vi "ArgosUltimateEditionV2.vi"(0 "PID 1 COM":refnum<visa-resource-name>="COM24", 1 "Setpoint\n START":bool, 2 "Write to File":bool, 3 "SP 1 input (°C)":dbl=10.0 min=0.0 max=1300.0, 4 "Intervall (s)":u32=1 max=600, 5 "Write/\nRead":bool=TRUE, 6 "Delay (ms)":u32=500 min=100 max=600000, 7 "Auto Tune":bool, 9 "Standby":bool, 11 "Reset\nSTOP":bool, 12 "ON":bool=TRUE caption="OFF", 13 "Get Values":bool, 15 "File Path":path) -> (8 "(°C)":dbl format="%#.3f", 14 "SP 1 is (°C)":dbl)   [LabVIEW 2013]
doc: "1. Verwendung\n\nDas Programm dient der Steuerung und Abfrage des Thermocontrollers I3252 und dem Auslesen von zwei VC 840 Messgeräten und einem Druckmessgerät Pfeiffer Single Gauge. \nDie Messgeräte werden Standardmäßig ausgelesen und erst nach Betätigung des Schalters \"Write to File\" in einer Textdatei abgespeichert. Das Eingabefeld \"Intervall\" legt den Abstand der Messpunkte fest.\nDer Setpoint für den Thermocontroller wird erst nach Betätigung des Tasters \"Setpoint START\" übernommen und angesteuert. Er wird ind den EEPROM des Gerätes geschrieben. Die Regelung kann mit Hilfe des Schalters \"Standby\" unterbrochen werden. Durch den Taster \"Reset STOPP\" kann der Setpoint aus dem EEPROM gelöscht werden.\nDie Eingabeflächen \"Constant\" und \"Thickness\" dienen der Berechnung des spezifischen Widerstands.\nDie Eingabeflächen \"User\" und \"Sample\" werden in den Header der Textdatei übernommen.\nDer Indikator \"File Path\" zeigt den aktuellen Speicherort der Textdatei an. Dieser wird nach ausschalten des Schalters \"Write to File\" gelöscht. Bei erneuten Schreiben muss ein neuer Speicherort gewählt werden. Bei Wahl desselben Speicherorts werden sämtliche bereits gespeicherte Daten gelöscht.\n\n\n2. Erläuterungen zum Blockdiagramm\n2.1 äußere Sequenz\nDie äußerte Sequenz besteht aus fünf Frames. Der erste dient der Initialisierung der Ports. Der zweite dient als Verzögerung um dem Programm genug Zeit zu geben die Ports zu öffnen. Jedoch senden die beiden VC 840 bereits Informationen an den Computer die in einem Puffer zwischengespeichert werden. Im dritten Frame wird dieser Puffer geleert. Somit kommt es zu keinem Framing Error. Desweiteren wird in diesem Frame die Startzeit der Messungen genommen. Im vierten Frame wird die eigentliche Messung und Verarbeitung der Daten durchgeführt. Die while-Schleife wird nur durch Auftreten eines Fehlers oder durch Betätigung des Stopbuttons auf dem Front Panel in der oberen linken Ecke unterbrochen. Im fünften und letzten Frame werden die Ports wieder geschlossen und beim Auftreten eines Fehlers wird das Programm automatisch gestoppt. Falls kein Fehler auftritt wird die Sequenz von vorne abgearbeitet.\n\n2.2 while-Schleife und innere Sequenz\n2.2.1 \"Event Structure\"\n2.2.1.1 Allgemein\nDer erste Frame beinhaltet ein \"Event Structure\". Dieser reagiert auf insgesamt elf verschiedene Ereignisse. Falls keines dieser Ereignisse auftreten sollte, warte die Struktur eine Millisekunde bevor die \"Event Structure\" verlassen wird. Die übrigen Ereignisse treten ein, wenn der entsprechende Kontroller eine Werteänderung erfährt.\n\n2.2.1.2 Event: Setpoint\nDieser Case besteht von außen nach innen aus einer Stacked Sequence, einer for-Loop und einer Flat Sequence die wiederum zwei \"Case Structures\" enthält. Als erstes wird bei dem Schalter \"Setpoint START\" der Blinkmodus aktiviert und bei dem Schalter \"Read Temperature\" deaktiviert. Danach folgt das eigentliche setzen des Temperatursollwerts. In der ersten Iteration wird dem Controller I3252 ein Schreibbefehl gesendet. Theoretisch kann der Setpoint in den RAM oder in den EEPROM geschrieben werden. Diese Auswahl erfolgt mit Hilfe des Schalters \"RAM\". Da das Schreiben in den RAM -Speicher aber aus diversen Gründen nicht erwünscht ist, wurde es nicht implementiert. Eine nachträgliche Implementierung ist aber leicht möglich, in dem die untere String-Konstante \"*P012\" durch \"*W012\" ersetzt wird. An diesem Befehl wird eine fünfstellige Hexadezimalzahl angehängt, die den Sollwert wiedergibt. Der Sollwert wird vorher mit zehn multipliziert, da das Komma standardmäßig nach der ersten Ziffer festgesetzt wurde (Bsp.: 800 wird gesendet um 80 einzustellen). Dieser Befehlsstrang wird an das Gerät mittels des SubVIs \"Comm_Interface\", auf welches später noch näher eingegangen wird, weitergegeben. Der durch das Gerät zurückgegebene String wird nicht verarbeitet.\nDie zweite Iteration dient dem Auslesen des eingestellten Sollwertes. Wahlweise kann der RAM- oder der EEPROM-Speicher ausgelesen werden. Die eigentliche Verarbeitung des Ausgabestrings erfolgt durch das SubVI \"Edit Setpoint\".\nDie Implementierung zur Einstellung des zweiten Setpoints erfolgt durch kopieren der ersten beiden Fälle und ersetzen der \"1\" im Befehf durch eine \"2\" (Bsp.: \"*P012\" zu \"*P022\"). Es darf aber nicht vergessen werden, dass dann ebenfalls die Anzahl der Iterationen angepasst werden muss.\nAls letztes wird der Blinkmodus des Schalters \"Setpoint START\" wieder deaktiviert.\n\n2.2.1.3 Event: Standby\nDieses Ereignis aktiviert bzw. deaktiviert als erstes den Blinckmodus des entsprechenden Schalters und sendet danach den Befehl zum aktivieren (\"*D03\") oder zum deaktivieren (\"*E03\") des Standbymodus an den Thermocontroller.\n\n2.2.1.4 Event: Set Command \nDer in das Feld \"Command shall be\" eingegebene Befehl wird an den Thermocontroller übermittlet. Die korrekte Form des Befehls ist im \"Communication Manuel\" nachzuschlagen. Das \"*\"-Zeichen wurde allerdings schon implementiert und muss somit nicht mit eingegeben werden.\n\n2.2.1.5 Event: Reset\nIn der ersten Iteration wird der Reset-Befehl an den Thermocontroller gesendet. In Folge wird der gesamte EEPROM-Speicher gelöscht. Deshalb wird in der zweiten Iteration der Setpoint aktualisiert. Dieser Befehl hat keinen Einfluss auf den RAM-Speicher. Die anschließende Wartezeit ist auf vier Sekunden festgesetzt und wurde empirisch ermittelt. Diese Zeit benötigt das Gerät um den Reset durchzuführen und für die Kommunikation wieder zur Verfügung zu stehen.\n\n2.2.1.6 Event: Auto Tune\nEs ist festgeschrieben, dass der Setpoint für die \"Auto Tune\"-Funktion wenigstens 20°C über der aktuellen Temperatur liegt. Deshalb wird zunächst der aktuelle Temperaturwert ausgelesen. Im zweiten Schritt werden zu diesem Wert zwanzig addiert und der Setpoint wird in den RAM-Speicher geschrieben. Das Schreiben in diesen Speicher ist nötig, da die \"Auto Tune\"-Funktion\" erst nach einem Reset startet. Im dritten Schritt wird der eigentliche Befehl für den \"Auto Tune\" gesendet (siehe dazu \"Communication Manuel\" S.27). Als vierte und letzte Iteration der for-Schleife folgt der bereits erwähnte Reset-Befehl. Der Temperatursollwert, der im RAM-Speicher eingetragen ist, muss zum Schluss wieder auf 0°C gesetzt werden. Die Zeit für die Ausführung des \"Auto Tune\"-Befehls wurde empirisch ermittelt und 45 s festgesetzt.\n\n2.2.1.7 Event: Write LOW/HI\nDieses Ereignis setzt die am Analogausgang anliegende Spannung fest. Normalerweise beträgt dieser Spannungswert 0-10 V. Das angeschlossene Netzteil verträgt aber maximal nur 2,3 V. Aus diesem Grund wird der \"%HIGH\" auf 23 gesetzt. Somit beträgt die maximal anliegende Spannung nur noch 23% von der maximal möglichen, d.h 2,3V. Ein niedrigerer Wert ist jederzeit möglich, genauso wie ein höherer für den Parameter \"%LOW\". Diese werden zunächst nacheinander in den RAM-Speicher geschrieben und anschließend wieder ausgelesen.\n\n2.2.1.8 Event: Set PID\nDie Werte für den PID-Regler können sowohl mit Hilfe der \"Auto Tune\"-Funktion, als auch manuell eingestellt werden. Es wird wiederum zwischen dem Schreiben in den RAM- und dem EEPROM-Speicher unterschieden. Zunächst werden die Werte für \"P\", \"I\" und \"D\", in dieser Reihenfolge, gesetzt und danach die aktuellen Werte ausgelesen.\n\n2.2.1.9 Event: Get Values\nDieses Ereignis hat zur Folge, dass die Werte für \"P\", \"I\", \"D\", \"%LOW\", \"%HIGH\" und des Setpoints wahlweise aus dem RAM- oder EEPROM-Speicher gelesen werden. Die aktuellen Werte werden nicht nur in die entsprechenden Anzeigefelder übernommen, sondern auch in die entsprechenden Eingabefelder, mit Ausnahme des Temperatursollwerts. \n\n2.2.1.10 Event: RAM\nPrinzipiell kann zwischen dem Schreiben in den RAM- oder EEPROM-Speicher des Thermocontrollers gewählt werden. Die entsprechende Schalterposition auf dem Frontpanel zeigt den aktuell verwendeten Speicher an. Die Anzeigewerte werden bei jedem Umschalten aktualisiert und sind im entsprechenden Speicher eingetragen. Die Implementierung ist identisch mit der des Ereignisses \"Get Values\". Es gilt zu beachten, dass die Werte für \"%LOW\" und \"%HIGH\" nur in den RAM-Speicher geschrieben werden können und somit auch nur aus diesem ausgelesen werden können.\n\n2.2.1.11 Event: Set Gauge to Zero\nMit Hilfe der SubVIs \"Get Pressure\" und \"Offset Display\" werden die Werte für den alten und den neuen Offset und der durch den zweiten Drucksensor ermittelt Druck ermittelt. \n\n2.2.1.12 Event: Write to File\nSollte der Schalter \"Write to File\" aktiviert werden, d.h. Schalterposition oben, so wird zunächst durch das SubVI \"Header\" ein Header für die unter \"File Path\" definierte Datei angelegt. Alle Werte, die bereits in der entsprechenden Datei stehen, werden dabei gelöscht.\n\n2.2.2 \"Timed Structures\"\nIm dritten Frame der inneren Sequenz werden die Werte für Zeitpunkt, Temperatur, Spannung, Strom und Druck ermittelt. Damit die Werte zum gleichen Zeitpunkt aufgenommen werden, werden \"Timed Sequences\" eingesetzt. Mit dem entsprechenden Schalter auf dem Front Panel unter dem Tab \"Settings\" kann gewählt werden, ob das entsprechende Gerät ausgelesen werden soll oder nicht. Die einzelnen Sequenzen werden parallel abgearbeitet, womit die Prozesszeit von diesem Frame durch der zeitintensivsten Sequenz abhängt. Dies ist in aller Regel das Auslesen der Temperatur, da ein \"Delay\" von 500 ms oder größer benötigt wird, um den Controller ordentlich ansprechen zu können.\nDie Systemzeit wird durch das SubVI \"System Time in Seconds\" in Sekunden umgerechnet und der in dem Parameter \"Starttime\" gespeicherte Wert wird abgezogen. Somit werden die Sekunden seit dem Start des Programms gezählt.\n\n2.2.3 restlichen Frames\nIm zweiten Frame wird das Intervall zwischen den einzelnen Messwerten festgelegt. Dabei wird der Wert des Parameters \"Delay\" abgezogen. Dieser Wert beträgt im Normalfall 500 ms und ist somit nicht vernachlääsigbar.\nDer Vierte Frame beinhaltet die Umrechnung des Temperatur-Strings in einen Temperaturwert durch das SubVI \"Edit Tmperature\", die Berechnung des spezifischen Widerstands durch das SubVI \"Resistivity Calculation\" und die Überprüfung des Druckwerts. Auch werden die neu gewonnen Werte in das entsprechende Shift-Register übernommen. Falls der Druckwert einen in dem Parameter \"Pressure Limit (mbar)\" festgelegten Grenzwert überschreiten sollte, wird der Thermocontroller automatisch in den Standby-Modus versetzt. Des Weiteren wird der Schalter \"Standby\" solange gesperrt, wie der Druck oberhalb des Grenzwertes liegt. Wenn der Druck wieder unter den Grenzwert gesunken ist, wird der Standby-Befehl nicht automatisch aufgehoben, sondern muss vom Benutzer durch Betätigung des entsprechenden Schalters gegeben werden.\nIm fünften Frame werden die Diagramme erstellt. Dabei wird jedes Mal von neuem das gesamte Shift-Register als Graph dargestellt. Weiterhin werden die Messwerte in ein 1D-Array geschrieben.\nDer sechste und letzte Frame beinhaltet den eigentlich Schreibvorgang der Messwerte in eine Textdatei und die Überprüfung ob ein Fehler vorliegt.\n\n2.3 SubVIs\n2.3.1 Allgemein\nDie SubVIs für die Messgeräte VC840 und das Druckmessgerät wurden aus anderen Quellen übernommen. \n\n2.3.2 \"Header\"\nIn den Header wird zunächst das aktuelle Datum und die aktuelle Zeit übernommen. Die ausgewählte Datei wird dabei überschrieben. Danach wird der Name des Benutzers und der Probe übernommen. Zum Schluss werden die Einheiten in einer Reihe, durch einen Tabulator getrennt, in den Header geschrieben.\n\n2.3.3 \"I3252 Comm Interface\"\nDieses VI stellt die Kommunikation mit dem Thermocontroller her und gibt den Ausgabe-String zurück.\n\n2.3.4 \"I3252 Edit Setpoint\"\nIm Ausgabe-String vom Thermocontroller ist an der vierten Stelle die Stelle des Dezimalpunktes verschlüsselt. Dieses Hexadezimalzahl wird herausgefiltert und an ein \"ENUM Controller\" übergeben. Dieser weist der Hexadezimalzahl eine Nummer zu, mit welcher ein Wert aus einem Array entnommen wird. Dieser Wert dient als Quotient. Der tatsächliche Wert kann somit errechnet werden.\n\n2.3.5 \"I3252 Edit Temperature\"\nDer Temperatur-String, der vom Thermocontroller zurückgegeben wird, wird in eine Dezimalzahl umgewandelt. Manchmal kommt es aus zu Dropouts, die durch dieses Programm herausgefiltert werden. Der letzte Wert wird dabei in einer \"Feedback Node\" gehalten unter der Annahme, dass sich der Temperaturwert nicht sprunghaft ändert.\n\n2.3.6 \"Resistivity Calculation\"\nDer spezifische Widerstand wird nach folgender Formel ausgerechnet. Dabei entspricht t der Dicke der Probe und C ist eine Konstante.\nrho=C*pi*t*U/(ln( 2)*I)\n\n2.3.7 \"System Time in Seconds\"\nZunächst wird die aktuelle Systemzeit ausgelesen. Danach wird diese in Stunden, Minuten und Sekunden aufgeteilt, alles in Sekunden umgerechnet und letztendlich addiert."
uses:
  <vilib>/Platform/TimedLoop/XDataNode/timing_clust.ctl
  <vilib>/Platform/TimedLoop/XDataNode/nitl_modes.ctl
  <vilib>/Platform/TimedLoop/XDataNode/wakeup.ctl
  <vilib>/Utility/config.llb/Read Key (String).vi
  <vilib>/Instr/_visa.llb/VISA Configure Serial Port (Instr).vi
  <vilib>/Platform/TimedLoop/scheduler/LVUserAPI/_suppVIs/Create_1kHz_TSource.vi
  <vilib>/Utility/file.llb/Write To Spreadsheet File (DBL).vi
  <vilib>/Platform/TimedLoop/XDataNode/XDataNode.xnode
  <vilib>/Platform/TimedLoop/XDataNode/XDNodeRunTimeDep.lvlib
  Dependencies/Pfeiffer TPG261+262 Single+Dual Gauge/Dual Gauge.lvlib
  <vilib>/Utility/config.llb/NI_LVConfig.lvlib
panel:
  out "appended array":dbl[](array[numeric])
  in  "Tab Control":T1(tab)
  in  "Temperature2":bool
  in  "Temprature1":bool
  out "TEMPERATURE":cluster{dbl[], dbl[]}[](graph)
  in  "OUTPUT":bool
  in  "SET":bool
  in  "Source \nCurrent":dbl=20.0
  in  "Unit":string(combo)="1"
  in  "Voltage\nCompl.":dbl=2.0
  in  "Unit   2":string(combo)="0"
  in  "4PP Const":dbl=1.0
  in  "Thickness":dbl=40.0
  out "Log Intervall (s)":dbl
  in  "Sample":string
  in  "User":string
  in  "SP 2 input (°C)":dbl=10.0 min=0.0 max=1300.0
  in  "Ramp 2":bool
  in  "RAMP\n\n 2":dbl
  in  "SOAK \n\n2":dbl
  in  "Ramp":bool
  in  "SOAK":dbl
  in  "RAMP":dbl
  out "SP 2 is (°C)":dbl
  in  "Standby\n2":bool
  in  "Setpoint\n START\n2":bool
  in  "Reset\nSTOP 2":bool
  in  "Baratron":bool
  out "Baratron":dbl format="%#_3e"
  in  "Manip":bool
  in  "VVP2":bool
  in  "VVP1":bool
  in  "Transf":bool
  in  "Main":bool
  out "Main Chamber":dbl format="%#.2e"
  out "VVP1":dbl format="%#.2e"
  out "Manipulator":dbl caption="current" format="%#.2e"
  out "LoadLock":dbl format="%#.2e"
  out "VVP2 2":dbl format="%#.2e"
  out "Pirani (VVP1 Scroll)":cluster{dbl[], dbl[]}[](graph)
  out "Current Time (s)":dbl
  out "Loop Time (s)":dbl
  out "CMR275 Baratron":cluster{dbl[], dbl[]}(graph)
  out "(°C) \n\n2":dbl format="%#.3f"
  in  "Set Gauge to Zero":bool
  out "Current Offset (mbar)":dbl caption="Offset"
  out "Resistivity Graph (Ohm Cm)":cluster{dbl[], dbl[]}(graph)
  out "Resistivity/ Temp Dependency":cluster{dbl[], dbl[]}(graph)
  out "Voltage Graph":cluster{dbl[], dbl[]}(graph)
  out "Current Graph":cluster{dbl[], dbl[]}(graph)
  out "Current (A) \n\n3":string
  out "Voltage  (V)\n 2":string
  out "Resistivity\n 2":dbl
  in  "Emissivity\n(eg: 0500)":dbl
  in  "Pyrometer":bool caption="ON\nOFF"
  out "Pyrometer Temperature °C":cluster{dbl[], dbl[]}(graph)
  out "Pyro Temp":dbl format="%.2f"
  in  "Thickness (nm)":dbl min=0.0
  in  "4PP constant":dbl min=0.0 max=5.0
  out "MM2":dbl format="%.4e"
  out "MM2":cluster{dbl[], dbl[]}(graph)
  out "MM1":cluster{dbl[], dbl[]}(graph)
  out "MM1":dbl format="%.4e"
  out "Resistivity":cluster{dbl[], dbl[]}(graph)
  out "Resistivity\n (Ohm*cm)":dbl format="%.3e"
  out "read buffer":string
  in  "Keithley COM Port":refnum<visa-resource-name>="COM6"
  in  "Pyro COM Port":refnum<visa-resource-name>="COM3"
  out "Pressure Gauge 2#2 2":dbl format="%.3e"
  out "Pressure Gauge 2#1 2":dbl format="%.3e"
  out "Status Gauge 2#2 2":i32(ring) items=["data OK", "underrange", "overrange", "sensor error", "sensor off", "no sensor", "ID error"]
  out "Status Gauge 2#1 2":i32(ring) items=["data OK", "underrange", "overrange", "sensor error", "sensor off", "no sensor", "ID error"]
  in  "TPG 2 COM 2":refnum<visa-resource-name>="COM22"
  in  "ON (TPG 3)":bool=TRUE caption="OFF"
  in  "ON (TPG 2)":bool=TRUE caption="OFF"
  out "Status Gauge 1#2":i32(ring) items=["data OK", "underrange", "overrange", "sensor error", "sensor off", "no sensor", "ID error"]
  out "Pressure Gauge 1#2":dbl format="%.3e"
  out "Pressure Gauge 1#1":dbl format="%.3e"
  out "Status Gauge 1#1":i32(ring) items=["data OK", "underrange", "overrange", "sensor error", "sensor off", "no sensor", "ID error"]
  in  "TPG 1 COM":refnum<visa-resource-name>="COM23"
  in  "ON (TPG 1)":bool=TRUE caption="OFF"
  in  "TPG 2 COM":refnum<visa-resource-name>="COM22"
  out "Pressure Gauge 2#2":dbl format="%.3e"
  out "Pressure Gauge 2#1":dbl format="%.3e"
  out "Status Gauge 2#2":i32(ring) items=["data OK", "underrange", "overrange", "sensor error", "sensor off", "no sensor", "ID error"]
  out "Status Gauge 2#1":i32(ring) items=["data OK", "underrange", "overrange", "sensor error", "sensor off", "no sensor", "ID error"]
  out "% HIGH Istwert 2":u32
  out "% LOW Istwert 2":u32
  in  "% High Sollwert 2":u32=23 max=24
  in  "% LOW Sollwert 2":u32 max=25
  in  "RAM 2":bool=TRUE caption="EEPROM"
  out "D (Rate) IstWert 2":u32
  out "I ( Reset1) Istwert 2":u32
  out "P (PB1) Istwert 2":u32 caption="actual value"
  in  "D (Rate) Sollwert 2":u32 max=3999
  in  "I ( Reset1) Sollwert 2":u32 max=3999
  in  "P (PB1) Sollwert 2":u32 caption="set value" max=9999
  in  "ON 2":bool=TRUE caption="OFF"
  in  "PID 2 COM":refnum<visa-resource-name>="COM25"
  in  "Delay (ms) 2":u32=500 min=100 max=600000
  in  "Write/\nRead \n\n2":bool=TRUE
  out "Command output 2":string
  in  "Command input 2":string
  in  "Set Command\n\n 2":bool
  in  "Auto Tune 2":bool
  in  "Set PID 2":bool
  in  "Write LOW/HI 2":bool
  in  "Get Values 2":bool
  in  "Pressure Limit (mbar)":dbl=1.0 min=0.0 max=1100.0
  in  "ON":bool caption="OFF"
  in  "VC 840 2":refnum<visa-resource-name>="COM8"
  out "Reading 2":dbl format="%_4f"
  out "Mode 2":enum16{"?", "Diode", "Beep", "DC", "AC"}(ring)
  out "Unit 2":string
  in  "VC 840 1":refnum<visa-resource-name>="COM1"
  out "Reading 1":dbl format="%_4f"
  out "Mode 1":enum16{"?", "Diode", "Beep", "DC", "AC"}(ring)
  out "Unit 1":string
  out "Status 1":T2
  out "Status 2":T2
  in  "ON":bool caption="OFF"
  out "% HIGH Istwert":u32
  out "% LOW Istwert":u32
  in  "% High Sollwert":u32=23 max=24
  in  "% LOW Sollwert":u32 max=25
  in  "RAM":bool=TRUE caption="EEPROM"
  out "D (Rate) IstWert":u32
  out "I ( Reset1) Istwert":u32
  out "P (PB1) Istwert":u32 caption="actual value"
  in  "D (Rate) Sollwert":u32 max=3999
  in  "I ( Reset1) Sollwert":u32 max=3999
  in  "P (PB1) Sollwert":u32 caption="set value" max=9999
  in  "Set Command":bool
  in  "Set PID":bool
  in  "Write LOW/HI":bool
  out "Command output":string
  in  "Command input":string
  in  "Get COM from Config":bool=TRUE
  # "mbar"
  # "PID Side B"
  # "PID Side A"
  # "T (°C)"
  # "T (°C)"
  # "Actual \n \n2"
  # "Actual"
  # "Pressure Measurement \n      (Pfeiffer TPG261)"
  # "PID Controller 2 (Omega Newport i3252)"
  # "P"
  # "I"
  # "D"
  # "% Low"
  # "% High"
  # "Multimeter\n#1 (VC 840)"
  # "Multimeter\n#2 (VC 840)"
  # "PID Controller (Omega Newport i3252)"
  # "P"
  # "I"
  # "D"
  # "% Low"
  # "% High"
  # "Authors:  Daniel Schuster (sir-dan@web.de)\n                 Steffen Cornelius (s.cornelius@hzdr.de)\n                 Nico Spahn (x)\n\n                 premade SubVIs for readout of Pfeiffer gauge and VC840 Multimeters were used\n                 SubVI \"I3252_Comm_Interface\" is based on a modified Labview example\n\nRelease:  v1.0    \n\nVersion History:\n\nv1.1  -    28.06.2011\n             - Format des Files geändert von %.3f auf %g\n             - maximale Eingabewerte für PID begrenzt\nv1.2  -    12.07.2011\n             - Anzeige p,rho, U, V auf Scientific geändert\n             - y-Achse p,rho auf Log geändert\n             - numerische Zeitanzeige hinzugefügt\n             - 4PP Constant: pi/ln(2)=4,532 set as the default value\nv1.3  -    25.07.2011\n             - Zeitvariable auf EXT geändert, um Sprünge in Diagrammen loszuwerden\nv1.4  -   27.07.2011\n             - ALLE Variablen auf DBL zurückgesetzt wegen Formatierungsproblem im File\n             - Zeitberechnung neu gemacht (Tick count differenzen) -> Zeitsprünge korrigiert ?\n             - Delay/Intervall überarbeitet\nv1.5  -   05.12.2012\n                - Austausch der alten Pfeifer SubvIs durch neue -> nun alle 4 Kanäle des DualGauge\n                                                                                                         Controllers gleichzeitig auslesbar\n                - neue Pfeiffer SubVIs verwendet in Druckwertauslesung und Offset Berechnung des Baratron\n                  Druckes (COM5 Sensor1)\n                - Neuarragement des GUI -> FullRange und Baratron neben Temperatur auf Haupseite zu sehen\n                                                                   Pirani und OpenPort auf Meas.2 zu sehen\n                                                                   Diagnose Seite umfasst nun auch Widerstandsdiagramm\n                - Änderungen der Settingseite -> nun alle 4 Drucksensoren mit aktuellem Messwert und Gerätestatus\n                                                                           zu sehen\n                - The readout of the PID-Temperature Controller and the VC840 Multimeters was not modified\nv1.73  -  18.10.2013\n                - Layout Änderungen\nv.1.8   -  19.01.2014\n                - Änderung Layout Settings Tab\n                - Trennung der beiden TPG Dual Gauge Controls\n                -"
  # "Version 1.73    - last change 18.10.2013"
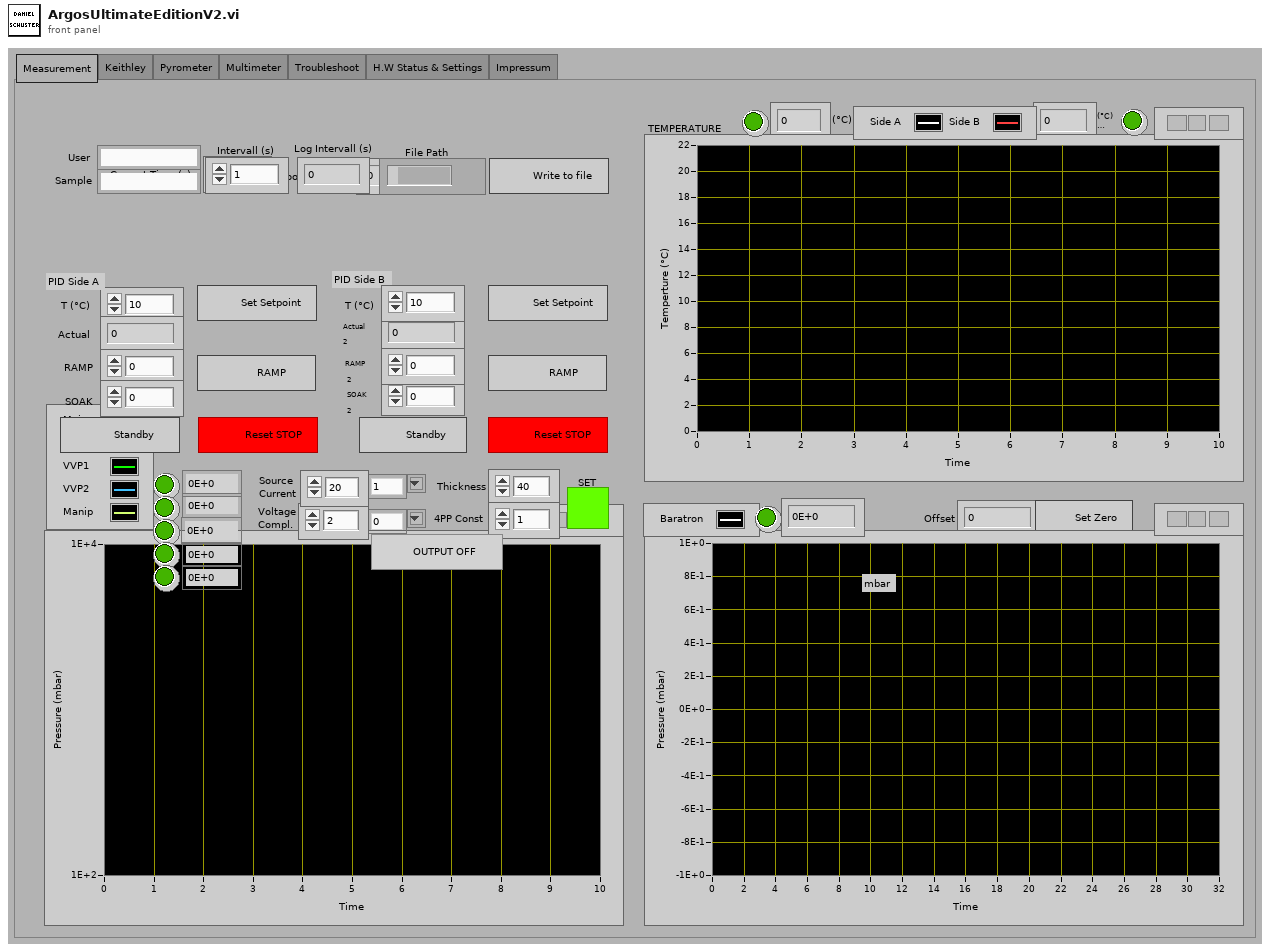
[diagram p1: front panel]
types:
  T1 = enum32{"Measurement", "Keithley", "Pyrometer", "Multimeter", "Troubleshoot", "H.W Status & Settings", "Impressum"}
  T2 = cluster{"Low Bat":bool, "Auto":bool, "Delta":bool, "Hold":bool, "RS232":bool}
  T3 = cluster{dbl[], dbl[], dbl[], dbl[], dbl[], dbl[]}
  T4 = typedef "XDNodeRunTimeDep.lvlib/timing_clust.ctl" = cluster{"Expected End [f-1]":u64, "Actual End [f-1]":u64, "Finished Late? [f-1]":bool, "Expected End [i-1]":u64, "Actual End [i-1]":u64, "Finished Late? [i-1]":bool, "Expected Start [i]":u64, "Actual Start [i]":u64, "Expected Start [f]":u64, "Actual Start [f]":u64, "Source Name":string, "Structure Name":string, "Period":i64, "Deadline":i64, "Offset":i64, "Start":i64, "Priority":i32, "Timeout":i32, "Mode":T5, "Wakeup Reason":T6, "Error":errorcluster, "Source Type":string, "Secondary Source Type":string, "Global End Time":u64, "Global Start Time":u64, "Frame Duration":u64, "Iteration Duration":u64, "Assigned CPU":i32, "I/O Scan Engine Mode":u32}
  T5 = typedef "XDNodeRunTimeDep.lvlib/nitl_modes.ctl" = enum32{"No Change", "Process missed periods, maintain original phase", "Discard missed periods, maintain original phase", "Process missed periods, ignore original phase", "Discard missed periods, ignore original phase"}
  T6 = typedef "XDNodeRunTimeDep.lvlib/wakeup.ctl" = enum32{"Normal", "Aborted", "Asynchronous wakeup", "Timing source error", "Timed loop error", "Timeout"}
  T7 = typedef "NI_LVConfig.lvlib/Config Data RefNum.ctl" = refnum<k1>
  T8 = enum8{"Enabled", "Disabled", "Disabled and Grayed Out"}
  T9 = cluster{"VISA resource name out":refnum<visa-resource-name>, "error out":errorcluster, "Delay (ms)":u32, "Write/\nRead":bool}
  T10 = cluster{"VISA resource name out":refnum<visa-resource-name>, "error out":errorcluster, "Delay (ms) 2":u32, "Write/\nRead \n\n2":bool}
  T11 = cluster{"TPG 2 COM":refnum<visa-resource-name>, "error out":errorcluster}
  T12 = cluster{"COM out":refnum<visa-resource-name>, "Cluster (Ausgang)":errorcluster}
  T13 = cluster{"Pressure Gauge#1":dbl, "Pressure Gauge#2":dbl}
  T14 = cluster{"TPG 1 COM":refnum<visa-resource-name>, "error out":errorcluster}
  T15 = cluster{"TPG 2 COM 2":refnum<visa-resource-name>, "error out":errorcluster}
  T16 = cluster{"COM out":refnum<visa-resource-name>, "error out":errorcluster, "COM out":refnum<visa-resource-name>, "error out":errorcluster}
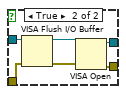
[diagram p10: hidden frame]
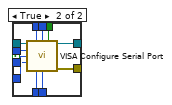
[diagram p12: hidden frame]
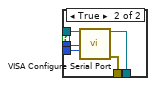
[diagram p14: hidden frame]
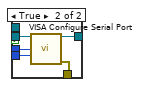
[diagram p15: hidden frame]
diagram:
  n1 = while {
    stop <- w52 stop-if-true
    n2 = flat-sequence {
      tunnel: [w97] -> w28
      tunnel: [w105] -> w27
      tunnel: [w104] -> w26
      tunnel: [w103] -> w25
      tunnel: [w102] -> w24
      tunnel: [w101] -> w23
      tunnel: [w100] -> w22
      tunnel: [w99] -> w21
      tunnel: [w92] -> w20
      tunnel: [w89] -> w15
      tunnel: [w88] -> w14
      tunnel: [w87] -> w13
      tunnel: [w86] -> w12
      tunnel: [w85] -> w11
      tunnel: [w84] -> w10
      tunnel: [w83] -> w7
      tunnel: [w82] -> w6
      tunnel: [w81] -> w1
      tunnel: [w200] -> w80
      tunnel: [w201] -> w79
      tunnel: [w193] -> w78
      tunnel: [w199] -> w77
      tunnel: [w198] -> w76
      tunnel: [w138] -> w75
      tunnel: [w137] -> w74
      tunnel: [errorcluster {"status"=FALSE, "code"=0, "source"=""} ("Fehler (Eingang)")] -> w49
      tunnel: [w187] -> w44
      tunnel: [w173] -> w39
      tunnel: [w172] -> w36
      tunnel: [w163] -> w32
      tunnel: [w162] -> w29
      tunnel: w28 -> [w161]
      tunnel: w27 -> [w159]
      tunnel: w26 -> [w156]
      tunnel: w25 -> [w155]
      tunnel: w24 -> [w152]
      tunnel: w23 -> [w151]
      tunnel: w22 -> [w148]
      tunnel: w21 -> [w146]
      tunnel: w20 -> [w143]
      tunnel: [w136] -> w18
      tunnel: w15 -> [w133]
      tunnel: w14 -> [w132]
      tunnel: w13 -> [w131]
      tunnel: w12 -> [w130]
      tunnel: w11 -> [w129]
      tunnel: w10 -> [w128]
      tunnel: [w127] -> w8
      tunnel: w7 -> [w127]
      tunnel: w6 -> [w126]
      tunnel: [w126] -> w5
      tunnel: [w125] -> w2
      tunnel: w1 -> [w125]
      tunnel: w80 -> [w280]
      tunnel: [w280] -> w73
      tunnel: w79 -> [w279]
      tunnel: [w279] -> w72
      tunnel: w78 -> [w278]
      tunnel: [w278] -> w71
      tunnel: w77 -> [w277]
      tunnel: [w277] -> w70
      tunnel: w76 -> [w276]
      tunnel: [w276] -> w69
      tunnel: [w274] -> w68
      tunnel: w75 -> [w274]
      tunnel: [w273] -> w67
      tunnel: w74 -> [w273]
      tunnel: [w272] -> w50
      tunnel: w49 -> [w272]
      tunnel: [w271] -> w45
      tunnel: w44 -> [w271]
      tunnel: [w270] -> w40
      tunnel: w39 -> [w270]
      tunnel: [w269] -> w37
      tunnel: w36 -> [w269]
      tunnel: [w268] -> w33
      tunnel: w32 -> [w268]
      tunnel: [w267] -> w30
      tunnel: w29 -> [w267]
      tunnel: [w266] -> w19
      tunnel: w18 -> [w266]
      tunnel: [w265] -> w9
      tunnel: w8 -> [w265]
      tunnel: w5 -> [w264]
      tunnel: [w264] -> w4
      tunnel: [w263] -> w3
      tunnel: w2 -> [w263]
      tunnel: w73 -> [w285]
      tunnel: [w285] -> w66
      tunnel: w72 -> [w284]
      tunnel: [w284] -> w65
      tunnel: w71 -> [w304]
      tunnel: [w304] -> w64
      tunnel: w70 -> [w287]
      tunnel: [w287] -> w63
      tunnel: w69 -> [w286]
      tunnel: [w286] -> w62
      tunnel: [w303] -> w61
      tunnel: [w301] -> w60
      tunnel: w68 -> [w302]
      tunnel: [w300] -> w59
      tunnel: w67 -> [w299]
      tunnel: w50 -> [w290]
      tunnel: [w298] -> w48
      tunnel: [w297] -> w47
      tunnel: [w296] -> w46
      tunnel: w45 -> [w296]
      tunnel: [w295] -> w41
      tunnel: w40 -> [w295]
      tunnel: [w294] -> w38
      tunnel: w37 -> [w294]
      tunnel: [w293] -> w34
      tunnel: w33 -> [w293]
      tunnel: [w292] -> w31
      tunnel: w30 -> [w292]
      tunnel: w19 -> [w291]
      tunnel: [w289] -> w17
      tunnel: [w288] -> w16
      tunnel: w9 -> [w283]
      tunnel: w4 -> [w282]
      tunnel: w3 -> [w281]
      tunnel: w66 -> [w358]
      tunnel: w65 -> [w357]
      tunnel: w64 -> [w356]
      tunnel: w63 -> [w354]
      tunnel: w62 -> [w353]
      tunnel: [w352] -> w58
      tunnel: [w351] -> w57
      tunnel: [w350] -> w56
      tunnel: [w349] -> w55
      tunnel: [w348] -> w54
      tunnel: [w347] -> w53
      tunnel: w61 -> [w341]
      tunnel: w60 -> [w340]
      tunnel: w59 -> [w339]
      tunnel: [w338] -> w52
      tunnel: [w337] -> w51
      tunnel: w48 -> [w336]
      tunnel: w47 -> [w335]
      tunnel: w46 -> [w334]
      tunnel: [w333] -> w43
      tunnel: [w332] -> w42
      tunnel: w41 -> [w330]
      tunnel: w38 -> [w329]
      tunnel: [w328] -> w35
      tunnel: w34 -> [w327]
      tunnel: w31 -> [w326]
      tunnel: w17 -> [w324]
      tunnel: w16 -> [w323]
      tunnel: w58 -> [w2653]
      tunnel: w57 -> [w2652]
      tunnel: w56 -> [w2655]
      tunnel: w55 -> [w2654]
      tunnel: w54 -> [w2657]
      tunnel: w53 -> [w2656]
      tunnel: w51 -> [w2650]
      tunnel: w43 -> [w2645]
      tunnel: w42 -> [w2644]
      tunnel: w35 -> [w2642]
      frame #0 {
        w93 = "PORTS"
        n3 = Current VI's Path() -> (path=w115:path)
        n4 = Strip Path(path=w115) -> ()  [unwired: 2 out]
        n5 = call <vilib>:"Application Directory.vi"() -> ("Application Directory"=w91:path)
        n6 = Build Path(base path=w91, name or relative path="Config.txt") -> (appended path=w113:path)
        n7 = call <vilib>:"Open Config Data.vi"("configuration file path"=w113) -> ("refnum"=w94:T7)  [unwired: 8 in, 2 out]
        n8 = call-poly <vilib>:"Read Key.vi"("section"=w93, "key"="DEFAULT", "refnum"=w94) -> ("value"=w95:string)  [unwired: 5 in, 3 out]
        n9 = call-poly <vilib>:"Read Key.vi"("section"=w93, "default value"=w95, "key"="Pyrometer", "refnum"=w94) -> ("value"=w99:string, "found?"=w84:bool)  [unwired: 4 in, 2 out]
        n10 = call-poly <vilib>:"Read Key.vi"("section"=w93, "default value"=w95, "key"="PID1", "refnum"=w94) -> ("value"=w97:string, "found?"=w89:bool)  [unwired: 4 in, 2 out]
        n11 = call-poly <vilib>:"Read Key.vi"("section"=w93, "default value"=w95, "key"="Keithley", "refnum"=w94) -> ("value"=w103:string, "found?"=w86:bool)  [unwired: 4 in, 2 out]
        n12 = call-poly <vilib>:"Read Key.vi"("section"=w93, "default value"=w95, "key"="Multimeter1", "refnum"=w94) -> ("value"=w104:string, "found?"=w87:bool)  [unwired: 4 in, 2 out]
        n13 = call-poly <vilib>:"Read Key.vi"("section"=w93, "default value"=w95, "key"="TPG2", "refnum"=w94) -> ("value"=w92:string, "found?"=w81:bool)  [unwired: 4 in, 2 out]
        n14 = call-poly <vilib>:"Read Key.vi"("section"=w93, "default value"=w95, "key"="PID2", "refnum"=w94) -> ("value"=w105:string, "found?"=w88:bool)  [unwired: 4 in, 2 out]
        n15 = case shown="False" w81 {
          frame False {
            n16 = property on="ON (TPG 3)" class="Bool (strict)"("Value"=FALSE ("ON")) -> ()  [unwired: 2 in, 2 out]
          }
          frame True {
          }
        }
        n17 = case shown="False" w84 {
          frame False {
            n18 = property on="Pyrometer" class="Bool (strict)"("Value"=FALSE ("ON")) -> ()  [unwired: 2 in, 2 out]
          }
          frame True {
          }
        }
        n19 = call-poly <vilib>:"Read Key.vi"("section"=w93, "default value"=w95, "key"="TPG2", "refnum"=w94) -> ("value"=w100:string, "found?"=w82:bool)  [unwired: 4 in, 2 out]
        n20 = case shown="False" w87 {
          frame False {
            n21 = property on="ON" class="Bool (strict)"("Value"=FALSE ("ON")) -> ()  [unwired: 2 in, 2 out]
          }
          frame True {
          }
        }
        n22 = call-poly <vilib>:"Read Key.vi"("section"=w93, "default value"=w95, "key"="Multimeter2", "refnum"=w94) -> ("value"=w102:string, "found?"=w85:bool)  [unwired: 4 in, 2 out]
        n23 = call-poly <vilib>:"Read Key.vi"("section"=w93, "default value"=w95, "key"="TPG1", "refnum"=w94) -> ("value"=w101:string, "found?"=w83:bool)  [unwired: 4 in, 2 out]
        n24 = case shown="False" w82 {
          frame False {
            n25 = property on="ON (TPG 2)" class="Bool (strict)"("Value"=FALSE ("ON")) -> ()  [unwired: 2 in, 2 out]
          }
          frame True {
          }
        }
        n26 = case shown="False" w88 {
          frame False {
            n27 = property on="ON 2" class="Bool (strict)"("Value"=FALSE ("ON")) -> ()  [unwired: 2 in, 2 out]
          }
          frame True {
          }
        }
        n28 = case shown="False" w85 {
          frame False {
            n29 = property on="ON" class="Bool (strict)"("Value"=FALSE ("ON")) -> ()  [unwired: 2 in, 2 out]
          }
          frame True {
          }
        }
        n30 = property on="Write to File" class="Bool (strict)"("Value"=FALSE ("Write to File")) -> ()  [unwired: 2 in, 2 out]
        n31 = case shown="False" w83 {
          frame False {
            n32 = property on="ON (TPG 1)" class="Bool (strict)"("Value"=FALSE ("ON")) -> ()  [unwired: 2 in, 2 out]
          }
          frame True {
          }
        }
        n33 = case shown="False" w89 {
          frame False {
            n34 = property on="ON" class="Bool (strict)"("Value"=FALSE ("ON")) -> ()  [unwired: 2 in, 2 out]
          }
          frame True {
          }
        }
      }
      frame #1 {
        w164 = u16 0 items=["None", "XON/XOFF", "RTS/CTS", "XON/XOFF & RTS/CTS", "DTR/DSR", "XON/XOFF & DTR/DSR"] ("flow control (0:none)")
        w165 = u16 10 items=["1.0"=10, "1.5"=15, "2.0"=20] ("stop bits (10: 1 bit)")
        w179 = u16 10 items=["1.0"=10, "1.5"=15, "2.0"=20] ("stop bits (10: 1 bit)")
        w178 = u16 0 items=["None", "XON/XOFF", "RTS/CTS", "XON/XOFF & RTS/CTS", "DTR/DSR", "XON/XOFF & DTR/DSR"] ("flow control (0:none)")
        w185 = u16 7 ("data bits (8)")
        w184 = enum16{"None", "Odd", "Even", "Mark", "Space"}."Odd" ("parity (0:none)")
        w186 = T8."Disabled and Grayed Out" ("Disabled")
        # "Disabling Auto-tune Feature"
        # "Zuweisung für die parallele Auslesung\nder DualGauge Ports"
        n35 = case shown="False" "Get COM from Config" {
          tunnel: w146 -> [_ w248]
          tunnel: [w247 w248] -> w135
          tunnel: "Pyro COM Port" -> [w247 _]
          frame False {
          }
          frame True {
          }
        }
        n36 = case shown="True" "Get COM from Config" {
          tunnel: w155 -> [_ w256]
          tunnel: [w255 w256] -> w140
          tunnel: "Keithley COM Port" -> [w255 _]
          frame False {
          }
          frame True {
          }
        }
        n37 = case shown="False" "Get COM from Config" {
          tunnel: w151 -> [_ w252]
          tunnel: [w251 w252] -> w138
          tunnel: "TPG 1 COM" -> [w251 _]
          frame False {
          }
          frame True {
          }
        }
        n38 = case shown="True" "Get COM from Config" {
          tunnel: w156 -> [_ w258]
          tunnel: [w257 w258] -> w142
          tunnel: "VC 840 1" -> [w257 _]
          frame False {
          }
          frame True {
          }
        }
        n39 = property on="TPG 1 COM" class="VISAName"("Value"=w138) -> ()  [unwired: 2 in, 2 out]
        n40 = case shown="False" "Get COM from Config" {
          tunnel: w152 -> [_ w254]
          tunnel: [w253 w254] -> w139
          tunnel: "VC 840 2" -> [w253 _]
          frame False {
          }
          frame True {
          }
        }
        n41 = property on="Pyro COM Port" class="VISAName"("Value"=w135) -> ()  [unwired: 2 in, 2 out]
        n42 = case shown="True" "Get COM from Config" {
          tunnel: w148 -> [_ w250]
          tunnel: [w249 w250] -> w137
          tunnel: "TPG 2 COM" -> [w249 _]
          frame False {
          }
          frame True {
          }
        }
        n43 = property on="TPG 2 COM" class="VISAName"("Value"=w137) -> ()  [unwired: 2 in, 2 out]
        n44 = case shown="False" "Get COM from Config" {
          tunnel: w159 -> [_ w260]
          tunnel: [w259 w260] -> w141
          tunnel: "PID 2 COM" -> [w259 _]
          frame False {
          }
          frame True {
          }
        }
        n45 = case shown="True" "Get COM from Config" {
          tunnel: w161 -> [_ w262]
          tunnel: [w261 w262] -> w134
          tunnel: "PID 1 COM" -> [w261 _]
          frame False {
          }
          frame True {
          }
        }
        n46 = property on="Keithley COM Port" class="VISAName"("Value"=w140) -> ()  [unwired: 2 in, 2 out]
        n47 = property on="VC 840 1" class="VISAName"("Value"=w142) -> ()  [unwired: 2 in, 2 out]
        n48 = case shown="False" "Get COM from Config" {
          tunnel: w143 -> [_ w246]
          tunnel: [w245 w246] -> w136
          tunnel: "TPG 2 COM 2" -> [w245 _]
          frame False {
          }
          frame True {
          }
        }
        n49 = case shown="True" w131 {
          tunnel: [_ w228] -> w201
          tunnel: [w227 w229] -> w200
          tunnel: w142 -> [w227 w232]
          frame False {
          }
          frame True {
            n50 = call "VC840_Open.vi"("VISA resource name"=w232) -> ("error out"=w230:errorcluster, "VISA resource name out"=w231:refnum<visa-resource-name>)  [unwired: 1 in, 8 out]
            n51 = VISA Flush I/O Buffer(VISA resource name=w231, error in (no error)=w230) -> (VISA resource name out=w229:refnum<visa-resource-name>, error out=w228:errorcluster)  [unwired: 1 in]
          }
        }
        n52 = case shown="True" w129 {
          tunnel: [w209 w211] -> w199
          tunnel: [_ w210] -> w198
          tunnel: w139 -> [w209 w214]
          frame False {
          }
          frame True {
            n53 = call "VC840_Open.vi"("VISA resource name"=w214) -> ("error out"=w212:errorcluster, "VISA resource name out"=w213:refnum<visa-resource-name>)  [unwired: 1 in, 8 out]
            n54 = VISA Flush I/O Buffer(VISA resource name=w213, error in (no error)=w212) -> (VISA resource name out=w211:refnum<visa-resource-name>, error out=w210:errorcluster)  [unwired: 1 in]
          }
        }
        n55 = property on="VC 840 2" class="VISAName"("Value"=w139) -> ()  [unwired: 2 in, 2 out]
        n56 = call-poly "VISA Configure Serial Port"("VISA resource name"=w135, "timeout (10sec)"=u32 10000, "termination char\n(0xA = '\\n' = LF)"=u8 10 ("termination char\n(0xA = '\\n' = LF)"), "Enable Termination\nChar (T)"=TRUE ("Enable Termination\nChar (T)"), "baud rate (9600)"=u32 19200, "data bits (8)"=u16 8, "parity (0:none)"=enum16{"None", "Odd", "Even", "Mark", "Space"}."Even", "stop bits (10: 1 bit)"=w179, "flow control (0:none)"=w178) -> ("VISA resource name out"=w183:refnum<visa-resource-name>, "error out"=w174:errorcluster)  [unwired: 5 in]
        n57 = property on="Auto Tune 2" class="Bool"("DisabledEnum"=w186) -> ()  [unwired: 2 in, 2 out]
        n58 = property on="Auto Tune" class="Bool"("DisabledEnum"=w186) -> ()  [unwired: 2 in, 2 out]
        n59 = case shown="False" w133 {
          tunnel: [_ w244] -> w197
          tunnel: [w239 w243] -> w196
          tunnel: w185 -> [_ w242]
          tunnel: w184 -> [_ w241]
          tunnel: w134 -> [_ w240]
          tunnel: w134 -> [w239 _]
          frame False {
          }
          frame True {
            n60 = call-poly "VISA Configure Serial Port"("VISA resource name"=w240, "data bits (8)"=w242, "parity (0:none)"=w241) -> ("VISA resource name out"=w243:refnum<visa-resource-name>, "error out"=w244:errorcluster)  [unwired: 6 in, 5 out]
          }
        }
        n61 = case shown="False" w132 {
          tunnel: [_ w238] -> w191
          tunnel: [w233 w237] -> w190
          tunnel: w185 -> [_ w236]
          tunnel: w184 -> [_ w235]
          tunnel: w141 -> [w233 w234]
          frame False {
          }
          frame True {
            n62 = call-poly "VISA Configure Serial Port"("VISA resource name"=w234, "data bits (8)"=w236, "parity (0:none)"=w235) -> ("VISA resource name out"=w237:refnum<visa-resource-name>, "error out"=w238:errorcluster)  [unwired: 6 in, 5 out]
          }
        }
        n63 = property on="PID 2 COM" class="VISAName"("Value"=w141) -> ()  [unwired: 2 in, 2 out]
        n64 = property on="PID 1 COM" class="VISAName"("Value"=w134) -> ()  [unwired: 2 in, 2 out]
        n65 = case shown="False" w130 {
          tunnel: u32 9600 ("baud rate (9600)") -> [_ w226]
          tunnel: u16 8 ("data bits (8)") -> [_ w225]
          tunnel: enum16{"None", "Odd", "Even", "Mark", "Space"}."None" ("parity (0:none)") -> [_ w224]
          tunnel: u32 10000 ("timeout (10sec)") -> [_ w223]
          tunnel: TRUE ("Enable Termination\nChar (T)") -> [_ w222]
          tunnel: u8 10 ("termination char\n(0xA = '\\n' = LF)") -> [_ w221]
          tunnel: w165 -> [_ w220]
          tunnel: w164 -> [_ w219]
          tunnel: [w215 w218] -> w163
          tunnel: [_ w217] -> w162
          tunnel: w140 -> [w215 w216]
          frame False {
          }
          frame True {
            n66 = call-poly "VISA Configure Serial Port"("VISA resource name"=w216, "timeout (10sec)"=w223, "termination char\n(0xA = '\\n' = LF)"=w221, "Enable Termination\nChar (T)"=w222, "baud rate (9600)"=w226, "data bits (8)"=w225, "parity (0:none)"=w224, "stop bits (10: 1 bit)"=w220, "flow control (0:none)"=w219) -> ("VISA resource name out"=w218:refnum<visa-resource-name>, "error out"=w217:errorcluster)  [unwired: 5 in]
          }
        }
        n67 = case shown="False" w128 {
          tunnel: w183 -> [w202 w207]
          tunnel: w174 -> [_ w206]
          tunnel: [w202 w204] -> w173
          tunnel: [_ w203] -> w172
          frame False {
          }
          frame True {
            n68 = VISA Flush I/O Buffer(VISA resource name=w207, error in (no error)=w206) -> (VISA resource name out=w208:refnum<visa-resource-name>, error out=w205:errorcluster)  [unwired: 1 in]
            n69 = VISA Open(error in (no error)=w205, VISA resource name=w208) -> (VISA resource name=w204:refnum<visa-resource-name>, error out=w203:errorcluster)  [unwired: 3 in]
          }
        }
        n70 = property on="TPG 2 COM 2" class="VISAName"("Value"=w136) -> ()  [unwired: 2 in, 2 out]
        n71 = Bundle("VISA resource name out"=w196, "error out"=w197, "Delay (ms)"="Delay (ms)", "Write/\nRead"="Write/\nRead") -> (w193:T9)  [unwired: 1 in]
        n72 = Bundle("VISA resource name out"=w190, "error out"=w191, "Delay (ms) 2"="Delay (ms) 2", "Write/\nRead \n\n2"="Write/\nRead \n\n2") -> (w187:T10)  [unwired: 1 in]
      }
      frame #2 {
        n73 = Wait (ms)(milliseconds to wait=u32 50) -> ()  [unwired: 1 out]
      }
      frame #3 {
        n74 = case shown="False" w282 {
          tunnel: [w312 w316] -> w300
          tunnel: w299 -> [w312 w315]
          tunnel: [w311 w314] -> w297
          tunnel: w290 -> [w311 w313]
          frame False {
          }
          frame True {
            n75 = VISA Flush I/O Buffer(VISA resource name=w315, error in (no error)=w313) -> (VISA resource name out=w316:refnum<visa-resource-name>, error out=w314:errorcluster)  [unwired: 1 in]
          }
        }
        n76 = case shown="False" w283 {
          tunnel: w302 -> [w318 w322]
          tunnel: [w318 w321] -> w301
          tunnel: [w317 w320] -> w298
          tunnel: w290 -> [w317 w319]
          frame False {
          }
          frame True {
            n77 = VISA Flush I/O Buffer(VISA resource name=w322, error in (no error)=w319) -> (VISA resource name out=w321:refnum<visa-resource-name>, error out=w320:errorcluster)  [unwired: 1 in]
          }
        }
        n78 = case shown="False" w281 {
          tunnel: w291 -> [w305 w310]
          tunnel: w290 -> [w306 w309]
          tunnel: [w305 w308] -> w289
          tunnel: [w306 w307] -> w288
          frame False {
          }
          frame True {
            n79 = VISA Flush I/O Buffer(VISA resource name=w310, error in (no error)=w309) -> (VISA resource name out=w308:refnum<visa-resource-name>, error out=w307:errorcluster)  [unwired: 1 in]
          }
        }
        n80 = Tick Count (ms)() -> (millisecond timer value=w303:u32)
      }
      frame #4 {
        n81 = call-poly <vilib>:"Create Timing Source.vi"() -> ("name (out)"=w355:string)  [unwired: 10 in, 1 out]
        n82 = while {
          tunnel: w358 -> [w627]
          tunnel: w357 -> [w626]
          tunnel: w356 -> [w625]
          tunnel: w355 -> [w618]
          tunnel: w354 -> [w611]
          tunnel: w353 -> [w610]
          tunnel: [w606] -> w352
          tunnel: [w605] -> w351
          tunnel: [w603] -> w350
          tunnel: [w601] -> w349
          tunnel: [w599] -> w348
          tunnel: [w597] -> w347
          shift-right: [w571] -> _
          shift-left: dbl[] [] -> [w576]
          shift-right: [w550] -> _
          shift-left: dbl[] [] -> [w584]
          shift-right: [w573] -> _
          shift-left: dbl[] [] -> [w580]
          shift-right: [w547] -> _
          shift-left: dbl[] [] -> [w583]
          shift-right: [w544] -> _
          shift-left: dbl[] [] -> [w582]
          tunnel: w341 -> [w539]
          tunnel: w340 -> [w495]
          tunnel: w339 -> [w491]
          shift-right: [w473] -> _
          shift-left: T3 {[], [], [], [], [], []} -> [w481]
          tunnel: [w359] -> w338
          tunnel: [w469] -> w337
          tunnel: w336 -> [w465]
          tunnel: w335 -> [w463]
          tunnel: w334 -> [w447]
          shift-right: [w439] -> _
          shift-left: dbl[] [] -> [w437]
          tunnel: [w428] -> w333
          tunnel: [w422] -> w332
          tunnel: w330 -> [w416]
          tunnel: w329 -> [w412]
          tunnel: [w406] -> w328
          shift-right: [w402] -> _
          shift-left: _ -> [w400]
          tunnel: w327 -> [w393]
          tunnel: w326 -> [w391]
          tunnel: w324 -> [w376]
          tunnel: w323 -> [w372]
          stop <- w468 stop-if-true
          w359 = FALSE ("y")
          n83 = flat-sequence {
            tunnel: w539 -> [w643]
            tunnel: w576 -> [w644]
            tunnel: w580 -> [w645]
            tunnel: w582 -> [w646]
            tunnel: w583 -> [w647]
            tunnel: w584 -> [w648]
            tunnel: w610 -> [w649]
            tunnel: w611 -> [w650]
            tunnel: w625 -> [w651]
            tunnel: w626 -> [w652]
            tunnel: w627 -> [w653]
            tunnel: [w653] -> w538
            tunnel: [w652] -> w537
            tunnel: [w651] -> w536
            tunnel: [w650] -> w535
            tunnel: [w649] -> w534
            tunnel: [w648] -> w533
            tunnel: [w647] -> w532
            tunnel: [w646] -> w531
            tunnel: [w645] -> w530
            tunnel: [w644] -> w529
            tunnel: [w643] -> w528
            tunnel: [w642] -> w510
            tunnel: [w641] -> w496
            tunnel: w495 -> [w641]
            tunnel: [w640] -> w492
            tunnel: w491 -> [w640]
            tunnel: [w639] -> w482
            tunnel: w481 -> [w639]
            tunnel: [w638] -> w466
            tunnel: w465 -> [w638]
            tunnel: [w637] -> w464
            tunnel: w463 -> [w637]
            tunnel: [w636] -> w448
            tunnel: w447 -> [w636]
            tunnel: [w635] -> w438
            tunnel: w437 -> [w635]
            tunnel: [w634] -> w417
            tunnel: w416 -> [w634]
            tunnel: [w633] -> w413
            tunnel: w412 -> [w633]
            tunnel: [w632] -> w401
            tunnel: w400 -> [w632]
            tunnel: [w631] -> w394
            tunnel: w393 -> [w631]
            tunnel: [w630] -> w392
            tunnel: w391 -> [w630]
            tunnel: [w629] -> w377
            tunnel: w376 -> [w629]
            tunnel: [w628] -> w373
            tunnel: w372 -> [w628]
            tunnel: [w685] -> w624
            tunnel: [w684] -> w622
            tunnel: [w680] -> w620
            tunnel: [w679] -> w615
            tunnel: [w678] -> w613
            tunnel: [w677] -> w581
            tunnel: [w676] -> w577
            tunnel: [w675] -> w558
            tunnel: [w674] -> w555
            tunnel: [w673] -> w553
            tunnel: [w672] -> w540
            tunnel: w538 -> [w685]
            tunnel: w537 -> [w684]
            tunnel: w536 -> [w683]
            tunnel: w535 -> [w679]
            tunnel: w534 -> [w678]
            tunnel: w533 -> [w675]
            tunnel: w532 -> [w674]
            tunnel: w531 -> [w673]
            tunnel: w530 -> [w677]
            tunnel: w529 -> [w676]
            tunnel: w528 -> [w672]
            tunnel: [w671] -> w511
            tunnel: w510 -> [w671]
            tunnel: w496 -> [w669]
            tunnel: [w669] -> w493
            tunnel: w492 -> [w670]
            tunnel: [w670] -> w489
            tunnel: w482 -> [w668]
            tunnel: [w668] -> w480
            tunnel: w466 -> [w667]
            tunnel: w464 -> [w666]
            tunnel: [w667] -> w461
            tunnel: [w666] -> w459
            tunnel: w448 -> [w662]
            tunnel: [w661] -> w445
            tunnel: w438 -> [w665]
            tunnel: [w665] -> w436
            tunnel: [w658] -> w418
            tunnel: w417 -> [w658]
            tunnel: [w660] -> w415
            tunnel: w413 -> [w660]
            tunnel: w401 -> [w659]
            tunnel: [w659] -> w397
            tunnel: w394 -> [w656]
            tunnel: w392 -> [w657]
            tunnel: [w656] -> w389
            tunnel: [w655] -> w378
            tunnel: w377 -> [w655]
            tunnel: [w654] -> w374
            tunnel: w373 -> [w654]
            tunnel: w624 -> [w1945]
            tunnel: [w1945] -> w623
            tunnel: w622 -> [w1944]
            tunnel: [w1944] -> w621
            tunnel: w620 -> [w1941]
            tunnel: [w1941] -> w619
            tunnel: w618 -> [w1926]
            tunnel: [w1926] -> w617
            tunnel: [w1926] -> w616
            tunnel: w615 -> [w1943]
            tunnel: [w1943] -> w614
            tunnel: w613 -> [w1942]
            tunnel: [w1942] -> w612
            tunnel: [w1926] -> w609
            tunnel: [w1926] -> w595
            tunnel: w581 -> [w1940]
            tunnel: [w1940] -> w579
            tunnel: w577 -> [w1939]
            tunnel: [w1939] -> w574
            tunnel: [w1938] -> w559
            tunnel: w558 -> [w1938]
            tunnel: [w1937] -> w556
            tunnel: w555 -> [w1937]
            tunnel: [w1936] -> w554
            tunnel: w553 -> [w1936]
            tunnel: [w1935] -> w541
            tunnel: w540 -> [w1935]
            tunnel: [w1934] -> w512
            tunnel: w511 -> [w1934]
            tunnel: [w1933] -> w494
            tunnel: w493 -> [w1933]
            tunnel: [w1932] -> w490
            tunnel: w489 -> [w1932]
            tunnel: w480 -> [w1931]
            tunnel: [w1931] -> w479
            tunnel: [w1930] -> w462
            tunnel: w461 -> [w1930]
            tunnel: [w1929] -> w460
            tunnel: w459 -> [w1929]
            tunnel: [w1928] -> w446
            tunnel: w445 -> [w1928]
            tunnel: w436 -> [w1927]
            tunnel: [w1927] -> w435
            tunnel: [w1926] -> w421
            tunnel: [w1925] -> w419
            tunnel: w418 -> [w1925]
            tunnel: w415 -> [w1924]
            tunnel: [w1924] -> w414
            tunnel: [w1923] -> w398
            tunnel: w397 -> [w1923]
            tunnel: [w1922] -> w390
            tunnel: w389 -> [w1922]
            tunnel: [w1921] -> w379
            tunnel: w378 -> [w1921]
            tunnel: [w1920] -> w375
            tunnel: w374 -> [w1920]
            tunnel: [w1993] -> w594
            tunnel: w623 -> [w2021]
            tunnel: w621 -> [w2020]
            tunnel: w619 -> [w2017]
            tunnel: w617 -> [w2016]
            tunnel: w616 -> [w2015]
            tunnel: w614 -> [w2005]
            tunnel: w612 -> [w2004]
            tunnel: w609 -> [w2006]
            tunnel: [w2002] -> w593
            tunnel: [w2003] -> w592
            tunnel: [w2014] -> w591
            tunnel: [w2013] -> w590
            tunnel: [w2012] -> w589
            tunnel: [w2011] -> w588
            tunnel: w595 -> [w1946]
            tunnel: [w2001] -> w587
            tunnel: [w2000] -> w586
            tunnel: [w1999] -> w585
            tunnel: w579 -> [w1998]
            tunnel: [w1998] -> w578
            tunnel: [w1997] -> w575
            tunnel: w574 -> [w1997]
            tunnel: w559 -> [w1996]
            tunnel: [w1996] -> w557
            tunnel: w556 -> [w1995]
            tunnel: w554 -> [w1994]
            tunnel: [w1995] -> w552
            tunnel: [w1994] -> w551
            tunnel: w541 -> [w1992]
            tunnel: [w1988] -> w513
            tunnel: w512 -> [w1988]
            tunnel: w494 -> [w1986]
            tunnel: w490 -> [w1985]
            tunnel: [w1983] -> w488
            tunnel: [w1947] -> w487
            tunnel: w479 -> [w1984]
            tunnel: [w1984] -> w478
            tunnel: [w1982] -> w470
            tunnel: w462 -> [w1981]
            tunnel: w460 -> [w1980]
            tunnel: [w1977] -> w455
            tunnel: [w1975] -> w454
            tunnel: [w1976] -> w451
            tunnel: w446 -> [w1972]
            tunnel: [w1971] -> w444
            tunnel: w435 -> [w1970]
            tunnel: [w1970] -> w434
            tunnel: [w1969] -> w432
            tunnel: [w1968] -> w423
            tunnel: w421 -> [w1967]
            tunnel: w419 -> [w1965]
            tunnel: w414 -> [w1964]
            tunnel: [w1963] -> w410
            tunnel: [w1962] -> w399
            tunnel: w398 -> [w1962]
            tunnel: [w1961] -> w396
            tunnel: w390 -> [w1960]
            tunnel: [w1958] -> w388
            tunnel: [w1957] -> w387
            tunnel: [w1956] -> w386
            tunnel: w379 -> [w1955]
            tunnel: w375 -> [w1954]
            tunnel: [w1952] -> w369
            tunnel: [w1951] -> w368
            tunnel: [w1950] -> w367
            tunnel: [w1947] -> w363
            tunnel: w594 -> [w2391]
            tunnel: [w2359] -> w569
            tunnel: w593 -> [w2402]
            tunnel: [w2402] -> w568
            tunnel: w592 -> [w2401]
            tunnel: [w2401] -> w567
            tunnel: w591 -> [w2400]
            tunnel: [w2400] -> w566
            tunnel: w590 -> [w2399]
            tunnel: [w2399] -> w565
            tunnel: w589 -> [w2398]
            tunnel: [w2398] -> w564
            tunnel: w588 -> [w2397]
            tunnel: [w2397] -> w563
            tunnel: w587 -> [w2386]
            tunnel: w586 -> [w2392]
            tunnel: w585 -> [w2360]
            tunnel: [w2391] -> w562
            tunnel: w578 -> [w2390]
            tunnel: w575 -> [w2389]
            tunnel: [w2388] -> w561
            tunnel: [w2379] -> w560
            tunnel: w557 -> [w2387]
            tunnel: w552 -> [w2384]
            tunnel: w551 -> [w2383]
            tunnel: [w2385] -> w548
            tunnel: [w2382] -> w545
            tunnel: [w2381] -> w542
            tunnel: [w2378] -> w514
            tunnel: w513 -> [w2378]
            tunnel: w488 -> [w2336]
            tunnel: w487 -> [w2337]
            tunnel: [w2357] -> w486
            tunnel: [w2356] -> w485
            tunnel: [w2355] -> w484
            tunnel: [w2354] -> w483
            tunnel: w478 -> [w2352]
            tunnel: [w2353] -> w477
            tunnel: [w2377] -> w471
            tunnel: w470 -> [w2377]
            tunnel: w455 -> [w2335]
            tunnel: w454 -> [w2334]
            tunnel: [w2376] -> w452
            tunnel: w451 -> [w2376]
            tunnel: w444 -> [w2361]
            tunnel: [w2375] -> w443
            tunnel: w434 -> [w2374]
            tunnel: [w2373] -> w433
            tunnel: w432 -> [w2373]
            tunnel: [w2372] -> w424
            tunnel: w423 -> [w2372]
            tunnel: [w2358] -> w420
            tunnel: [w2371] -> w411
            tunnel: w410 -> [w2371]
            tunnel: w399 -> [w2368]
            tunnel: w396 -> [w2330]
            tunnel: [w2370] -> w395
            tunnel: w388 -> [w2342]
            tunnel: w387 -> [w2341]
            tunnel: w386 -> [w2340]
            tunnel: [w2367] -> w384
            tunnel: [w2366] -> w382
            tunnel: [w2365] -> w380
            tunnel: [w2347] -> w370
            tunnel: w369 -> [w2347]
            tunnel: w368 -> [w2333]
            tunnel: w367 -> [w2332]
            tunnel: [w2344] -> w366
            tunnel: [w2343] -> w365
            tunnel: [w2339] -> w364
            tunnel: w363 -> [w2338]
            tunnel: [w2331] -> w362
            tunnel: [w2330] -> w361
            tunnel: [w2327] -> w360
            tunnel: w569 -> [w2481]
            tunnel: [w2505] -> w608
            tunnel: [w2504] -> w607
            tunnel: w568 -> [w2504]
            tunnel: [w2499] -> w604
            tunnel: w567 -> [w2499]
            tunnel: [w2503] -> w602
            tunnel: w566 -> [w2503]
            tunnel: [w2502] -> w600
            tunnel: w565 -> [w2502]
            tunnel: [w2501] -> w598
            tunnel: w564 -> [w2501]
            tunnel: [w2500] -> w596
            tunnel: w563 -> [w2500]
            tunnel: w562 -> [w2482]
            tunnel: w561 -> [w2470]
            tunnel: [w2470] -> w572
            tunnel: w560 -> [w2474]
            tunnel: [w2474] -> w570
            tunnel: [w2496] -> w549
            tunnel: w548 -> [w2496]
            tunnel: [w2497] -> w546
            tunnel: w545 -> [w2497]
            tunnel: [w2498] -> w543
            tunnel: w542 -> [w2498]
            tunnel: [w2495] -> w515
            tunnel: w514 -> [w2495]
            tunnel: w486 -> [w2494]
            tunnel: w485 -> [w2493]
            tunnel: w484 -> [w2492]
            tunnel: w483 -> [w2491]
            tunnel: w477 -> [w2490]
            tunnel: [w2490] -> w475
            tunnel: [w2489] -> w472
            tunnel: w471 -> [w2489]
            tunnel: [w2488] -> w453
            tunnel: w452 -> [w2488]
            tunnel: w443 -> [w2487]
            tunnel: [w2487] -> w440
            tunnel: w433 -> [w2486]
            tunnel: [w2486] -> w429
            tunnel: [w2485] -> w425
            tunnel: w424 -> [w2485]
            tunnel: w420 -> [w2480]
            tunnel: w411 -> [w2479]
            tunnel: [w2479] -> w408
            tunnel: [w2478] -> w403
            tunnel: w395 -> [w2478]
            tunnel: [w2477] -> w385
            tunnel: w384 -> [w2477]
            tunnel: [w2476] -> w383
            tunnel: w382 -> [w2476]
            tunnel: [w2475] -> w381
            tunnel: w380 -> [w2475]
            tunnel: [w2473] -> w371
            tunnel: w370 -> [w2473]
            tunnel: w366 -> [w2472]
            tunnel: w365 -> [w2471]
            tunnel: w364 -> [w2431]
            tunnel: w362 -> [w2430]
            tunnel: w361 -> [w2429]
            tunnel: w360 -> [w2428]
            tunnel: w608 -> [w2558]
            tunnel: w607 -> [w2572]
            tunnel: w604 -> [w2566]
            tunnel: w602 -> [w2571]
            tunnel: w600 -> [w2568]
            tunnel: w598 -> [w2570]
            tunnel: w596 -> [w2569]
            tunnel: w572 -> [w2563]
            tunnel: w570 -> [w2562]
            tunnel: w549 -> [w2561]
            tunnel: w546 -> [w2560]
            tunnel: w543 -> [w2559]
            tunnel: [w2555] -> w467
            tunnel: [w2572] -> w527
            tunnel: [w2566] -> w526
            tunnel: [w2571] -> w525
            tunnel: [w2568] -> w524
            tunnel: [w2570] -> w523
            tunnel: [w2569] -> w522
            tunnel: [w2563] -> w521
            tunnel: [w2562] -> w520
            tunnel: [w2561] -> w519
            tunnel: [w2560] -> w518
            tunnel: [w2559] -> w517
            tunnel: [w2557] -> w516
            tunnel: w515 -> [w2557]
            tunnel: [w2556] -> w476
            tunnel: w475 -> [w2556]
            tunnel: w472 -> [w2554]
            tunnel: [w2553] -> w458
            tunnel: [w2552] -> w457
            tunnel: w453 -> [w2551]
            tunnel: [w2550] -> w450
            tunnel: [w2549] -> w449
            tunnel: [w2548] -> w441
            tunnel: w440 -> [w2548]
            tunnel: [w2547] -> w430
            tunnel: w429 -> [w2547]
            tunnel: [w2546] -> w426
            tunnel: w425 -> [w2546]
            tunnel: [w2541] -> w409
            tunnel: w408 -> [w2541]
            tunnel: [w2540] -> w404
            tunnel: w403 -> [w2539]
            tunnel: w385 -> [w2538]
            tunnel: w383 -> [w2537]
            tunnel: w381 -> [w2536]
            tunnel: w371 -> [w2535]
            tunnel: w527 -> [w2618]
            tunnel: w526 -> [w2617]
            tunnel: w525 -> [w2616]
            tunnel: w524 -> [w2615]
            tunnel: w523 -> [w2614]
            tunnel: w522 -> [w2613]
            tunnel: w521 -> [w2612]
            tunnel: w520 -> [w2611]
            tunnel: w519 -> [w2610]
            tunnel: w518 -> [w2609]
            tunnel: w517 -> [w2608]
            tunnel: w516 -> [w2605]
            tunnel: [w2618] -> w509
            tunnel: [w2617] -> w508
            tunnel: [w2616] -> w507
            tunnel: [w2615] -> w506
            tunnel: [w2614] -> w505
            tunnel: [w2613] -> w504
            tunnel: [w2612] -> w503
            tunnel: [w2611] -> w502
            tunnel: [w2610] -> w501
            tunnel: [w2609] -> w500
            tunnel: [w2608] -> w499
            tunnel: [w2605] -> w498
            tunnel: [w2604] -> w497
            tunnel: w476 -> [w2602]
            tunnel: [w2602] -> w474
            tunnel: w458 -> [w2601]
            tunnel: w457 -> [w2600]
            tunnel: [w2595] -> w456
            tunnel: w450 -> [w2594]
            tunnel: w449 -> [w2593]
            tunnel: [w2592] -> w442
            tunnel: w441 -> [w2592]
            tunnel: [w2591] -> w431
            tunnel: w430 -> [w2591]
            tunnel: [w2590] -> w427
            tunnel: w426 -> [w2590]
            tunnel: w409 -> [w2589]
            tunnel: [w2589] -> w407
            tunnel: [w2588] -> w405
            tunnel: w404 -> [w2588]
            tunnel: [w2631] -> w544
            tunnel: [w2632] -> w547
            tunnel: [w2633] -> w550
            tunnel: [w2634] -> w571
            tunnel: [w2635] -> w573
            tunnel: [w2636] -> w597
            tunnel: [w2637] -> w599
            tunnel: [w2638] -> w601
            tunnel: [w2639] -> w603
            tunnel: [w2640] -> w605
            tunnel: [w2641] -> w606
            tunnel: w509 -> [w2641]
            tunnel: w508 -> [w2640]
            tunnel: w507 -> [w2639]
            tunnel: w506 -> [w2638]
            tunnel: w505 -> [w2637]
            tunnel: w504 -> [w2636]
            tunnel: w503 -> [w2635]
            tunnel: w502 -> [w2634]
            tunnel: w501 -> [w2633]
            tunnel: w500 -> [w2632]
            tunnel: w499 -> [w2631]
            tunnel: w498 -> [w2627]
            tunnel: w497 -> [w2626]
            tunnel: [w2625] -> w473
            tunnel: w474 -> [w2625]
            tunnel: [w2624] -> w469
            tunnel: w456 -> [w2624]
            tunnel: [w2623] -> w439
            tunnel: w442 -> [w2623]
            tunnel: w431 -> [w2622]
            tunnel: [w2622] -> w428
            tunnel: w427 -> [w2621]
            tunnel: [w2621] -> w422
            tunnel: w407 -> [w2620]
            tunnel: [w2620] -> w406
            tunnel: [w2619] -> w402
            tunnel: w405 -> [w2619]
            frame #0 {
              n84 = Tick Count (ms)() -> (millisecond timer value=w642:u32)
            }
            frame #1 {
              n85 = while {
                tunnel: w683 -> [w696]
                tunnel: [w695] -> w682
                tunnel: [w691] -> w681
                tunnel: w669 -> [w693]
                tunnel: w662 -> [w692]
                tunnel: [w690] -> w664
                tunnel: [w689] -> w663
                tunnel: w658 -> [w688]
                tunnel: w656 -> [w687]
                tunnel: w657 -> [w686]
                stop <- w697 stop-if-true
                n86 = event shown="[2] \"Setpoint  START 2\": Value Change" {
                  selector: _ -> [_ _ _ _ _ _ _ _ _ _ _ _ _ _ _ _ _ _ _ _ _ _ _ _ _]
                  dyn-events: _ -> [_ _ _ _ _ _ _ _ _ _ _ _ _ _ _ _ _ _ _ _ _ _ _ _ _]
                  timeout: 1 -> [_ _ _ _ _ _ _ _ _ _ _ _ _ _ _ _ _ _ _ _ _ _ _ _ _]
                  tunnel: [TRUE ("Set Gauge to Zero") w711 w762 w813 w838 w862 w891 w920 w959 w997 w1055 w1114 w1168 w1222 w1304 w1386 w1460 w1534 w1608 "Set Gauge to Zero" _ _ _ _ "SET"] -> w697
                  tunnel: w696 -> [w704 w710 w757 w810 w832 w860 w888 w916 w954 w996 w1050 w1110 w1166 w1220 w1302 w1384 w1456 w1532 w1606 w1686 w1711 w1722 w1795 w1881 _]
                  tunnel: [w703 w709 w756 w809 w831 w859 w885 w918 w953 w994 w1052 w1112 w1165 w1219 w1301 w1383 w1458 w1531 w1605 w1685 w1710 w1720 w1799 w1879 _] -> w695
                  tunnel: [w702 w708 w755 w808 w830 w858 w884 w917 w952 w995 w1051 w1111 w1164 w1218 w1300 w1382 w1457 w1530 w1604 w1684 w1709 w1721 w1800 w1878 _] -> w691
                  tunnel: w693 -> [_ _ _ _ _ _ _ _ _ _ _ _ _ _ _ _ _ _ _ w1682 _ _ _ _ _]
                  tunnel: w692 -> [w700 w707 w760 w807 w835 w857 w889 w913 w957 w993 w1049 w1109 w1163 w1217 w1297 w1381 w1455 w1529 w1603 w1677 w1703 w1719 w1796 w1880 _]
                  tunnel: [w698 w706 w759 w806 w834 w856 w887 w915 w956 w992 w1054 w1108 w1162 w1216 w1299 w1380 w1454 w1528 w1602 w1676 w1702 w1718 w1798 w1877 _] -> w690
                  tunnel: [w699 w705 w758 w805 w833 w855 w886 w914 w955 w991 w1053 w1107 w1161 w1215 w1298 w1379 w1453 w1527 w1601 w1675 w1701 w1717 w1797 w1876 _] -> w689
                  tunnel: w688 -> [_ _ _ _ _ _ _ _ _ _ _ _ _ _ _ _ _ _ _ _ _ _ _ w1882 _]
                  tunnel: w687 -> [_ _ _ _ _ _ _ _ _ _ _ _ _ _ _ _ _ _ _ _ _ _ _ _ w1889]
                  tunnel: w686 -> [_ _ _ _ _ _ _ _ _ _ _ _ _ _ _ _ _ _ _ _ _ _ _ _ w1888]
                  event Timeout {
                    n87 = event-data() -> ()  [unwired: 1 in, 1 out]
                    n88 = Unbundle(w704) -> ("VISA resource name out"=w703:refnum<visa-resource-name>, "error out"=w702:errorcluster)  [unwired: 2 out]
                    n89 = Unbundle(w700) -> ("VISA resource name out"=w698:refnum<visa-resource-name>, "error out"=w699:errorcluster)  [unwired: 2 out]
                  }
                  event "Setpoint\n START": Value Change {
                    n90 = event-data() -> ()  [unwired: 1 in, 1 out]
                    n91 = stacked-sequence {
                      tunnel: w710 -> [_ w717 _]
                      tunnel: [_ w716 _] -> w708
                      tunnel: [_ w715 _] -> w709
                      frame #0 {
                        n92 = property on="Setpoint\n START" class="Bool"("Blinking"=TRUE) -> ()  [unwired: 2 in, 2 out]
                        n93 = property on="ON" class="Bool (strict)"("Blinking"=FALSE) -> ()  [unwired: 2 in, 2 out]
                      }
                      frame #1 {
                        n94 = for {
                          N: 2 -> [_]
                          tunnel: w717 -> [w721]
                          tunnel: [w720] -> w716
                          tunnel: [w719] -> w715
                          i -> [w723]
                          n95 = flat-sequence {
                            tunnel: [w726] -> w722
                            tunnel: w723 -> [w725]
                            tunnel: [w744] -> w724
                            tunnel: w722 -> [w743]
                            tunnel: w721 -> [w745]
                            tunnel: [w742] -> w720
                            tunnel: [w741] -> w719
                            tunnel: w724 -> [w751]
                            tunnel: w723 -> [w750]
                            frame #0 {
                              n96 = case shown="0, Default" w725 {
                                tunnel: [w735 w737] -> w726
                                frame 0, Default {
                                n97 = Multiply(x=10.0, y="SP 1 input (°C)") -> (x*y=w732:dbl)
                                n98 = local read "RAM"() -> (w730:bool)
                                n99 = Number To Hexadecimal String(1:i16 5 ("width (-)"), 2:w732) -> (0:w734:string)
                                n100 = Select(t="*P012", s=w730, f="*P012") -> (s? t:f=w727:string)
                                n101 = Concatenate Strings(w727, w734) -> (w735:string)
                                }
                                frame 1 {
                                n102 = local read "RAM"() -> (w740:bool)
                                n103 = Select(t="*G01", s=w740, f="*R01") -> (s? t:f=w737:string)
                                }
                              }
                            }
                            frame #1 {
                              n104 = Unbundle(w745) -> ("VISA resource name out"=w746:refnum<visa-resource-name>, "error out"=w748:errorcluster, "Delay (ms)"=w747:u32, "Write/\nRead"=w749:bool)
                              n105 = call "I3252_Comm_Interface.vi"("VISA resource name in"=w746, "error in"=w748, "Delay (ms)"=w747, "Write"=w749, "String to Write"=w743, "Read"=w749) -> ("VISA resource name out"=w741:refnum<visa-resource-name>, "error out"=w742:errorcluster, "Read String"=w744:string)  [unwired: 2 in]
                            }
                            frame #2 {
                              n106 = case shown="0, Default" w750 {
                                tunnel: w751 -> [_ w753]
                                frame 0, Default {
                                }
                                frame 1 {
                                n107 = call "I3252_Edit_Setpoint.vi"("Read String"=w753) -> ("Setpoint is"=→"SP 1 is (°C)":dbl)
                                }
                              }
                            }
                          }
                        }
                      }
                      frame #2 {
                        n108 = property on="Setpoint\n START" class="Bool"("Blinking"=FALSE) -> ()  [unwired: 2 in, 2 out]
                      }
                    }
                    n109 = Unbundle(w707) -> ("VISA resource name out"=w706:refnum<visa-resource-name>, "error out"=w705:errorcluster)  [unwired: 2 out]
                    n110 = Not(x="Setpoint\n START") -> (.not. x?=w711:bool)
                  }
                  event "Setpoint\n START\n2": Value Change {
                    n111 = event-data() -> ()  [unwired: 1 in, 1 out]
                    n112 = stacked-sequence {
                      tunnel: w760 -> [_ w767 _]
                      tunnel: [_ w766 _] -> w758
                      tunnel: [_ w765 _] -> w759
                      frame #0 {
                        n113 = property on="Setpoint\n START\n2" class="Bool"("Blinking"=TRUE) -> ()  [unwired: 2 in, 2 out]
                        n114 = property on="ON 2" class="Bool (strict)"("Blinking"=FALSE) -> ()  [unwired: 2 in, 2 out]
                      }
                      frame #1 {
                        n115 = for {
                          N: 2 -> [_]
                          tunnel: w767 -> [w771]
                          tunnel: [w770] -> w766
                          tunnel: [w769] -> w765
                          i -> [w773]
                          n116 = flat-sequence {
                            tunnel: [w776] -> w772
                            tunnel: w773 -> [w775]
                            tunnel: [w794] -> w774
                            tunnel: w772 -> [w793]
                            tunnel: w771 -> [w795]
                            tunnel: [w792] -> w770
                            tunnel: [w791] -> w769
                            tunnel: w774 -> [w801]
                            tunnel: w773 -> [w800]
                            frame #0 {
                              n117 = case shown="0, Default" w775 {
                                tunnel: [w785 w787] -> w776
                                frame 0, Default {
                                n118 = Multiply(x=10.0, y="SP 2 input (°C)") -> (x*y=w783:dbl)
                                n119 = local read "RAM"() -> (w781:bool)
                                n120 = Number To Hexadecimal String(1:i16 5 ("width (-)"), 2:w783) -> (0:w784:string)
                                n121 = Select(t="*P012", s=w781, f="*P012") -> (s? t:f=w778:string)
                                n122 = Concatenate Strings(w778, w784) -> (w785:string)
                                }
                                frame 1 {
                                n123 = local read "RAM"() -> (w790:bool)
                                n124 = Select(t="*G01", s=w790, f="*R01") -> (s? t:f=w787:string)
                                }
                              }
                            }
                            frame #1 {
                              n125 = Unbundle(w795) -> ("VISA resource name out"=w796:refnum<visa-resource-name>, "error out"=w798:errorcluster, "Delay (ms) 2"=w797:u32, "Write/\nRead \n\n2"=w799:bool)
                              n126 = call "I3252_Comm_Interface.vi"("VISA resource name in"=w796, "error in"=w798, "Delay (ms)"=w797, "Write"=w799, "String to Write"=w793, "Read"=w799) -> ("VISA resource name out"=w791:refnum<visa-resource-name>, "error out"=w792:errorcluster, "Read String"=w794:string)  [unwired: 2 in]
                            }
                            frame #2 {
                              n127 = case shown="1" w800 {
                                tunnel: w801 -> [_ w803]
                                frame 0, Default {
                                }
                                frame 1 {
                                n128 = call "I3252_Edit_Setpoint.vi"("Read String"=w803) -> ("Setpoint is"=→"SP 2 is (°C)":dbl)
                                }
                              }
                            }
                          }
                        }
                      }
                      frame #2 {
                        n129 = property on="Setpoint\n START\n2" class="Bool"("Blinking"=FALSE) -> ()  [unwired: 2 in, 2 out]
                      }
                    }
                    n130 = Not(x="Setpoint\n START\n2") -> (.not. x?=w762:bool)
                    n131 = Unbundle(w757) -> ("VISA resource name out"=w756:refnum<visa-resource-name>, "error out"=w755:errorcluster)  [unwired: 2 out]
                  }
                  event "Standby": Value Change {
                    n132 = event-data() -> ()  [unwired: 1 in, 1 out]
                    n133 = flat-sequence {
                      tunnel: [w821] -> w811
                      tunnel: w811 -> [w825]
                      tunnel: w810 -> [w824]
                      tunnel: [w823] -> w808
                      tunnel: [w822] -> w809
                      frame #0 {
                        n134 = local read "Standby"() -> (w814:bool)
                        n135 = Select(t=TRUE, s=w814, f=FALSE) -> (s? t:f=w817:bool)
                        n136 = property on="Standby" class="Bool (strict)"("Blinking"=w817) -> ()  [unwired: 2 in, 2 out]
                      }
                      frame #1 {
                        n137 = local read "Standby"() -> (w819:bool)
                        n138 = Select(t="*D03", s=w819, f="*E03") -> (s? t:f=w821:string)
                      }
                      frame #2 {
                        n139 = Unbundle(w824) -> ("VISA resource name out"=w826:refnum<visa-resource-name>, "error out"=w828:errorcluster, "Delay (ms)"=w827:u32, "Write/\nRead"=w829:bool)
                        n140 = call "I3252_Comm_Interface.vi"("VISA resource name in"=w826, "error in"=w828, "Delay (ms)"=w827, "Write"=w829, "String to Write"=w825, "Read"=w829) -> ("VISA resource name out"=w822:refnum<visa-resource-name>, "error out"=w823:errorcluster)  [unwired: 2 in, 1 out]
                      }
                    }
                    n141 = Not(x="Standby") -> (.not. x?=w813:bool)
                    n142 = Unbundle(w807) -> ("VISA resource name out"=w806:refnum<visa-resource-name>, "error out"=w805:errorcluster)  [unwired: 2 out]
                  }
                  event "Standby\n2": Value Change {
                    n143 = event-data() -> ()  [unwired: 1 in, 1 out]
                    n144 = flat-sequence {
                      tunnel: [w846] -> w837
                      tunnel: w837 -> [w850]
                      tunnel: w835 -> [w849]
                      tunnel: [w848] -> w833
                      tunnel: [w847] -> w834
                      frame #0 {
                        n145 = local read "Standby\n2"() -> (w840:bool)
                        n146 = Select(t=TRUE, s=w840, f=FALSE) -> (s? t:f=w839:bool)
                        n147 = property on="Standby\n2" class="Bool (strict)"("Blinking"=w839) -> ()  [unwired: 2 in, 2 out]
                      }
                      frame #1 {
                        n148 = local read "Standby\n2"() -> (w844:bool)
                        n149 = Select(t="*D03", s=w844, f="*E03") -> (s? t:f=w846:string)
                      }
                      frame #2 {
                        n150 = Unbundle(w849) -> ("VISA resource name out"=w851:refnum<visa-resource-name>, "error out"=w853:errorcluster, "Delay (ms) 2"=w852:u32, "Write/\nRead \n\n2"=w854:bool)
                        n151 = call "I3252_Comm_Interface.vi"("VISA resource name in"=w851, "error in"=w853, "Delay (ms)"=w852, "Write"=w854, "String to Write"=w850, "Read"=w854) -> ("VISA resource name out"=w847:refnum<visa-resource-name>, "error out"=w848:errorcluster)  [unwired: 2 in, 1 out]
                      }
                    }
                    n152 = Not(x="Standby\n2") -> (.not. x?=w838:bool)
                    n153 = Unbundle(w832) -> ("VISA resource name out"=w831:refnum<visa-resource-name>, "error out"=w830:errorcluster)  [unwired: 2 out]
                  }
                  event "Set Command": Value Change {
                    n154 = event-data() -> ()  [unwired: 1 in, 1 out]
                    n155 = stacked-sequence {
                      tunnel: w860 -> [_ w867 _]
                      tunnel: [_ w866 _] -> w859
                      tunnel: [_ w865 _] -> w858
                      frame #0 {
                        n156 = property on="Set Command" class="Bool"("Blinking"=TRUE) -> ()  [unwired: 2 in, 2 out]
                        n157 = property on="ON" class="Bool (strict)"("Blinking"=FALSE) -> ()  [unwired: 2 in, 2 out]
                      }
                      frame #1 {
                        n158 = flat-sequence {
                          tunnel: [w872] -> w869
                          tunnel: [w875] -> w868
                          tunnel: w869 -> [w876]
                          tunnel: w867 -> [w877]
                          tunnel: [w874] -> w866
                          tunnel: [w873] -> w865
                          tunnel: w868 -> [w882]
                          frame #0 {
                            n159 = Concatenate Strings("*", "Command input") -> (w872:string)
                          }
                          frame #1 {
                            n160 = Unbundle(w877) -> ("VISA resource name out"=w881:refnum<visa-resource-name>, "error out"=w879:errorcluster, "Delay (ms)"=w880:u32, "Write/\nRead"=w878:bool)
                            n161 = call "I3252_Comm_Interface.vi"("VISA resource name in"=w881, "error in"=w879, "Delay (ms)"=w880, "Write"=w878, "String to Write"=w876, "Read"=w878) -> ("VISA resource name out"=w874:refnum<visa-resource-name>, "error out"=w873:errorcluster, "Read String"=w875:string)  [unwired: 2 in]
                          }
                          frame #2 {
                            "Command output" <- w882
                          }
                        }
                      }
                      frame #2 {
                        n162 = property on="Set Command" class="Bool"("Blinking"=FALSE) -> ()  [unwired: 2 in, 2 out]
                      }
                    }
                    n163 = Not(x="Set Command") -> (.not. x?=w862:bool)
                    n164 = Unbundle(w857) -> ("VISA resource name out"=w856:refnum<visa-resource-name>, "error out"=w855:errorcluster)  [unwired: 2 out]
                  }
                  event "Set Command\n\n 2": Value Change {
                    n165 = event-data() -> ()  [unwired: 1 in, 1 out]
                    n166 = stacked-sequence {
                      tunnel: w889 -> [_ w896 _]
                      tunnel: [_ w895 _] -> w887
                      tunnel: [_ w894 _] -> w886
                      frame #0 {
                        n167 = property on="Set Command\n\n 2" class="Bool"("Blinking"=TRUE) -> ()  [unwired: 2 in, 2 out]
                        n168 = property on="ON 2" class="Bool (strict)"("Blinking"=FALSE) -> ()  [unwired: 2 in, 2 out]
                      }
                      frame #1 {
                        n169 = flat-sequence {
                          tunnel: [w901] -> w898
                          tunnel: [w904] -> w897
                          tunnel: w898 -> [w905]
                          tunnel: w896 -> [w906]
                          tunnel: [w903] -> w895
                          tunnel: [w902] -> w894
                          tunnel: w897 -> [w911]
                          frame #0 {
                            n170 = Concatenate Strings("*", "Command input 2") -> (w901:string)
                          }
                          frame #1 {
                            n171 = Unbundle(w906) -> ("VISA resource name out"=w910:refnum<visa-resource-name>, "error out"=w908:errorcluster, "Delay (ms) 2"=w909:u32, "Write/\nRead \n\n2"=w907:bool)
                            n172 = call "I3252_Comm_Interface.vi"("VISA resource name in"=w910, "error in"=w908, "Delay (ms)"=w909, "Write"=w907, "String to Write"=w905, "Read"=w907) -> ("VISA resource name out"=w903:refnum<visa-resource-name>, "error out"=w902:errorcluster, "Read String"=w904:string)  [unwired: 2 in]
                          }
                          frame #2 {
                            "Command output 2" <- w911
                          }
                        }
                      }
                      frame #2 {
                        n173 = property on="Set Command\n\n 2" class="Bool"("Blinking"=FALSE) -> ()  [unwired: 2 in, 2 out]
                      }
                    }
                    n174 = Not(x="Set Command\n\n 2") -> (.not. x?=w891:bool)
                    n175 = Unbundle(w888) -> ("VISA resource name out"=w885:refnum<visa-resource-name>, "error out"=w884:errorcluster)  [unwired: 2 out]
                  }
                  event "Reset\nSTOP": Value Change {
                    n176 = event-data() -> ()  [unwired: 1 in, 1 out]
                    n177 = stacked-sequence {
                      tunnel: [_ w927 _] -> w917
                      tunnel: [_ w926 _] -> w918
                      tunnel: w916 -> [_ w924 _]
                      frame #0 {
                        n178 = property on="Reset\nSTOP" class="Bool"("Blinking"=TRUE) -> ()  [unwired: 2 in, 2 out]
                        n179 = property on="ON" class="Bool (strict)"("Blinking"=FALSE) -> ()  [unwired: 2 in, 2 out]
                      }
                      frame #1 {
                        n180 = for {
                          N: 2 -> [_]
                          tunnel: [w933] -> w927
                          tunnel: [w932] -> w926
                          tunnel: w924 -> [w931]
                          i -> [w929]
                          n181 = flat-sequence {
                            tunnel: w929 -> [w935]
                            tunnel: [w934] -> w930
                            tunnel: [w940] -> w933
                            tunnel: [w941] -> w932
                            tunnel: w931 -> [w942]
                            tunnel: w930 -> [w939]
                            tunnel: [w938] -> w928
                            tunnel: w929 -> [w948]
                            tunnel: w928 -> [w947]
                            frame #0 {
                              n182 = case shown="0, Default" w935 {
                                tunnel: ["*Z02" "*G01"] -> w934
                                frame 0, Default {
                                }
                                frame 1 {
                                }
                              }
                            }
                            frame #1 {
                              n183 = Unbundle(w942) -> ("VISA resource name out"=w943:refnum<visa-resource-name>, "error out"=w945:errorcluster, "Delay (ms)"=w944:u32, "Write/\nRead"=w946:bool)
                              n184 = call "I3252_Comm_Interface.vi"("VISA resource name in"=w943, "error in"=w945, "Delay (ms)"=w944, "Write"=w946, "String to Write"=w939, "Read"=w946) -> ("VISA resource name out"=w941:refnum<visa-resource-name>, "error out"=w940:errorcluster, "Read String"=w938:string)  [unwired: 2 in]
                            }
                            frame #2 {
                              n185 = case shown="0, Default" w948 {
                                tunnel: w947 -> [_ w950]
                                frame 0, Default {
                                }
                                frame 1 {
                                n186 = call "I3252_Edit_Setpoint.vi"("Read String"=w950) -> ("Setpoint is"=w949:dbl)
                                n187 = local write "SP 1 is (°C)"(w949) -> ()
                                }
                              }
                            }
                          }
                        }
                        n188 = Wait (ms)(milliseconds to wait=u32 4000) -> ()  [unwired: 1 out]
                      }
                      frame #2 {
                        n189 = property on="Reset\nSTOP" class="Bool"("Blinking"=FALSE) -> ()  [unwired: 2 in, 2 out]
                      }
                    }
                    n190 = Not(x="Reset\nSTOP") -> (.not. x?=w920:bool)
                    n191 = Unbundle(w913) -> ("VISA resource name out"=w915:refnum<visa-resource-name>, "error out"=w914:errorcluster)  [unwired: 2 out]
                  }
                  event "Reset\nSTOP 2": Value Change {
                    n192 = event-data() -> ()  [unwired: 1 in, 1 out]
                    n193 = stacked-sequence {
                      tunnel: [_ w966 _] -> w955
                      tunnel: [_ w965 _] -> w956
                      tunnel: w957 -> [_ w963 _]
                      frame #0 {
                        n194 = property on="Reset\nSTOP 2" class="Bool"("Blinking"=TRUE) -> ()  [unwired: 2 in, 2 out]
                        n195 = property on="ON 2" class="Bool (strict)"("Blinking"=FALSE) -> ()  [unwired: 2 in, 2 out]
                      }
                      frame #1 {
                        n196 = for {
                          N: 2 -> [_]
                          tunnel: [w972] -> w966
                          tunnel: [w971] -> w965
                          tunnel: w963 -> [w970]
                          i -> [w968]
                          n197 = flat-sequence {
                            tunnel: w968 -> [w974]
                            tunnel: [w973] -> w969
                            tunnel: [w979] -> w972
                            tunnel: [w980] -> w971
                            tunnel: w970 -> [w981]
                            tunnel: w969 -> [w978]
                            tunnel: [w977] -> w967
                            tunnel: w968 -> [w987]
                            tunnel: w967 -> [w986]
                            frame #0 {
                              n198 = case shown="0, Default" w974 {
                                tunnel: ["*Z02" "*G01"] -> w973
                                frame 0, Default {
                                }
                                frame 1 {
                                }
                              }
                            }
                            frame #1 {
                              n199 = Unbundle(w981) -> ("VISA resource name out"=w982:refnum<visa-resource-name>, "error out"=w984:errorcluster, "Delay (ms) 2"=w983:u32, "Write/\nRead \n\n2"=w985:bool)
                              n200 = call "I3252_Comm_Interface.vi"("VISA resource name in"=w982, "error in"=w984, "Delay (ms)"=w983, "Write"=w985, "String to Write"=w978, "Read"=w985) -> ("VISA resource name out"=w980:refnum<visa-resource-name>, "error out"=w979:errorcluster, "Read String"=w977:string)  [unwired: 2 in]
                            }
                            frame #2 {
                              n201 = case shown="1" w987 {
                                tunnel: w986 -> [_ w989]
                                frame 0, Default {
                                }
                                frame 1 {
                                n202 = call "I3252_Edit_Setpoint.vi"("Read String"=w989) -> ("Setpoint is"=w988:dbl)
                                n203 = local write "SP 2 is (°C)"(w988) -> ()
                                }
                              }
                            }
                          }
                        }
                        n204 = Wait (ms)(milliseconds to wait=u32 4000) -> ()  [unwired: 1 out]
                      }
                      frame #2 {
                        n205 = property on="Reset\nSTOP 2" class="Bool"("Blinking"=FALSE) -> ()  [unwired: 2 in, 2 out]
                      }
                    }
                    n206 = Not(x="Reset\nSTOP 2") -> (.not. x?=w959:bool)
                    n207 = Unbundle(w954) -> ("VISA resource name out"=w953:refnum<visa-resource-name>, "error out"=w952:errorcluster)  [unwired: 2 out]
                  }
                  event "Auto Tune": Value Change {
                    n208 = event-data() -> ()  [unwired: 1 in, 1 out]
                    n209 = stacked-sequence {
                      tunnel: w996 -> [_ w1003 w1048]
                      tunnel: [_ w1002 _] -> w995
                      tunnel: [_ w1001 _] -> w994
                      frame #0 {
                        n210 = property on="Auto Tune" class="Bool"("Blinking"=TRUE) -> ()  [unwired: 2 in, 2 out]
                        n211 = property on="ON" class="Bool (strict)"("Blinking"=FALSE) -> ()  [unwired: 2 in, 2 out]
                      }
                      frame #1 {
                        n212 = for {
                          N: 4 -> [_]
                          tunnel: [w1008] -> w1001
                          tunnel: [w1007] -> w1002
                          tunnel: w1003 -> [w1006]
                          i -> [w1011]
                          n213 = flat-sequence {
                            tunnel: w1011 -> [w1013]
                            tunnel: [w1012] -> w1009
                            tunnel: w1009 -> [w1028]
                            tunnel: [w1027] -> w1010
                            tunnel: [w1030] -> w1008
                            tunnel: [w1029] -> w1007
                            tunnel: w1006 -> [w1026]
                            tunnel: w1011 -> [w1036]
                            tunnel: w1010 -> [w1035]
                            frame #0 {
                              n214 = case shown="0, Default" w1013 {
                                tunnel: ["*V01" w1016 "*W0C35" "*Z02"] -> w1012
                                frame 0, Default {
                                }
                                frame 1 {
                                n215 = local read "(°C)"() -> (w1015:dbl)
                                n216 = Add(x=20.0, y=w1015) -> (x+y=w1022:dbl)
                                n217 = Multiply(x=10.0, y=w1022) -> (x*y=w1019:dbl)
                                n218 = Number To Hexadecimal String(1:i16 5 ("width (-)"), 2:w1019) -> (0:w1018:string)
                                n219 = Concatenate Strings("*W012", w1018) -> (w1016:string)
                                }
                                frame 2 {
                                # "35 hex = \n00110101 bin"
                                }
                                frame 3 {
                                }
                              }
                            }
                            frame #1 {
                              n220 = Unbundle(w1026) -> ("VISA resource name out"=w1034:refnum<visa-resource-name>, "error out"=w1032:errorcluster, "Delay (ms)"=w1033:u32, "Write/\nRead"=w1031:bool)
                              n221 = call "I3252_Comm_Interface.vi"("VISA resource name in"=w1034, "error in"=w1032, "Delay (ms)"=w1033, "Write"=w1031, "String to Write"=w1028, "Read"=w1031) -> ("VISA resource name out"=w1030:refnum<visa-resource-name>, "error out"=w1029:errorcluster, "Read String"=w1027:string)  [unwired: 2 in]
                            }
                            frame #2 {
                              n222 = case shown="0, Default" w1036 {
                                tunnel: w1035 -> [w1038]
                                frame 0, Default {
                                n223 = call <vilib>:"Space Constant.vi"() -> ("String"=w1041:string)
                                n224 = Search/Split String(string=w1038, search string/char (-)=w1041) -> (match + rest of string=w1040:string)  [unwired: 1 in, 2 out]
                                n225 = Fract/Exp String To Number(use system decimal point (T)=FALSE, string=w1040) -> (number=w1037:dbl)  [unwired: 2 in, 1 out]
                                n226 = local write "(°C)"(w1037) -> ()
                                }
                              }
                            }
                          }
                        }
                        n227 = Wait (ms)(milliseconds to wait=u32 45000) -> ()  [unwired: 1 out]
                      }
                      frame #2 {
                        n228 = Unbundle(w1048) -> ("VISA resource name out"=w1047:refnum<visa-resource-name>, "error out"=w1045:errorcluster, "Delay (ms)"=w1046:u32, "Write/\nRead"=w1044:bool)
                        n229 = property on="Auto Tune" class="Bool"("Blinking"=FALSE) -> ()  [unwired: 2 in, 2 out]
                        n230 = call "I3252_Comm_Interface.vi"("VISA resource name in"=w1047, "error in"=w1045, "Delay (ms)"=w1046, "Write"=w1044, "String to Write"="*W01200000", "Read"=w1044) -> ()  [unwired: 2 in, 3 out]
                      }
                    }
                    n231 = Not(x="Auto Tune") -> (.not. x?=w997:bool)
                    n232 = Unbundle(w993) -> ("VISA resource name out"=w992:refnum<visa-resource-name>, "error out"=w991:errorcluster)  [unwired: 2 out]
                  }
                  event "Auto Tune 2": Value Change {
                    n233 = event-data() -> ()  [unwired: 1 in, 1 out]
                    n234 = stacked-sequence {
                      tunnel: w1049 -> [_ w1061 w1106]
                      tunnel: [_ w1060 _] -> w1053
                      tunnel: [_ w1059 _] -> w1054
                      frame #0 {
                        n235 = property on="Auto Tune 2" class="Bool"("Blinking"=TRUE) -> ()  [unwired: 2 in, 2 out]
                        n236 = property on="ON" class="Bool (strict)"("Blinking"=FALSE) -> ()  [unwired: 2 in, 2 out]
                      }
                      frame #1 {
                        n237 = for {
                          N: 4 -> [_]
                          tunnel: [w1066] -> w1059
                          tunnel: [w1065] -> w1060
                          tunnel: w1061 -> [w1064]
                          i -> [w1069]
                          n238 = flat-sequence {
                            tunnel: w1069 -> [w1071]
                            tunnel: [w1070] -> w1067
                            tunnel: w1067 -> [w1086]
                            tunnel: [w1085] -> w1068
                            tunnel: [w1088] -> w1066
                            tunnel: [w1087] -> w1065
                            tunnel: w1064 -> [w1084]
                            tunnel: w1069 -> [w1094]
                            tunnel: w1068 -> [w1093]
                            frame #0 {
                              n239 = case shown="1" w1071 {
                                tunnel: ["*V01" w1074 "*W0C35" "*Z02"] -> w1070
                                frame 0, Default {
                                }
                                frame 1 {
                                n240 = local read "(°C) \n\n2"() -> (w1073:dbl)
                                n241 = Add(x=20.0, y=w1073) -> (x+y=w1080:dbl)
                                n242 = Multiply(x=10.0, y=w1080) -> (x*y=w1077:dbl)
                                n243 = Number To Hexadecimal String(1:i16 5 ("width (-)"), 2:w1077) -> (0:w1076:string)
                                n244 = Concatenate Strings("*W012", w1076) -> (w1074:string)
                                }
                                frame 2 {
                                # "35 hex = \n00110101 bin"
                                }
                                frame 3 {
                                }
                              }
                            }
                            frame #1 {
                              n245 = Unbundle(w1084) -> ("VISA resource name out"=w1092:refnum<visa-resource-name>, "error out"=w1090:errorcluster, "Delay (ms) 2"=w1091:u32, "Write/\nRead \n\n2"=w1089:bool)
                              n246 = call "I3252_Comm_Interface.vi"("VISA resource name in"=w1092, "error in"=w1090, "Delay (ms)"=w1091, "Write"=w1089, "String to Write"=w1086, "Read"=w1089) -> ("VISA resource name out"=w1088:refnum<visa-resource-name>, "error out"=w1087:errorcluster, "Read String"=w1085:string)  [unwired: 2 in]
                            }
                            frame #2 {
                              n247 = case shown="0, Default" w1094 {
                                tunnel: w1093 -> [w1096]
                                frame 0, Default {
                                n248 = call <vilib>:"Space Constant.vi"() -> ("String"=w1099:string)
                                n249 = Search/Split String(string=w1096, search string/char (-)=w1099) -> (match + rest of string=w1098:string)  [unwired: 1 in, 2 out]
                                n250 = Fract/Exp String To Number(use system decimal point (T)=FALSE, string=w1098) -> (number=w1095:dbl)  [unwired: 2 in, 1 out]
                                n251 = local write "(°C) \n\n2"(w1095) -> ()
                                }
                              }
                            }
                          }
                        }
                        n252 = Wait (ms)(milliseconds to wait=u32 45000) -> ()  [unwired: 1 out]
                      }
                      frame #2 {
                        n253 = Unbundle(w1106) -> ("VISA resource name out"=w1105:refnum<visa-resource-name>, "error out"=w1103:errorcluster, "Delay (ms) 2"=w1104:u32, "Write/\nRead \n\n2"=w1102:bool)
                        n254 = property on="Auto Tune 2" class="Bool"("Blinking"=FALSE) -> ()  [unwired: 2 in, 2 out]
                        n255 = call "I3252_Comm_Interface.vi"("VISA resource name in"=w1105, "error in"=w1103, "Delay (ms)"=w1104, "Write"=w1102, "String to Write"="*W01200000", "Read"=w1102) -> ()  [unwired: 2 in, 3 out]
                      }
                    }
                    n256 = Not(x="Auto Tune 2") -> (.not. x?=w1055:bool)
                    n257 = Unbundle(w1050) -> ("VISA resource name out"=w1052:refnum<visa-resource-name>, "error out"=w1051:errorcluster)  [unwired: 2 out]
                  }
                  event "Write LOW/HI": Value Change {
                    n258 = event-data() -> ()  [unwired: 1 in, 1 out]
                    n259 = stacked-sequence {
                      tunnel: [_ w1119 _] -> w1112
                      tunnel: [_ w1118 _] -> w1111
                      tunnel: w1110 -> [_ w1117 _]
                      frame #0 {
                        n260 = property on="Write LOW/HI" class="Bool"("Blinking"=TRUE) -> ()  [unwired: 2 in, 2 out]
                        n261 = property on="ON" class="Bool (strict)"("Blinking"=FALSE) -> ()  [unwired: 2 in, 2 out]
                      }
                      frame #1 {
                        n262 = for {
                          N: 4 -> [_]
                          tunnel: [w1123] -> w1119
                          tunnel: [w1122] -> w1118
                          tunnel: w1117 -> [w1121]
                          i -> [w1125]
                          n263 = flat-sequence {
                            tunnel: w1125 -> [w1127]
                            tunnel: [w1128] -> w1124
                            tunnel: w1124 -> [w1142]
                            tunnel: [w1143] -> w1126
                            tunnel: [w1145] -> w1123
                            tunnel: [w1144] -> w1122
                            tunnel: w1121 -> [w1141]
                            tunnel: w1126 -> [w1151]
                            tunnel: w1125 -> [w1150]
                            frame #0 {
                              n264 = case shown="0, Default" w1127 {
                                tunnel: [w1130 w1136 "*R27" "*R28"] -> w1128
                                frame 0, Default {
                                n265 = Number To Hexadecimal String(1:i16 2 ("width (-)"), 2:"% LOW Sollwert") -> (0:w1131:string)
                                n266 = Concatenate Strings("*W27", w1131) -> (w1130:string)
                                }
                                frame 1 {
                                n267 = Number To Hexadecimal String(1:i16 2 ("width (-)"), 2:"% High Sollwert") -> (0:w1137:string)
                                n268 = Concatenate Strings("*W28", w1137) -> (w1136:string)
                                }
                                frame 2 {
                                }
                                frame 3 {
                                }
                              }
                            }
                            frame #1 {
                              n269 = Unbundle(w1141) -> ("VISA resource name out"=w1149:refnum<visa-resource-name>, "error out"=w1147:errorcluster, "Delay (ms)"=w1148:u32, "Write/\nRead"=w1146:bool)
                              n270 = call "I3252_Comm_Interface.vi"("VISA resource name in"=w1149, "error in"=w1147, "Delay (ms)"=w1148, "Write"=w1146, "String to Write"=w1142, "Read"=w1146) -> ("VISA resource name out"=w1145:refnum<visa-resource-name>, "error out"=w1144:errorcluster, "Read String"=w1143:string)  [unwired: 2 in]
                            }
                            frame #2 {
                              n271 = case shown="0, Default" w1150 {
                                tunnel: w1151 -> [_ w1155 w1159]
                                frame 0, Default {
                                }
                                frame 2 {
                                n272 = String Subset(string=w1155, offset (0)=3) -> (substring=w1153:string)  [unwired: 1 in]
                                n273 = Hexadecimal String To Number(string=w1153) -> (number=→"% LOW Istwert":u32)  [unwired: 2 in, 1 out]
                                }
                                frame 3 {
                                n274 = String Subset(string=w1159, offset (0)=3) -> (substring=w1157:string)  [unwired: 1 in]
                                n275 = Hexadecimal String To Number(string=w1157) -> (number=→"% HIGH Istwert":u32)  [unwired: 2 in, 1 out]
                                }
                              }
                            }
                          }
                        }
                      }
                      frame #2 {
                        n276 = property on="Write LOW/HI" class="Bool"("Blinking"=FALSE) -> ()  [unwired: 2 in, 2 out]
                      }
                    }
                    n277 = Not(x="Write LOW/HI") -> (.not. x?=w1114:bool)
                    n278 = Unbundle(w1109) -> ("VISA resource name out"=w1108:refnum<visa-resource-name>, "error out"=w1107:errorcluster)  [unwired: 2 out]
                  }
                  event "Write LOW/HI 2": Value Change {
                    n279 = event-data() -> ()  [unwired: 1 in, 1 out]
                    n280 = stacked-sequence {
                      tunnel: [_ w1173 _] -> w1162
                      tunnel: [_ w1172 _] -> w1161
                      tunnel: w1163 -> [_ w1171 _]
                      frame #0 {
                        n281 = property on="Write LOW/HI 2" class="Bool"("Blinking"=TRUE) -> ()  [unwired: 2 in, 2 out]
                        n282 = property on="ON 2" class="Bool (strict)"("Blinking"=FALSE) -> ()  [unwired: 2 in, 2 out]
                      }
                      frame #1 {
                        n283 = for {
                          N: 4 -> [_]
                          tunnel: [w1177] -> w1173
                          tunnel: [w1176] -> w1172
                          tunnel: w1171 -> [w1175]
                          i -> [w1179]
                          n284 = flat-sequence {
                            tunnel: w1179 -> [w1181]
                            tunnel: [w1182] -> w1178
                            tunnel: w1178 -> [w1196]
                            tunnel: [w1197] -> w1180
                            tunnel: [w1199] -> w1177
                            tunnel: [w1198] -> w1176
                            tunnel: w1175 -> [w1195]
                            tunnel: w1180 -> [w1205]
                            tunnel: w1179 -> [w1204]
                            frame #0 {
                              n285 = case shown="0, Default" w1181 {
                                tunnel: [w1185 w1190 "*R27" "*R28"] -> w1182
                                frame 0, Default {
                                n286 = Number To Hexadecimal String(1:i16 2 ("width (-)"), 2:"% LOW Sollwert 2") -> (0:w1186:string)
                                n287 = Concatenate Strings("*W27", w1186) -> (w1185:string)
                                }
                                frame 1 {
                                n288 = Number To Hexadecimal String(1:i16 2 ("width (-)"), 2:"% High Sollwert 2") -> (0:w1191:string)
                                n289 = Concatenate Strings("*W28", w1191) -> (w1190:string)
                                }
                                frame 2 {
                                }
                                frame 3 {
                                }
                              }
                            }
                            frame #1 {
                              n290 = Unbundle(w1195) -> ("VISA resource name out"=w1203:refnum<visa-resource-name>, "error out"=w1201:errorcluster, "Delay (ms) 2"=w1202:u32, "Write/\nRead \n\n2"=w1200:bool)
                              n291 = call "I3252_Comm_Interface.vi"("VISA resource name in"=w1203, "error in"=w1201, "Delay (ms)"=w1202, "Write"=w1200, "String to Write"=w1196, "Read"=w1200) -> ("VISA resource name out"=w1199:refnum<visa-resource-name>, "error out"=w1198:errorcluster, "Read String"=w1197:string)  [unwired: 2 in]
                            }
                            frame #2 {
                              n292 = case shown="3" w1204 {
                                tunnel: w1205 -> [_ w1209 w1213]
                                frame 0, Default {
                                }
                                frame 2 {
                                n293 = String Subset(string=w1209, offset (0)=3) -> (substring=w1207:string)  [unwired: 1 in]
                                n294 = Hexadecimal String To Number(string=w1207) -> (number=→"% LOW Istwert 2":u32)  [unwired: 2 in, 1 out]
                                }
                                frame 3 {
                                n295 = String Subset(string=w1213, offset (0)=3) -> (substring=w1211:string)  [unwired: 1 in]
                                n296 = Hexadecimal String To Number(string=w1211) -> (number=→"% HIGH Istwert 2":u32)  [unwired: 2 in, 1 out]
                                }
                              }
                            }
                          }
                        }
                      }
                      frame #2 {
                        n297 = property on="Write LOW/HI 2" class="Bool"("Blinking"=FALSE) -> ()  [unwired: 2 in, 2 out]
                      }
                    }
                    n298 = Not(x="Write LOW/HI 2") -> (.not. x?=w1168:bool)
                    n299 = Unbundle(w1166) -> ("VISA resource name out"=w1165:refnum<visa-resource-name>, "error out"=w1164:errorcluster)  [unwired: 2 out]
                  }
                  event "Set PID": Value Change {
                    n300 = event-data() -> ()  [unwired: 1 in, 1 out]
                    n301 = stacked-sequence {
                      tunnel: w1220 -> [_ w1227 _]
                      tunnel: [_ w1226 _] -> w1219
                      tunnel: [_ w1225 _] -> w1218
                      frame #0 {
                        n302 = property on="Set PID" class="Bool"("Blinking"=TRUE) -> ()  [unwired: 2 in, 2 out]
                        n303 = property on="ON" class="Bool (strict)"("Blinking"=FALSE) -> ()  [unwired: 2 in, 2 out]
                      }
                      frame #1 {
                        n304 = for {
                          N: 6 -> [_]
                          tunnel: w1227 -> [w1231]
                          tunnel: [w1230] -> w1226
                          tunnel: [w1229] -> w1225
                          i -> [w1233]
                          n305 = flat-sequence {
                            tunnel: w1233 -> [w1235]
                            tunnel: [w1236] -> w1232
                            tunnel: w1232 -> [w1277]
                            tunnel: [w1273] -> w1234
                            tunnel: w1231 -> [w1276]
                            tunnel: [w1275] -> w1229
                            tunnel: [w1274] -> w1230
                            tunnel: w1234 -> [w1283]
                            tunnel: w1233 -> [w1282]
                            frame #0 {
                              n306 = case shown="2" w1235 {
                                tunnel: [w1243 w1251 w1259 w1261 w1265 w1269] -> w1236
                                frame 0, Default {
                                n307 = local read "RAM"() -> (w1237:bool)
                                n308 = Number To Hexadecimal String(1:i16 4 ("width (-)"), 2:"P (PB1) Sollwert") -> (0:w1244:string)
                                n309 = Select(t="*P17", s=w1237, f="*W17") -> (s? t:f=w1238:string)
                                n310 = Concatenate Strings(w1238, w1244) -> (w1243:string)
                                }
                                frame 1 {
                                n311 = local read "RAM"() -> (w1245:bool)
                                n312 = Number To Hexadecimal String(1:i16 4 ("width (-)"), 2:"I ( Reset1) Sollwert") -> (0:w1252:string)
                                n313 = Select(t="*P18", s=w1245, f="*W18") -> (s? t:f=w1247:string)
                                n314 = Concatenate Strings(w1247, w1252) -> (w1251:string)
                                }
                                frame 2 {
                                n315 = local read "RAM"() -> (w1254:bool)
                                n316 = Number To Hexadecimal String(1:i16 4 ("width (-)"), 2:"D (Rate) Sollwert") -> (0:w1260:string)
                                n317 = Select(t="*P19", s=w1254, f="*W19") -> (s? t:f=w1255:string)
                                n318 = Concatenate Strings(w1255, w1260) -> (w1259:string)
                                }
                                frame 3 {
                                n319 = local read "RAM"() -> (w1264:bool)
                                n320 = Select(t="*G17", s=w1264, f="*R17") -> (s? t:f=w1261:string)
                                }
                                frame 4 {
                                n321 = local read "RAM"() -> (w1268:bool)
                                n322 = Select(t="*G18", s=w1268, f="*R18") -> (s? t:f=w1265:string)
                                }
                                frame 5 {
                                n323 = local read "RAM"() -> (w1272:bool)
                                n324 = Select(t="*G19", s=w1272, f="*R19") -> (s? t:f=w1269:string)
                                }
                              }
                            }
                            frame #1 {
                              n325 = Unbundle(w1276) -> ("VISA resource name out"=w1281:refnum<visa-resource-name>, "error out"=w1279:errorcluster, "Delay (ms)"=w1280:u32, "Write/\nRead"=w1278:bool)
                              n326 = call "I3252_Comm_Interface.vi"("VISA resource name in"=w1281, "error in"=w1279, "Delay (ms)"=w1280, "Write"=w1278, "String to Write"=w1277, "Read"=w1278) -> ("VISA resource name out"=w1274:refnum<visa-resource-name>, "error out"=w1275:errorcluster, "Read String"=w1273:string)  [unwired: 2 in]
                            }
                            frame #2 {
                              n327 = case shown="4" w1282 {
                                tunnel: w1283 -> [_ w1287 w1291 w1295]
                                frame 0, Default {
                                }
                                frame 3 {
                                n328 = String Subset(string=w1287, offset (0)=3) -> (substring=w1285:string)  [unwired: 1 in]
                                n329 = Hexadecimal String To Number(string=w1285) -> (number=→"P (PB1) Istwert":u32)  [unwired: 2 in, 1 out]
                                }
                                frame 4 {
                                n330 = String Subset(string=w1291, offset (0)=3) -> (substring=w1289:string)  [unwired: 1 in]
                                n331 = Hexadecimal String To Number(string=w1289) -> (number=→"I ( Reset1) Istwert":u32)  [unwired: 2 in, 1 out]
                                }
                                frame 5 {
                                n332 = String Subset(string=w1295, offset (0)=3) -> (substring=w1293:string)  [unwired: 1 in]
                                n333 = Hexadecimal String To Number(string=w1293) -> (number=→"D (Rate) IstWert":u32)  [unwired: 2 in, 1 out]
                                }
                              }
                            }
                          }
                        }
                      }
                      frame #2 {
                        n334 = property on="Set PID" class="Bool"("Blinking"=FALSE) -> ()  [unwired: 2 in, 2 out]
                      }
                    }
                    n335 = Not(x="Set PID") -> (.not. x?=w1222:bool)
                    n336 = Unbundle(w1217) -> ("VISA resource name out"=w1216:refnum<visa-resource-name>, "error out"=w1215:errorcluster)  [unwired: 2 out]
                  }
                  event "Set PID 2": Value Change {
                    n337 = event-data() -> ()  [unwired: 1 in, 1 out]
                    n338 = stacked-sequence {
                      tunnel: w1297 -> [_ w1309 _]
                      tunnel: [_ w1308 _] -> w1299
                      tunnel: [_ w1307 _] -> w1298
                      frame #0 {
                        n339 = property on="Set PID 2" class="Bool"("Blinking"=TRUE) -> ()  [unwired: 2 in, 2 out]
                        n340 = property on="ON 2" class="Bool (strict)"("Blinking"=FALSE) -> ()  [unwired: 2 in, 2 out]
                      }
                      frame #1 {
                        n341 = for {
                          N: 6 -> [_]
                          tunnel: w1309 -> [w1313]
                          tunnel: [w1312] -> w1308
                          tunnel: [w1311] -> w1307
                          i -> [w1315]
                          n342 = flat-sequence {
                            tunnel: w1315 -> [w1317]
                            tunnel: [w1318] -> w1314
                            tunnel: w1314 -> [w1359]
                            tunnel: [w1355] -> w1316
                            tunnel: w1313 -> [w1358]
                            tunnel: [w1357] -> w1311
                            tunnel: [w1356] -> w1312
                            tunnel: w1316 -> [w1365]
                            tunnel: w1315 -> [w1364]
                            frame #0 {
                              n343 = case shown="0, Default" w1317 {
                                tunnel: [w1325 w1333 w1341 w1343 w1347 w1351] -> w1318
                                frame 0, Default {
                                n344 = local read "RAM 2"() -> (w1320:bool)
                                n345 = Number To Hexadecimal String(1:i16 4 ("width (-)"), 2:"P (PB1) Sollwert 2") -> (0:w1326:string)
                                n346 = Select(t="*P17", s=w1320, f="*W17") -> (s? t:f=w1321:string)
                                n347 = Concatenate Strings(w1321, w1326) -> (w1325:string)
                                }
                                frame 1 {
                                n348 = local read "RAM 2"() -> (w1328:bool)
                                n349 = Number To Hexadecimal String(1:i16 4 ("width (-)"), 2:"I ( Reset1) Sollwert 2") -> (0:w1334:string)
                                n350 = Select(t="*P18", s=w1328, f="*W18") -> (s? t:f=w1329:string)
                                n351 = Concatenate Strings(w1329, w1334) -> (w1333:string)
                                }
                                frame 2 {
                                n352 = local read "RAM 2"() -> (w1336:bool)
                                n353 = Number To Hexadecimal String(1:i16 4 ("width (-)"), 2:"D (Rate) Sollwert 2") -> (0:w1342:string)
                                n354 = Select(t="*P19", s=w1336, f="*W19") -> (s? t:f=w1337:string)
                                n355 = Concatenate Strings(w1337, w1342) -> (w1341:string)
                                }
                                frame 3 {
                                n356 = local read "RAM"() -> (w1346:bool)
                                n357 = Select(t="*G17", s=w1346, f="*R17") -> (s? t:f=w1343:string)
                                }
                                frame 4 {
                                n358 = local read "RAM"() -> (w1350:bool)
                                n359 = Select(t="*G18", s=w1350, f="*R18") -> (s? t:f=w1347:string)
                                }
                                frame 5 {
                                n360 = local read "RAM"() -> (w1354:bool)
                                n361 = Select(t="*G19", s=w1354, f="*R19") -> (s? t:f=w1351:string)
                                }
                              }
                            }
                            frame #1 {
                              n362 = Unbundle(w1358) -> ("VISA resource name out"=w1363:refnum<visa-resource-name>, "error out"=w1361:errorcluster, "Delay (ms) 2"=w1362:u32, "Write/\nRead \n\n2"=w1360:bool)
                              n363 = call "I3252_Comm_Interface.vi"("VISA resource name in"=w1363, "error in"=w1361, "Delay (ms)"=w1362, "Write"=w1360, "String to Write"=w1359, "Read"=w1360) -> ("VISA resource name out"=w1356:refnum<visa-resource-name>, "error out"=w1357:errorcluster, "Read String"=w1355:string)  [unwired: 2 in]
                            }
                            frame #2 {
                              n364 = case shown="0, Default" w1364 {
                                tunnel: w1365 -> [_ w1369 w1373 w1377]
                                frame 0, Default {
                                }
                                frame 3 {
                                n365 = String Subset(string=w1369, offset (0)=3) -> (substring=w1367:string)  [unwired: 1 in]
                                n366 = Hexadecimal String To Number(string=w1367) -> (number=→"P (PB1) Istwert 2":u32)  [unwired: 2 in, 1 out]
                                }
                                frame 4 {
                                n367 = String Subset(string=w1373, offset (0)=3) -> (substring=w1371:string)  [unwired: 1 in]
                                n368 = Hexadecimal String To Number(string=w1371) -> (number=→"I ( Reset1) Istwert 2":u32)  [unwired: 2 in, 1 out]
                                }
                                frame 5 {
                                n369 = String Subset(string=w1377, offset (0)=3) -> (substring=w1375:string)  [unwired: 1 in]
                                n370 = Hexadecimal String To Number(string=w1375) -> (number=→"D (Rate) IstWert 2":u32)  [unwired: 2 in, 1 out]
                                }
                              }
                            }
                          }
                        }
                      }
                      frame #2 {
                        n371 = property on="Set PID 2" class="Bool"("Blinking"=FALSE) -> ()  [unwired: 2 in, 2 out]
                      }
                    }
                    n372 = Not(x="Set PID 2") -> (.not. x?=w1304:bool)
                    n373 = Unbundle(w1302) -> ("VISA resource name out"=w1301:refnum<visa-resource-name>, "error out"=w1300:errorcluster)  [unwired: 2 out]
                  }
                  event "Get Values": Value Change {
                    n374 = event-data() -> ()  [unwired: 1 in, 1 out]
                    n375 = stacked-sequence {
                      tunnel: w1384 -> [_ w1391 _]
                      tunnel: [_ w1390 _] -> w1383
                      tunnel: [_ w1389 _] -> w1382
                      frame #0 {
                        n376 = property on="Get Values" class="Bool"("Blinking"=TRUE) -> ()  [unwired: 2 in, 2 out]
                        n377 = property on="ON" class="Bool (strict)"("Blinking"=FALSE) -> ()  [unwired: 2 in, 2 out]
                      }
                      frame #1 {
                        n378 = for {
                          N: 6 -> [_]
                          tunnel: w1391 -> [w1395]
                          tunnel: [w1394] -> w1390
                          tunnel: [w1393] -> w1389
                          i -> [w1397]
                          n379 = flat-sequence {
                            tunnel: w1397 -> [w1399]
                            tunnel: [w1400] -> w1396
                            tunnel: w1396 -> [w1422]
                            tunnel: [w1423] -> w1398
                            tunnel: w1395 -> [w1421]
                            tunnel: [w1420] -> w1393
                            tunnel: [w1419] -> w1394
                            tunnel: w1398 -> [w1429]
                            tunnel: w1397 -> [w1428]
                            frame #0 {
                              n380 = case shown="0, Default" w1399 {
                                tunnel: [w1403 w1407 w1411 "*R27" "*R28" w1417] -> w1400
                                frame 0, Default {
                                n381 = local read "RAM"() -> (w1404:bool)
                                n382 = Select(t="*G17", s=w1404, f="*R17") -> (s? t:f=w1403:string)
                                }
                                frame 1 {
                                n383 = local read "RAM"() -> (w1408:bool)
                                n384 = Select(t="*G18", s=w1408, f="*R18") -> (s? t:f=w1407:string)
                                }
                                frame 2 {
                                n385 = local read "RAM"() -> (w1412:bool)
                                n386 = Select(t="*G19", s=w1412, f="*R19") -> (s? t:f=w1411:string)
                                }
                                frame 3 {
                                }
                                frame 4 {
                                }
                                frame 5 {
                                n387 = local read "RAM"() -> (w1418:bool)
                                n388 = Select(t="*G01", s=w1418, f="*R01") -> (s? t:f=w1417:string)
                                }
                              }
                            }
                            frame #1 {
                              n389 = Unbundle(w1421) -> ("VISA resource name out"=w1427:refnum<visa-resource-name>, "error out"=w1425:errorcluster, "Delay (ms)"=w1426:u32, "Write/\nRead"=w1424:bool)
                              n390 = call "I3252_Comm_Interface.vi"("VISA resource name in"=w1427, "error in"=w1425, "Delay (ms)"=w1426, "Write"=w1424, "String to Write"=w1422, "Read"=w1424) -> ("VISA resource name out"=w1419:refnum<visa-resource-name>, "error out"=w1420:errorcluster, "Read String"=w1423:string)  [unwired: 2 in]
                            }
                            frame #2 {
                              n391 = case shown="1" w1428 {
                                tunnel: w1429 -> [w1431 w1435 w1439 w1443 w1447 w1451]
                                frame 0, Default {
                                n392 = String Subset(string=w1431, offset (0)=3) -> (substring=w1432:string)  [unwired: 1 in]
                                n393 = Hexadecimal String To Number(string=w1432) -> (number=w1430:u32)  [unwired: 2 in, 1 out]
                                n394 = local write "P (PB1) Sollwert"(w1430) -> ()
                                n395 = local write "P (PB1) Istwert"(w1430) -> ()
                                }
                                frame 1 {
                                n396 = String Subset(string=w1435, offset (0)=3) -> (substring=w1436:string)  [unwired: 1 in]
                                n397 = Hexadecimal String To Number(string=w1436) -> (number=w1434:u32)  [unwired: 2 in, 1 out]
                                n398 = local write "I ( Reset1) Sollwert"(w1434) -> ()
                                n399 = local write "I ( Reset1) Istwert"(w1434) -> ()
                                }
                                frame 2 {
                                n400 = String Subset(string=w1439, offset (0)=3) -> (substring=w1440:string)  [unwired: 1 in]
                                n401 = Hexadecimal String To Number(string=w1440) -> (number=w1438:u32)  [unwired: 2 in, 1 out]
                                n402 = local write "D (Rate) Sollwert"(w1438) -> ()
                                n403 = local write "D (Rate) IstWert"(w1438) -> ()
                                }
                                frame 3 {
                                n404 = String Subset(string=w1443, offset (0)=3) -> (substring=w1444:string)  [unwired: 1 in]
                                n405 = Hexadecimal String To Number(string=w1444) -> (number=w1442:u32)  [unwired: 2 in, 1 out]
                                n406 = local write "% LOW Istwert"(w1442) -> ()
                                n407 = local write "% LOW Sollwert"(w1442) -> ()
                                }
                                frame 4 {
                                n408 = String Subset(string=w1447, offset (0)=3) -> (substring=w1448:string)  [unwired: 1 in]
                                n409 = Hexadecimal String To Number(string=w1448) -> (number=w1446:u32)  [unwired: 2 in, 1 out]
                                n410 = local write "% High Sollwert"(w1446) -> ()
                                n411 = local write "% HIGH Istwert"(w1446) -> ()
                                }
                                frame 5 {
                                n412 = call "I3252_Edit_Setpoint.vi"("Read String"=w1451) -> ("Setpoint is"=w1450:dbl)
                                n413 = local write "SP 1 is (°C)"(w1450) -> ()
                                }
                              }
                            }
                          }
                        }
                      }
                      frame #2 {
                        n414 = property on="Get Values" class="Bool"("Blinking"=FALSE) -> ()  [unwired: 2 in, 2 out]
                      }
                    }
                    n415 = Not(x="Get Values") -> (.not. x?=w1386:bool)
                    n416 = Unbundle(w1381) -> ("VISA resource name out"=w1380:refnum<visa-resource-name>, "error out"=w1379:errorcluster)  [unwired: 2 out]
                  }
                  event "Get Values 2": Value Change {
                    n417 = event-data() -> ()  [unwired: 1 in, 1 out]
                    n418 = stacked-sequence {
                      tunnel: w1455 -> [_ w1465 _]
                      tunnel: [_ w1464 _] -> w1454
                      tunnel: [_ w1463 _] -> w1453
                      frame #0 {
                        n419 = property on="Get Values 2" class="Bool"("Blinking"=TRUE) -> ()  [unwired: 2 in, 2 out]
                        n420 = property on="ON 2" class="Bool (strict)"("Blinking"=FALSE) -> ()  [unwired: 2 in, 2 out]
                      }
                      frame #1 {
                        n421 = for {
                          N: 6 -> [_]
                          tunnel: w1465 -> [w1469]
                          tunnel: [w1468] -> w1464
                          tunnel: [w1467] -> w1463
                          i -> [w1471]
                          n422 = flat-sequence {
                            tunnel: w1471 -> [w1473]
                            tunnel: [w1474] -> w1470
                            tunnel: w1470 -> [w1496]
                            tunnel: [w1497] -> w1472
                            tunnel: w1469 -> [w1495]
                            tunnel: [w1494] -> w1467
                            tunnel: [w1493] -> w1468
                            tunnel: w1472 -> [w1503]
                            tunnel: w1471 -> [w1502]
                            frame #0 {
                              n423 = case shown="1" w1473 {
                                tunnel: [w1477 w1481 w1485 "*R27" "*R28" w1491] -> w1474
                                frame 0, Default {
                                n424 = local read "RAM 2"() -> (w1478:bool)
                                n425 = Select(t="*G17", s=w1478, f="*R17") -> (s? t:f=w1477:string)
                                }
                                frame 1 {
                                n426 = local read "RAM 2"() -> (w1482:bool)
                                n427 = Select(t="*G18", s=w1482, f="*R18") -> (s? t:f=w1481:string)
                                }
                                frame 2 {
                                n428 = local read "RAM 2"() -> (w1486:bool)
                                n429 = Select(t="*G19", s=w1486, f="*R19") -> (s? t:f=w1485:string)
                                }
                                frame 3 {
                                }
                                frame 4 {
                                }
                                frame 5 {
                                n430 = local read "RAM 2"() -> (w1492:bool)
                                n431 = Select(t="*G01", s=w1492, f="*R01") -> (s? t:f=w1491:string)
                                }
                              }
                            }
                            frame #1 {
                              n432 = Unbundle(w1495) -> ("VISA resource name out"=w1501:refnum<visa-resource-name>, "error out"=w1499:errorcluster, "Delay (ms) 2"=w1500:u32, "Write/\nRead \n\n2"=w1498:bool)
                              n433 = call "I3252_Comm_Interface.vi"("VISA resource name in"=w1501, "error in"=w1499, "Delay (ms)"=w1500, "Write"=w1498, "String to Write"=w1496, "Read"=w1498) -> ("VISA resource name out"=w1493:refnum<visa-resource-name>, "error out"=w1494:errorcluster, "Read String"=w1497:string)  [unwired: 2 in]
                            }
                            frame #2 {
                              n434 = case shown="0, Default" w1502 {
                                tunnel: w1503 -> [w1505 w1509 w1513 w1517 w1521 w1525]
                                frame 0, Default {
                                n435 = String Subset(string=w1505, offset (0)=3) -> (substring=w1506:string)  [unwired: 1 in]
                                n436 = Hexadecimal String To Number(string=w1506) -> (number=w1504:u32)  [unwired: 2 in, 1 out]
                                n437 = local write "P (PB1) Sollwert 2"(w1504) -> ()
                                n438 = local write "P (PB1) Istwert 2"(w1504) -> ()
                                }
                                frame 1 {
                                n439 = String Subset(string=w1509, offset (0)=3) -> (substring=w1510:string)  [unwired: 1 in]
                                n440 = Hexadecimal String To Number(string=w1510) -> (number=w1508:u32)  [unwired: 2 in, 1 out]
                                n441 = local write "I ( Reset1) Sollwert 2"(w1508) -> ()
                                n442 = local write "I ( Reset1) Istwert 2"(w1508) -> ()
                                }
                                frame 2 {
                                n443 = String Subset(string=w1513, offset (0)=3) -> (substring=w1514:string)  [unwired: 1 in]
                                n444 = Hexadecimal String To Number(string=w1514) -> (number=w1512:u32)  [unwired: 2 in, 1 out]
                                n445 = local write "D (Rate) Sollwert 2"(w1512) -> ()
                                n446 = local write "D (Rate) IstWert 2"(w1512) -> ()
                                }
                                frame 3 {
                                n447 = String Subset(string=w1517, offset (0)=3) -> (substring=w1518:string)  [unwired: 1 in]
                                n448 = Hexadecimal String To Number(string=w1518) -> (number=w1516:u32)  [unwired: 2 in, 1 out]
                                n449 = local write "% LOW Istwert 2"(w1516) -> ()
                                n450 = local write "% LOW Sollwert 2"(w1516) -> ()
                                }
                                frame 4 {
                                n451 = String Subset(string=w1521, offset (0)=3) -> (substring=w1522:string)  [unwired: 1 in]
                                n452 = Hexadecimal String To Number(string=w1522) -> (number=w1520:u32)  [unwired: 2 in, 1 out]
                                n453 = local write "% High Sollwert 2"(w1520) -> ()
                                n454 = local write "% HIGH Istwert 2"(w1520) -> ()
                                }
                                frame 5 {
                                n455 = call "I3252_Edit_Setpoint.vi"("Read String"=w1525) -> ("Setpoint is"=w1524:dbl)
                                n456 = local write "SP 2 is (°C)"(w1524) -> ()
                                }
                              }
                            }
                          }
                        }
                      }
                      frame #2 {
                        n457 = property on="Get Values 2" class="Bool"("Blinking"=FALSE) -> ()  [unwired: 2 in, 2 out]
                      }
                    }
                    n458 = Not(x="Get Values 2") -> (.not. x?=w1460:bool)
                    n459 = Unbundle(w1456) -> ("VISA resource name out"=w1458:refnum<visa-resource-name>, "error out"=w1457:errorcluster)  [unwired: 2 out]
                  }
                  event "RAM": Value Change {
                    n460 = event-data() -> ()  [unwired: 1 in, 1 out]
                    n461 = stacked-sequence {
                      tunnel: w1532 -> [_ w1539 _]
                      tunnel: [_ w1538 _] -> w1531
                      tunnel: [_ w1537 _] -> w1530
                      frame #0 {
                        n462 = property on="RAM" class="Bool (strict)"("Blinking"=TRUE) -> ()  [unwired: 2 in, 2 out]
                        n463 = property on="ON" class="Bool (strict)"("Blinking"=FALSE) -> ()  [unwired: 2 in, 2 out]
                      }
                      frame #1 {
                        n464 = for {
                          N: 6 -> [_]
                          tunnel: w1539 -> [w1543]
                          tunnel: [w1542] -> w1538
                          tunnel: [w1541] -> w1537
                          i -> [w1545]
                          n465 = flat-sequence {
                            tunnel: w1545 -> [w1547]
                            tunnel: [w1548] -> w1544
                            tunnel: w1544 -> [w1567]
                            tunnel: [w1568] -> w1546
                            tunnel: w1543 -> [w1571]
                            tunnel: [w1570] -> w1541
                            tunnel: [w1569] -> w1542
                            tunnel: w1546 -> [w1577]
                            tunnel: w1545 -> [w1576]
                            frame #0 {
                              n466 = case shown="3" w1547 {
                                tunnel: [w1551 w1555 w1559 "*R27" "*R28" w1565] -> w1548
                                frame 0, Default {
                                n467 = local read "RAM"() -> (w1552:bool)
                                n468 = Select(t="*G17", s=w1552, f="*R17") -> (s? t:f=w1551:string)
                                }
                                frame 1 {
                                n469 = local read "RAM"() -> (w1556:bool)
                                n470 = Select(t="*G18", s=w1556, f="*R18") -> (s? t:f=w1555:string)
                                }
                                frame 2 {
                                n471 = local read "RAM"() -> (w1560:bool)
                                n472 = Select(t="*G19", s=w1560, f="*R19") -> (s? t:f=w1559:string)
                                }
                                frame 3 {
                                }
                                frame 4 {
                                }
                                frame 5 {
                                n473 = local read "RAM"() -> (w1566:bool)
                                n474 = Select(t="*G01", s=w1566, f="*R01") -> (s? t:f=w1565:string)
                                }
                              }
                            }
                            frame #1 {
                              n475 = Unbundle(w1571) -> ("VISA resource name out"=w1575:refnum<visa-resource-name>, "error out"=w1573:errorcluster, "Delay (ms)"=w1574:u32, "Write/\nRead"=w1572:bool)
                              n476 = call "I3252_Comm_Interface.vi"("VISA resource name in"=w1575, "error in"=w1573, "Delay (ms)"=w1574, "Write"=w1572, "String to Write"=w1567, "Read"=w1572) -> ("VISA resource name out"=w1569:refnum<visa-resource-name>, "error out"=w1570:errorcluster, "Read String"=w1568:string)  [unwired: 2 in]
                            }
                            frame #2 {
                              n477 = case shown="5" w1576 {
                                tunnel: w1577 -> [w1579 w1583 w1587 w1591 w1595 w1599]
                                frame 0, Default {
                                n478 = String Subset(string=w1579, offset (0)=3) -> (substring=w1580:string)  [unwired: 1 in]
                                n479 = Hexadecimal String To Number(string=w1580) -> (number=w1578:u32)  [unwired: 2 in, 1 out]
                                n480 = local write "P (PB1) Sollwert"(w1578) -> ()
                                n481 = local write "P (PB1) Istwert"(w1578) -> ()
                                }
                                frame 1 {
                                n482 = String Subset(string=w1583, offset (0)=3) -> (substring=w1584:string)  [unwired: 1 in]
                                n483 = Hexadecimal String To Number(string=w1584) -> (number=w1582:u32)  [unwired: 2 in, 1 out]
                                n484 = local write "I ( Reset1) Sollwert"(w1582) -> ()
                                n485 = local write "I ( Reset1) Istwert"(w1582) -> ()
                                }
                                frame 2 {
                                n486 = String Subset(string=w1587, offset (0)=3) -> (substring=w1588:string)  [unwired: 1 in]
                                n487 = Hexadecimal String To Number(string=w1588) -> (number=w1586:u32)  [unwired: 2 in, 1 out]
                                n488 = local write "D (Rate) IstWert"(w1586) -> ()
                                n489 = local write "D (Rate) Sollwert"(w1586) -> ()
                                }
                                frame 3 {
                                n490 = String Subset(string=w1591, offset (0)=3) -> (substring=w1592:string)  [unwired: 1 in]
                                n491 = Hexadecimal String To Number(string=w1592) -> (number=w1590:u32)  [unwired: 2 in, 1 out]
                                n492 = local write "% LOW Istwert"(w1590) -> ()
                                n493 = local write "% LOW Sollwert"(w1590) -> ()
                                }
                                frame 4 {
                                n494 = String Subset(string=w1595, offset (0)=3) -> (substring=w1596:string)  [unwired: 1 in]
                                n495 = Hexadecimal String To Number(string=w1596) -> (number=w1594:u32)  [unwired: 2 in, 1 out]
                                n496 = local write "% HIGH Istwert"(w1594) -> ()
                                n497 = local write "% High Sollwert"(w1594) -> ()
                                }
                                frame 5 {
                                n498 = call "I3252_Edit_Setpoint.vi"("Read String"=w1599) -> ("Setpoint is"=w1598:dbl)
                                n499 = local write "SP 1 is (°C)"(w1598) -> ()
                                }
                              }
                            }
                          }
                        }
                      }
                      frame #2 {
                        n500 = property on="RAM" class="Bool (strict)"("Blinking"=FALSE) -> ()  [unwired: 2 in, 2 out]
                      }
                    }
                    n501 = Not(x="RAM") -> (.not. x?=w1534:bool)
                    n502 = Unbundle(w1529) -> ("VISA resource name out"=w1528:refnum<visa-resource-name>, "error out"=w1527:errorcluster)  [unwired: 2 out]
                  }
                  event "RAM 2": Value Change {
                    n503 = event-data() -> ()  [unwired: 1 in, 1 out]
                    n504 = stacked-sequence {
                      tunnel: w1603 -> [_ w1613 _]
                      tunnel: [_ w1612 _] -> w1602
                      tunnel: [_ w1611 _] -> w1601
                      frame #0 {
                        n505 = property on="RAM 2" class="Bool (strict)"("Blinking"=TRUE) -> ()  [unwired: 2 in, 2 out]
                        n506 = property on="ON 2" class="Bool (strict)"("Blinking"=FALSE) -> ()  [unwired: 2 in, 2 out]
                      }
                      frame #1 {
                        n507 = for {
                          N: 6 -> [_]
                          tunnel: w1613 -> [w1617]
                          tunnel: [w1616] -> w1612
                          tunnel: [w1615] -> w1611
                          i -> [w1619]
                          n508 = flat-sequence {
                            tunnel: w1619 -> [w1621]
                            tunnel: [w1622] -> w1618
                            tunnel: w1618 -> [w1641]
                            tunnel: [w1642] -> w1620
                            tunnel: w1617 -> [w1645]
                            tunnel: [w1644] -> w1615
                            tunnel: [w1643] -> w1616
                            tunnel: w1620 -> [w1651]
                            tunnel: w1619 -> [w1650]
                            frame #0 {
                              n509 = case shown="5" w1621 {
                                tunnel: [w1625 w1629 w1633 "*R27" "*R28" w1639] -> w1622
                                frame 0, Default {
                                n510 = local read "RAM 2"() -> (w1626:bool)
                                n511 = Select(t="*G17", s=w1626, f="*R17") -> (s? t:f=w1625:string)
                                }
                                frame 1 {
                                n512 = local read "RAM 2"() -> (w1630:bool)
                                n513 = Select(t="*G18", s=w1630, f="*R18") -> (s? t:f=w1629:string)
                                }
                                frame 2 {
                                n514 = local read "RAM 2"() -> (w1634:bool)
                                n515 = Select(t="*G19", s=w1634, f="*R19") -> (s? t:f=w1633:string)
                                }
                                frame 3 {
                                }
                                frame 4 {
                                }
                                frame 5 {
                                n516 = local read "RAM 2"() -> (w1640:bool)
                                n517 = Select(t="*G01", s=w1640, f="*R01") -> (s? t:f=w1639:string)
                                }
                              }
                            }
                            frame #1 {
                              n518 = Unbundle(w1645) -> ("VISA resource name out"=w1649:refnum<visa-resource-name>, "error out"=w1647:errorcluster, "Delay (ms) 2"=w1648:u32, "Write/\nRead \n\n2"=w1646:bool)
                              n519 = call "I3252_Comm_Interface.vi"("VISA resource name in"=w1649, "error in"=w1647, "Delay (ms)"=w1648, "Write"=w1646, "String to Write"=w1641, "Read"=w1646) -> ("VISA resource name out"=w1643:refnum<visa-resource-name>, "error out"=w1644:errorcluster, "Read String"=w1642:string)  [unwired: 2 in]
                            }
                            frame #2 {
                              n520 = case shown="0, Default" w1650 {
                                tunnel: w1651 -> [w1653 w1657 w1661 w1665 w1669 w1673]
                                frame 0, Default {
                                n521 = String Subset(string=w1653, offset (0)=3) -> (substring=w1654:string)  [unwired: 1 in]
                                n522 = Hexadecimal String To Number(string=w1654) -> (number=w1652:u32)  [unwired: 2 in, 1 out]
                                n523 = local write "P (PB1) Sollwert 2"(w1652) -> ()
                                n524 = local write "P (PB1) Istwert 2"(w1652) -> ()
                                }
                                frame 1 {
                                n525 = String Subset(string=w1657, offset (0)=3) -> (substring=w1658:string)  [unwired: 1 in]
                                n526 = Hexadecimal String To Number(string=w1658) -> (number=w1656:u32)  [unwired: 2 in, 1 out]
                                n527 = local write "I ( Reset1) Sollwert 2"(w1656) -> ()
                                n528 = local write "I ( Reset1) Istwert 2"(w1656) -> ()
                                }
                                frame 2 {
                                n529 = String Subset(string=w1661, offset (0)=3) -> (substring=w1662:string)  [unwired: 1 in]
                                n530 = Hexadecimal String To Number(string=w1662) -> (number=w1660:u32)  [unwired: 2 in, 1 out]
                                n531 = local write "D (Rate) IstWert 2"(w1660) -> ()
                                n532 = local write "D (Rate) Sollwert 2"(w1660) -> ()
                                }
                                frame 3 {
                                n533 = String Subset(string=w1665, offset (0)=3) -> (substring=w1666:string)  [unwired: 1 in]
                                n534 = Hexadecimal String To Number(string=w1666) -> (number=w1664:u32)  [unwired: 2 in, 1 out]
                                n535 = local write "% LOW Istwert 2"(w1664) -> ()
                                n536 = local write "% LOW Sollwert 2"(w1664) -> ()
                                }
                                frame 4 {
                                n537 = String Subset(string=w1669, offset (0)=3) -> (substring=w1670:string)  [unwired: 1 in]
                                n538 = Hexadecimal String To Number(string=w1670) -> (number=w1668:u32)  [unwired: 2 in, 1 out]
                                n539 = local write "% HIGH Istwert 2"(w1668) -> ()
                                n540 = local write "% High Sollwert 2"(w1668) -> ()
                                }
                                frame 5 {
                                n541 = call "I3252_Edit_Setpoint.vi"("Read String"=w1673) -> ("Setpoint is"=w1672:dbl)
                                n542 = local write "SP 2 is (°C)"(w1672) -> ()
                                }
                              }
                            }
                          }
                        }
                      }
                      frame #2 {
                        n543 = property on="RAM 2" class="Bool (strict)"("Blinking"=FALSE) -> ()  [unwired: 2 in, 2 out]
                      }
                    }
                    n544 = Not(x="RAM 2") -> (.not. x?=w1608:bool)
                    n545 = Unbundle(w1606) -> ("VISA resource name out"=w1605:refnum<visa-resource-name>, "error out"=w1604:errorcluster)  [unwired: 2 out]
                  }
                  event "Set Gauge to Zero": Value Change {
                    n546 = event-data() -> ()  [unwired: 1 in, 1 out]
                    n547 = flat-sequence {
                      tunnel: w1682 -> [w1687]
                      tunnel: [w1687] -> w1681
                      tunnel: w1681 -> [w1689]
                      tunnel: [w1693] -> w1680
                      tunnel: [w1692] -> w1679
                      tunnel: [w1689] -> w1678
                      tunnel: w1680 -> [w1699]
                      tunnel: w1679 -> [w1698]
                      tunnel: w1678 -> [w1694]
                      frame #0 {
                        n548 = property on="Set Gauge to Zero" class="Bool"("Blinking"=TRUE) -> ()  [unwired: 2 in, 2 out]
                      }
                      frame #1 {
                        w1690 = 0 items=["sensor 1", "sensor 2", "test"] ("Sensor Nr.:")
                        n549 = call "DUAL GAUGE-Get Pressure,Status.vi"("Sensor Nr.:"=w1690, "Referenz in"=w1689) -> ("Pressure"=w1693:dbl)  [unwired: 6 in, 3 out]
                        n550 = call "DUAL GAUGE-Offset display.vi"("W/R"=FALSE, "Referenz in"=w1689) -> ("Sensor 1 Get"=w1692:dbl)  [unwired: 6 in, 3 out]
                      }
                      frame #2 {
                        n551 = Add(x=w1699, y=w1698) -> (x+y=w1695:dbl)
                        n552 = call "DUAL GAUGE-Offset display.vi"("W/R"=TRUE, "Sensor 1 Set"=w1695, "Referenz in"=w1694) -> ("Sensor 1 Get"=→"Current Offset (mbar)":dbl)  [unwired: 5 in, 3 out]
                      }
                      frame #3 {
                        n553 = property on="Set Gauge to Zero" class="Bool"("Blinking"=TRUE) -> ()  [unwired: 2 in, 2 out]
                      }
                    }
                    n554 = Unbundle(w1686) -> ("VISA resource name out"=w1685:refnum<visa-resource-name>, "error out"=w1684:errorcluster)  [unwired: 2 out]
                    n555 = Unbundle(w1677) -> ("VISA resource name out"=w1676:refnum<visa-resource-name>, "error out"=w1675:errorcluster)  [unwired: 2 out]
                  }
                  event "Write to File": Value Change {
                    n556 = event-data() -> ("NewVal"=w1708:bool)  [unwired: 1 in]
                    n557 = Unbundle(w1711) -> ("VISA resource name out"=w1710:refnum<visa-resource-name>, "error out"=w1709:errorcluster)  [unwired: 2 out]
                    n558 = local read "File Path"() -> (w1704:path)
                    n559 = case shown="True" w1708 {
                      tunnel: w1704 -> [_ w1716]
                      tunnel: "User" -> [_ w1715]
                      tunnel: "Sample" -> [_ w1714]
                      tunnel: [path "" ("File Path") w1713] -> w1705
                      frame False {
                      }
                      frame True {
                        n560 = call "Header.vi"("Sample"=w1714, "User"=w1715, "File Path"=w1716) -> ("File Path"=w1713:path)
                      }
                    }
                    n561 = local write "File Path"(w1705) -> ()
                    n562 = Unbundle(w1703) -> ("VISA resource name out"=w1702:refnum<visa-resource-name>, "error out"=w1701:errorcluster)  [unwired: 2 out]
                  }
                  event "Ramp": Value Change {
                    n563 = event-data() -> ()  [unwired: 1 in, 6 out]
                    n564 = stacked-sequence {
                      tunnel: [_ w1727 _ _] -> w1721
                      tunnel: [_ w1726 _ _] -> w1720
                      tunnel: w1722 -> [_ w1725 w1780 _]
                      frame #0 {
                        n565 = property on="Ramp" class="Bool (strict)"("Blinking"=TRUE) -> ()  [unwired: 2 in, 2 out]
                      }
                      frame #1 {
                        n566 = for {
                          N: 6 -> [_]
                          tunnel: [w1733] -> w1727
                          tunnel: [w1732] -> w1726
                          tunnel: w1725 -> [w1731]
                          i -> [w1729]
                          n567 = flat-sequence {
                            tunnel: w1729 -> [w1735]
                            tunnel: [w1734] -> w1730
                            tunnel: [w1772] -> w1733
                            tunnel: [w1773] -> w1732
                            tunnel: w1731 -> [w1774]
                            tunnel: w1730 -> [w1771]
                            frame #0 {
                              n568 = case shown="3" w1735 {
                                tunnel: ["*D03" w1739 w1741 w1755 "*E03" ("string") "*Z02" ("string")] -> w1734
                                frame 0, Default {
                                }
                                frame 1 {
                                n569 = local read "Ramp"() -> (w1737:bool)
                                n570 = Select(t="*W0D78", s=w1737, f="*W0D60") -> (s? t:f=w1739:string)
                                }
                                frame 2 {
                                n571 = local read "Ramp"() -> (w1742:bool)
                                n572 = case shown="True" w1742 {
                                tunnel: ["*W0E0000" ("string") w1748] -> w1741
                                frame False {
                                }
                                frame True {
                                n573 = Quotient & Remainder(x="RAMP", y=60.0) -> (x-y*floor(x/y)=w1744:dbl, floor(x/y)=w1745:dbl)
                                n574 = Multiply(x=w1745, y=100.0) -> (x*y=w1753:dbl)
                                n575 = Add(x=w1753, y=w1744) -> (x+y=w1751:dbl)
                                n576 = Number To Hexadecimal String(1:i16 4 ("width (-)"), 2:w1751) -> (0:w1752:string)
                                n577 = Concatenate Strings("*W0E" ("string"), w1752) -> (w1748:string)
                                }
                                }
                                }
                                frame 3 {
                                n578 = local read "Ramp"() -> (w1756:bool)
                                n579 = case shown="True" w1756 {
                                tunnel: ["*W1E0000" ("string") w1762] -> w1755
                                frame False {
                                }
                                frame True {
                                n580 = Quotient & Remainder(x="SOAK", y=60.0) -> (x-y*floor(x/y)=w1759:dbl, floor(x/y)=w1758:dbl)
                                n581 = Multiply(x=w1758, y=100.0) -> (x*y=w1767:dbl)
                                n582 = Add(x=w1767, y=w1759) -> (x+y=w1765:dbl)
                                n583 = Number To Hexadecimal String(1:i16 4 ("width (-)"), 2:w1765) -> (0:w1766:string)
                                n584 = Concatenate Strings("*W1E" ("string"), w1766) -> (w1762:string)
                                }
                                }
                                }
                                frame 4 {
                                }
                                frame 5 {
                                }
                              }
                            }
                            frame #1 {
                              n585 = Unbundle(w1774) -> ("VISA resource name out"=w1775:refnum<visa-resource-name>, "error out"=w1777:errorcluster, "Delay (ms)"=w1776:u32, "Write/\nRead"=w1778:bool)
                              n586 = call "I3252_Comm_Interface.vi"("VISA resource name in"=w1775, "error in"=w1777, "Delay (ms)"=w1776, "Write"=w1778, "String to Write"=w1771, "Read"=w1778) -> ("VISA resource name out"=w1773:refnum<visa-resource-name>, "error out"=w1772:errorcluster)  [unwired: 2 in, 1 out]
                            }
                          }
                          n587 = Wait (ms)(milliseconds to wait=u32 1000) -> ()  [unwired: 1 out]
                        }
                      }
                      frame #2 {
                        n588 = local read "Ramp"() -> (w1779:bool)
                        n589 = case shown="True" w1779 {
                          tunnel: w1780 -> [_ w1782]
                          frame False {
                          }
                          frame True {
                            n590 = property on="SP 1 input (°C)" class="DigNum (strict)"() -> ("Value"=w1781:dbl)  [unwired: 2 in, 2 out]
                            n591 = Multiply(x=10.0, y=w1781) -> (x*y=w1786:dbl)
                            n592 = Number To Hexadecimal String(1:i16 5 ("width (-)"), 2:w1786) -> (0:w1787:string)
                            n593 = Concatenate Strings("*P012", w1787) -> (w1784:string)
                            n594 = Wait (ms)(milliseconds to wait=u32 4000) -> ()  [unwired: 1 out]
                            n595 = Unbundle(w1782) -> ("VISA resource name out"=w1789:refnum<visa-resource-name>, "error out"=w1791:errorcluster, "Delay (ms)"=w1790:u32, "Write/\nRead"=w1792:bool)
                            n596 = call "I3252_Comm_Interface.vi"("VISA resource name in"=w1789, "error in"=w1791, "Delay (ms)"=w1790, "Write"=w1792, "String to Write"=w1784, "Read"=w1792) -> ()  [unwired: 2 in, 3 out]
                          }
                        }
                      }
                      frame #3 {
                        n597 = property on="Ramp" class="Bool (strict)"("Blinking"=FALSE) -> ()  [unwired: 2 in, 2 out]
                      }
                    }
                    n598 = Unbundle(w1719) -> ("VISA resource name out"=w1718:refnum<visa-resource-name>, "error out"=w1717:errorcluster)  [unwired: 2 out]
                  }
                  event "Ramp 2": Value Change {
                    n599 = event-data() -> ()  [unwired: 1 in, 6 out]
                    n600 = stacked-sequence {
                      tunnel: [_ w1805 _ _] -> w1800
                      tunnel: [_ w1804 _ _] -> w1799
                      tunnel: w1796 -> [_ w1803 w1858 _]
                      frame #0 {
                        n601 = property on="Ramp 2" class="Bool (strict)"("Blinking"=TRUE) -> ()  [unwired: 2 in, 2 out]
                      }
                      frame #1 {
                        n602 = for {
                          N: 6 -> [_]
                          tunnel: [w1811] -> w1805
                          tunnel: [w1810] -> w1804
                          tunnel: w1803 -> [w1809]
                          i -> [w1807]
                          n603 = flat-sequence {
                            tunnel: w1807 -> [w1813]
                            tunnel: [w1812] -> w1808
                            tunnel: [w1850] -> w1811
                            tunnel: [w1851] -> w1810
                            tunnel: w1809 -> [w1852]
                            tunnel: w1808 -> [w1849]
                            frame #0 {
                              n604 = case shown="2" w1813 {
                                tunnel: ["*D03" w1817 w1819 w1833 "*E03" ("string") "*Z02" ("string")] -> w1812
                                frame 0, Default {
                                }
                                frame 1 {
                                n605 = local read "Ramp 2"() -> (w1815:bool)
                                n606 = Select(t="*W0D78", s=w1815, f="*W0D60") -> (s? t:f=w1817:string)
                                }
                                frame 2 {
                                n607 = local read "Ramp 2"() -> (w1820:bool)
                                n608 = case shown="True" w1820 {
                                tunnel: ["*W0E0000" ("string") w1826] -> w1819
                                frame False {
                                }
                                frame True {
                                n609 = Quotient & Remainder(x="RAMP\n\n 2", y=60.0) -> (x-y*floor(x/y)=w1822:dbl, floor(x/y)=w1823:dbl)
                                n610 = Multiply(x=w1823, y=100.0) -> (x*y=w1831:dbl)
                                n611 = Add(x=w1831, y=w1822) -> (x+y=w1829:dbl)
                                n612 = Number To Hexadecimal String(1:i16 4 ("width (-)"), 2:w1829) -> (0:w1830:string)
                                n613 = Concatenate Strings("*W0E" ("string"), w1830) -> (w1826:string)
                                }
                                }
                                }
                                frame 3 {
                                n614 = local read "Ramp 2"() -> (w1834:bool)
                                n615 = case shown="True" w1834 {
                                tunnel: ["*W1E0000" ("string") w1840] -> w1833
                                frame False {
                                }
                                frame True {
                                n616 = Quotient & Remainder(x="SOAK \n\n2", y=60.0) -> (x-y*floor(x/y)=w1837:dbl, floor(x/y)=w1836:dbl)
                                n617 = Multiply(x=w1836, y=100.0) -> (x*y=w1845:dbl)
                                n618 = Add(x=w1845, y=w1837) -> (x+y=w1843:dbl)
                                n619 = Number To Hexadecimal String(1:i16 4 ("width (-)"), 2:w1843) -> (0:w1844:string)
                                n620 = Concatenate Strings("*W1E" ("string"), w1844) -> (w1840:string)
                                }
                                }
                                }
                                frame 4 {
                                }
                                frame 5 {
                                }
                              }
                            }
                            frame #1 {
                              n621 = Unbundle(w1852) -> ("VISA resource name out"=w1853:refnum<visa-resource-name>, "error out"=w1855:errorcluster, "Delay (ms) 2"=w1854:u32, "Write/\nRead \n\n2"=w1856:bool)
                              n622 = call "I3252_Comm_Interface.vi"("VISA resource name in"=w1853, "error in"=w1855, "Delay (ms)"=w1854, "Write"=w1856, "String to Write"=w1849, "Read"=w1856) -> ("VISA resource name out"=w1851:refnum<visa-resource-name>, "error out"=w1850:errorcluster)  [unwired: 2 in, 1 out]
                            }
                          }
                          n623 = Wait (ms)(milliseconds to wait=u32 1000) -> ()  [unwired: 1 out]
                        }
                      }
                      frame #2 {
                        n624 = local read "Ramp 2"() -> (w1857:bool)
                        n625 = case shown="True" w1857 {
                          tunnel: w1858 -> [_ w1860]
                          frame False {
                          }
                          frame True {
                            n626 = property on="SP 1 input (°C)" class="DigNum (strict)"() -> ("Value"=w1859:dbl)  [unwired: 2 in, 2 out]
                            n627 = Multiply(x=10.0, y=w1859) -> (x*y=w1864:dbl)
                            n628 = Number To Hexadecimal String(1:i16 5 ("width (-)"), 2:w1864) -> (0:w1865:string)
                            n629 = Concatenate Strings("*P012", w1865) -> (w1862:string)
                            n630 = Wait (ms)(milliseconds to wait=u32 4000) -> ()  [unwired: 1 out]
                            n631 = Unbundle(w1860) -> ("VISA resource name out"=w1867:refnum<visa-resource-name>, "error out"=w1869:errorcluster, "Delay (ms) 2"=w1868:u32, "Write/\nRead \n\n2"=w1870:bool)
                            n632 = call "I3252_Comm_Interface.vi"("VISA resource name in"=w1867, "error in"=w1869, "Delay (ms)"=w1868, "Write"=w1870, "String to Write"=w1862, "Read"=w1870) -> ()  [unwired: 2 in, 3 out]
                          }
                        }
                      }
                      frame #3 {
                        n633 = property on="Ramp 2" class="Bool (strict)"("Blinking"=FALSE) -> ()  [unwired: 2 in, 2 out]
                      }
                    }
                    n634 = Unbundle(w1795) -> ("VISA resource name out"=w1798:refnum<visa-resource-name>, "error out"=w1797:errorcluster)  [unwired: 2 out]
                  }
                  event "Emissivity\n(eg: 0500)": Value Change {
                    n635 = event-data() -> ()  [unwired: 1 in, 6 out]
                    n636 = Number To Decimal String(number="Emissivity\n(eg: 0500)", width (-)=i16 4) -> (decimal integer string=w1874:string)
                    n637 = Concatenate Strings("em" ("string"), w1874, "\\n" ("string")) -> (w1885:string)
                    n638 = VISA Write(VISA resource name=w1882, write buffer=w1885) -> ()  [unwired: 1 in, 3 out]
                    n639 = Unbundle(w1881) -> ("VISA resource name out"=w1879:refnum<visa-resource-name>, "error out"=w1878:errorcluster)  [unwired: 2 out]
                    n640 = Unbundle(w1880) -> ("VISA resource name out"=w1877:refnum<visa-resource-name>, "error out"=w1876:errorcluster)  [unwired: 2 out]
                  }
                  event "OUTPUT": Value Change {
                    n641 = event-data() -> ()  [unwired: 1 in, 6 out]
                    n642 = case shown="False" "OUTPUT" {
                      tunnel: w1889 -> [w1891 w1894]
                      tunnel: w1888 -> [w1890 w1893]
                      frame False {
                        n643 = VISA Write(VISA resource name=w1891, write buffer=" :OUTP OFF;" ("string"), error in (no error)=w1890) -> ()  [unwired: 3 out]
                      }
                      frame True {
                        n644 = case shown="\"2\", Default" "Unit" {
                          tunnel: [1e-09 ("y") 1e-06 ("y") 0.001 ("y")] -> w1902
                          frame "2", Default {
                          }
                          frame "1" {
                          }
                          frame "0" {
                          }
                        }
                        n645 = case shown="\"1\", Default" "Unit   2" {
                          tunnel: [0.001 ("y") 1.0 ("y")] -> w1898
                          frame "1", Default {
                          }
                          frame "0" {
                          }
                        }
                        n646 = Multiply(x="Source \nCurrent", y=w1902) -> (x*y=w1905:dbl)
                        n647 = Multiply(x="Voltage\nCompl.", y=w1898) -> (x*y=w1896:dbl)
                        n648 = Number To Exponential String(number=w1905, 1:FALSE ("use system decimal point (T)")) -> (E-format string=w1907:string)  [unwired: 2 in]
                        n649 = Concatenate Strings(":SOUR:CURR " ("string"), w1907) -> (w1913:string)
                        n650 = Number To Exponential String(number=w1896, 1:FALSE ("use system decimal point (T)")) -> (E-format string=w1900:string)  [unwired: 2 in]
                        n651 = Concatenate Strings(" ;:VOLT:PROT " ("string"), w1900) -> (w1912:string)
                        n652 = Concatenate Strings(":SYST:RSEN ON;:SOUR:CURR:RANG:AUTO 1 ;:SOUR:FUNC CURR ;" ("write buffer"), w1913, w1912, " ;:OUTP ON" ("string"), "\r") -> (w1911:string)
                        n653 = VISA Write(VISA resource name=w1894, write buffer=w1911, error in (no error)=w1893) -> ()  [unwired: 3 out]
                      }
                    }
                  }
                }
              }
              n654 = Bundle(cluster=w683, "VISA resource name out"=w682, "error out"=w681) -> (w680:T9)  [unwired: 2 in]
              n655 = Bundle(cluster=w662, "VISA resource name out"=w664, "error out"=w663) -> (w661:T10)  [unwired: 2 in]
            }
            frame #2 {
            }
            frame #3 {
              (unwired) "Daniel Schuster (geb. 20.03.1988)"
              n656 = node-c288(w1946) -> (w2010:T4)  [unwired: 2 in]
              n657 = node-c288(w2016) -> (w2019:T4)  [unwired: 2 in]
              n658 = node-c288(w2006) -> (w2008:T4)  [unwired: 2 in]
              n659 = node-c288(w2015) -> (w2023:T4)  [unwired: 2 in]
              n660 = property on="OUTPUT" class="Bool (strict)"() -> ("Value"=w1959:bool)  [unwired: 2 in, 2 out]
              n661 = timed-sequence {
                timing: w2010 -> [_]
                timing-out: [_] -> w2009
                tunnel: w1986 -> [w2164]
                tunnel: w1985 -> [w2160]
                tunnel: [w2163] -> w1982
                tunnel: w1981 -> [w2162]
                tunnel: w1980 -> [w2161]
                tunnel: [w2159] -> w1979
                tunnel: [w2158] -> w1978
                tunnel: [w2157] -> w1976
                tunnel: w1955 -> [w2156]
                tunnel: w1954 -> [w2155]
                tunnel: [w2154] -> w1953
                tunnel: [w2153] -> w1952
                n662 = timed-flat-sequence {
                  tunnel: w2164 -> [w2178]
                  tunnel: [w2177] -> w2163
                  tunnel: w2162 -> [w2176]
                  tunnel: w2161 -> [w2175]
                  tunnel: w2160 -> [w2174]
                  tunnel: [w2172] -> w2159
                  tunnel: [w2171] -> w2158
                  tunnel: [w2170] -> w2157
                  tunnel: w2156 -> [w2168]
                  tunnel: w2155 -> [w2167]
                  tunnel: [w2166] -> w2154
                  tunnel: [w2165] -> w2153
                  n663 = node-c288() -> ()  [unwired: 1 in, 1 out]
                  n664 = case shown="True" "ON (TPG 2)" {
                    tunnel: w2174 -> [w2206 w2212]
                    tunnel: w2175 -> [w2205 w2211]
                    tunnel: [w2204 w2210] -> w2171
                    tunnel: [w2203 w2209] -> w2170
                    frame False {
                      w2207 = 0.0 ("Pressure")
                      n665 = property on="ON (TPG 2)" class="Bool (strict)"("Blinking"=FALSE) -> ()  [unwired: 2 in, 2 out]
                      n666 = Bundle("Pressure"=w2207, "Pressure"=w2207) -> (w2204:cluster{"Pressure":dbl, "Pressure":dbl})  [unwired: 1 in]
                      n667 = Bundle("TPG 2 COM"=w2206, "error out"=w2205) -> (w2203:T11)  [unwired: 1 in]
                    }
                    frame True {
                      n668 = stacked-sequence {
                        tunnel: w2212 -> [_ w2225]
                        tunnel: [_ w2221] -> w2210
                        tunnel: [_ w2217] -> w2209
                        tunnel: w2211 -> [_ w2214]
                        frame #0 {
                          n669 = property on="ON (TPG 2)" class="Bool (strict)"("Blinking"=TRUE) -> ()  [unwired: 2 in, 2 out]
                        }
                        frame #1 {
                          n670 = call "PresureGetSubVI.vi"("COM in"=w2225, "Fehler (Eingang)"=w2214) -> ("Status Gauge#1"=→"Status Gauge 2#1":i32, "Status Gauge#2"=→"Status Gauge 2#2":i32, "COM out"=w2218:refnum<visa-resource-name>, "Pressure Gauge#1"=w2219:dbl, "Pressure Gauge#2"=w2222:dbl, "Cluster (Ausgang)"=w2215:errorcluster)  [unwired: 12 in]
                          "Pressure Gauge 2#1" <- w2219
                          "Pressure Gauge 2#2" <- w2222
                          n671 = Bundle("COM out"=w2218, "Cluster (Ausgang)"=w2215) -> (w2217:T12)  [unwired: 1 in]
                          n672 = Unbundle(w2215) -> ("status"=w2216:bool, "code"=w2220:i32)  [unwired: 1 out]
                          n673 = Bundle("status"=w2216, "code"=w2220) -> ()  [unwired: 1 in, 1 out]
                          n674 = Bundle("Pressure Gauge#1"=w2219, "Pressure Gauge#2"=w2222) -> (w2221:T13)  [unwired: 1 in]
                        }
                      }
                    }
                  }
                  n675 = case shown="True" "ON (TPG 1)" {
                    tunnel: w2178 -> [w2229 w2235]
                    tunnel: [w2228 w2234] -> w2177
                    tunnel: w2176 -> [w2227 w2233]
                    tunnel: [w2226 w2232] -> w2172
                    frame False {
                      w2230 = 0.0 ("Pressure")
                      n676 = property on="ON (TPG 1)" class="Bool (strict)"("Blinking"=FALSE) -> ()  [unwired: 2 in, 2 out]
                      n677 = Bundle("Pressure"=w2230, "Pressure"=w2230) -> (w2226:cluster{"Pressure":dbl, "Pressure":dbl})  [unwired: 1 in]
                      n678 = Bundle("TPG 1 COM"=w2229, "error out"=w2227) -> (w2228:T14)  [unwired: 1 in]
                    }
                    frame True {
                      n679 = stacked-sequence {
                        tunnel: w2235 -> [_ w2248]
                        tunnel: [_ w2241] -> w2234
                        tunnel: w2233 -> [_ w2238]
                        tunnel: [_ w2237] -> w2232
                        frame #0 {
                          n680 = property on="ON (TPG 1)" class="Bool (strict)"("Blinking"=TRUE) -> ()  [unwired: 2 in, 2 out]
                        }
                        frame #1 {
                          n681 = call "PresureGetSubVI.vi"("COM in"=w2248, "Fehler (Eingang)"=w2238) -> ("Status Gauge#1"=→"Status Gauge 1#1":i32, "Status Gauge#2"=→"Status Gauge 1#2":i32, "COM out"=w2242:refnum<visa-resource-name>, "Pressure Gauge#1"=w2243:dbl, "Pressure Gauge#2"=w2245:dbl, "Cluster (Ausgang)"=w2239:errorcluster)  [unwired: 12 in]
                          "Pressure Gauge 1#1" <- w2243
                          "Pressure Gauge 1#2" <- w2245
                          n682 = Bundle("COM out"=w2242, "Cluster (Ausgang)"=w2239) -> (w2241:T12)  [unwired: 1 in]
                          n683 = Unbundle(w2239) -> ("status"=w2240:bool, "code"=w2244:i32)  [unwired: 1 out]
                          n684 = Bundle("status"=w2240, "code"=w2244) -> ()  [unwired: 1 in, 1 out]
                          n685 = Bundle("Pressure Gauge#1"=w2243, "Pressure Gauge#2"=w2245) -> (w2237:T13)  [unwired: 1 in]
                        }
                      }
                    }
                  }
                  n686 = case shown="True" "ON (TPG 3)" {
                    tunnel: w2168 -> [w2183 w2189]
                    tunnel: w2167 -> [w2182 w2188]
                    tunnel: [w2181 w2187] -> w2166
                    tunnel: [w2180 w2186] -> w2165
                    frame False {
                      w2184 = 0.0 ("Pressure")
                      n687 = property on="ON (TPG 3)" class="Bool (strict)"("Blinking"=FALSE) -> ()  [unwired: 2 in, 2 out]
                      n688 = Bundle("Pressure"=w2184, "Pressure"=w2184) -> (w2181:cluster{"Pressure":dbl, "Pressure":dbl})  [unwired: 1 in]
                      n689 = Bundle("TPG 2 COM 2"=w2183, "error out"=w2182) -> (w2180:T15)  [unwired: 1 in]
                    }
                    frame True {
                      n690 = stacked-sequence {
                        tunnel: w2189 -> [_ w2202]
                        tunnel: [_ w2198] -> w2187
                        tunnel: [_ w2194] -> w2186
                        tunnel: w2188 -> [_ w2191]
                        frame #0 {
                          n691 = property on="ON (TPG 3)" class="Bool (strict)"("Blinking"=TRUE) -> ()  [unwired: 2 in, 2 out]
                        }
                        frame #1 {
                          n692 = call "PresureGetSubVI.vi"("COM in"=w2202, "Fehler (Eingang)"=w2191) -> ("Status Gauge#1"=→"Status Gauge 2#1 2":i32, "Status Gauge#2"=→"Status Gauge 2#2 2":i32, "COM out"=w2195:refnum<visa-resource-name>, "Pressure Gauge#1"=w2196:dbl, "Pressure Gauge#2"=w2199:dbl, "Cluster (Ausgang)"=w2192:errorcluster)  [unwired: 12 in]
                          "Pressure Gauge 2#1 2" <- w2196
                          "Pressure Gauge 2#2 2" <- w2199
                          n693 = Bundle("COM out"=w2195, "Cluster (Ausgang)"=w2192) -> (w2194:T12)  [unwired: 1 in]
                          n694 = Unbundle(w2192) -> ("status"=w2193:bool, "code"=w2197:i32)  [unwired: 1 out]
                          n695 = Bundle("status"=w2193, "code"=w2197) -> ()  [unwired: 1 in, 1 out]
                          n696 = Bundle("Pressure Gauge#1"=w2196, "Pressure Gauge#2"=w2199) -> (w2198:T13)  [unwired: 1 in]
                        }
                      }
                    }
                  }
                  n697 = node-c288() -> ()  [unwired: 1 in, 1 out]
                }
              }
              n698 = timed-sequence {
                timing: w2019 -> [_]
                timing-out: [_] -> w2018
                tunnel: w2017 -> [w2258]
                tunnel: [w2257] -> w2012
                tunnel: [w2256] -> w2011
                tunnel: [w2255] -> w1999
                n699 = timed-flat-sequence {
                  tunnel: w2258 -> [w2262]
                  tunnel: [w2261] -> w2257
                  tunnel: [w2260] -> w2256
                  tunnel: [w2259] -> w2255
                  n700 = node-c288() -> ()  [unwired: 1 in, 1 out]
                  n701 = case shown="True" "ON" {
                    tunnel: w2262 -> [w2266 w2271]
                    tunnel: [w2265 w2270] -> w2261
                    tunnel: [w2264 w2269] -> w2260
                    tunnel: [_ w2268] -> w2259
                    frame False {
                      n702 = Unbundle(w2266) -> ("VISA resource name out"=w2265:refnum<visa-resource-name>, "error out"=w2264:errorcluster)  [unwired: 2 out]
                      n703 = property on="ON" class="Bool (strict)"("Blinking"=FALSE) -> ()  [unwired: 2 in, 2 out]
                    }
                    frame True {
                      n704 = stacked-sequence {
                        tunnel: w2271 -> [_ w2276]
                        tunnel: [_ w2275] -> w2270
                        tunnel: [_ w2274] -> w2269
                        tunnel: [_ w2273] -> w2268
                        frame #0 {
                          n705 = property on="ON" class="Bool (strict)"("Blinking"=TRUE) -> ()  [unwired: 2 in, 2 out]
                        }
                        frame #1 {
                          n706 = Unbundle(w2276) -> ("VISA resource name out"=w2280:refnum<visa-resource-name>, "error out"=w2278:errorcluster, "Delay (ms)"=w2279:u32, "Write/\nRead"=w2277:bool)
                          n707 = call "I3252_Comm_Interface.vi"("VISA resource name in"=w2280, "error in"=w2278, "Delay (ms)"=w2279, "Write"=w2277, "String to Write"="*V01", "Read"=w2277) -> ("VISA resource name out"=w2275:refnum<visa-resource-name>, "error out"=w2274:errorcluster, "Read String"=w2273:string)  [unwired: 2 in]
                        }
                      }
                    }
                  }
                  n708 = node-c288() -> ()  [unwired: 1 in, 1 out]
                }
              }
              n709 = timed-sequence {
                timing: w2008 -> [_]
                timing-out: [_] -> w2007
                tunnel: w2005 -> [w2119]
                tunnel: w2004 -> [w2118]
                tunnel: [w2117] -> w2002
                tunnel: [w2116] -> w2003
                tunnel: [w2115] -> w2000
                tunnel: [w2114] -> w1948
                n710 = timed-flat-sequence {
                  tunnel: w2119 -> [w2125]
                  tunnel: w2118 -> [w2124]
                  tunnel: [w2123] -> w2117
                  tunnel: [w2122] -> w2116
                  tunnel: [w2121] -> w2115
                  tunnel: [w2120] -> w2114
                  n711 = node-c288() -> ()  [unwired: 1 in, 1 out]
                  n712 = case shown="False" "ON" {
                    tunnel: w2125 -> [w2130 w2137]
                    tunnel: w2124 -> [w2131 w2136]
                    tunnel: [w2130 w2135] -> w2123
                    tunnel: [w2131 w2134] -> w2122
                    tunnel: [0.0 ("Reading") w2133] -> w2121
                    tunnel: ["Parameter" w2132] -> w2120
                    frame False {
                      n713 = property on="ON" class="Bool (strict)"("Blinking"=FALSE) -> ()  [unwired: 2 in, 2 out]
                    }
                    frame True {
                      n714 = stacked-sequence {
                        tunnel: w2137 -> [_ w2144]
                        tunnel: w2136 -> [_ w2143]
                        tunnel: [_ w2142] -> w2135
                        tunnel: [_ w2141] -> w2134
                        tunnel: [_ w2140] -> w2133
                        tunnel: [_ w2139] -> w2132
                        frame #0 {
                          n715 = property on="ON" class="Bool (strict)"("Blinking"=TRUE) -> ()  [unwired: 2 in, 2 out]
                        }
                        frame #1 {
                          n716 = call "VC840_Read.vi"("error in (no error)"=w2143, "VISA resource name"=w2144) -> ("error out"=w2141:errorcluster, "Unit"=w2139:string, "Reading"=w2140:dbl, "VISA resource name out"=w2142:refnum<visa-resource-name>, "Status"=→"Status 2":T2, "Mode"=→"Mode 2":enum16{"?", "Diode", "Beep", "DC", "AC"})  [unwired: 4 out]
                          "Reading 2" <- w2140
                          "Unit 2" <- w2139
                        }
                      }
                    }
                  }
                  n717 = node-c288() -> ()  [unwired: 1 in, 1 out]
                }
              }
              n718 = timed-sequence {
                timing: w2023 -> [_]
                timing-out: [_] -> w2022
                tunnel: w2021 -> [w2293]
                tunnel: w2020 -> [w2292]
                tunnel: [w2291] -> w2014
                tunnel: [w2290] -> w2013
                tunnel: [w2289] -> w2001
                tunnel: [w2288] -> w1949
                n719 = timed-flat-sequence {
                  tunnel: w2293 -> [w2299]
                  tunnel: w2292 -> [w2298]
                  tunnel: [w2297] -> w2291
                  tunnel: [w2296] -> w2290
                  tunnel: [w2295] -> w2289
                  tunnel: [w2294] -> w2288
                  n720 = node-c288() -> ()  [unwired: 1 in, 1 out]
                  n721 = case shown="False" "ON" {
                    tunnel: w2299 -> [w2304 w2311]
                    tunnel: w2298 -> [w2305 w2310]
                    tunnel: [w2304 w2309] -> w2297
                    tunnel: [w2305 w2308] -> w2296
                    tunnel: [0.0 ("Reading") w2307] -> w2295
                    tunnel: ["Parameter" w2306] -> w2294
                    frame False {
                      n722 = property on="ON" class="Bool (strict)"("Blinking"=FALSE) -> ()  [unwired: 2 in, 2 out]
                    }
                    frame True {
                      n723 = stacked-sequence {
                        tunnel: w2311 -> [_ w2318]
                        tunnel: w2310 -> [_ w2317]
                        tunnel: [_ w2316] -> w2309
                        tunnel: [_ w2315] -> w2308
                        tunnel: [_ w2314] -> w2307
                        tunnel: [_ w2313] -> w2306
                        frame #0 {
                          n724 = property on="ON" class="Bool (strict)"("Blinking"=TRUE) -> ()  [unwired: 2 in, 2 out]
                        }
                        frame #1 {
                          n725 = call "VC840_Read.vi"("error in (no error)"=w2317, "VISA resource name"=w2318) -> ("error out"=w2315:errorcluster, "Unit"=w2313:string, "Reading"=w2314:dbl, "VISA resource name out"=w2316:refnum<visa-resource-name>, "Status"=→"Status 1":T2, "Mode"=→"Mode 1":enum16{"?", "Diode", "Beep", "DC", "AC"})  [unwired: 4 out]
                          "Reading 1" <- w2314
                          "Unit 1" <- w2313
                        }
                      }
                    }
                  }
                  n726 = node-c288() -> ()  [unwired: 1 in, 1 out]
                }
              }
              n727 = case shown="True" w1959 {
                tunnel: [0.0 w2030] -> w1956
                tunnel: [0.0 w2029] -> w1957
                tunnel: [0.0 w2028] -> w1958
                tunnel: w1960 -> [_ w2027]
                frame False {
                }
                frame True {
                  n728 = flat-sequence {
                    tunnel: [w2055] -> w2051
                    tunnel: w2050 -> [w2054]
                    frame #0 {
                      n729 = Wait (ms)(milliseconds to wait=u32 300) -> ()  [unwired: 1 out]
                    }
                    frame #1 {
                      n730 = property class="Instr"(reference=w2054) -> ("Bytes at Port"=w2055:u32)  [unwired: 1 in, 2 out]
                    }
                  }
                  n731 = VISA Write(VISA resource name=w2027, write buffer=":MEAS:VOLT?;") -> (VISA resource name out=w2050:refnum<visa-resource-name>)  [unwired: 1 in, 2 out]
                  n732 = VISA Read(VISA resource name=w2050, byte count=w2051) -> (read buffer=w2044:string)  [unwired: 1 in, 3 out]
                  "read buffer" <- w2044
                  n733 = String Subset(string=w2044, offset (0)=2) -> (substring=w2043:string)  [unwired: 1 in]
                  n734 = Match Pattern(string=w2043, regular expression=",", offset (0)=1) -> (before substring=w2041:string, after substring=w2045:string)  [unwired: 2 out]
                  "Voltage  (V)\n 2" <- w2041
                  n735 = Fract/Exp String To Number(use system decimal point (T)=FALSE, string=w2041, offset=0) -> (number=w2028:dbl)  [unwired: 1 in, 1 out]
                  n736 = Match Pattern(string=w2045, regular expression=",", offset (0)=1) -> (before substring=w2040:string)  [unwired: 3 out]
                  "Current (A) \n\n3" <- w2040
                  n737 = Fract/Exp String To Number(use system decimal point (T)=FALSE, string=w2040, offset=0) -> (number=w2029:dbl)  [unwired: 1 in, 1 out]
                  n738 = Divide(x=w2028, y=w2029) -> (x/y=w2035:dbl)
                  n739 = Compound Arithmetic op=MULTIPLY(w2035, "Thickness", 4.523 ("value"), "4PP Const", 1e-07 ("value")) -> (w2030:dbl)
                  "Resistivity\n 2" <- w2030
                }
              }
              n740 = Tick Count (ms)() -> (millisecond timer value=w1987:u32)
              n741 = case shown="True" "Pyrometer" {
                tunnel: [0 w2061] -> w1961
                tunnel: w1965 -> [w2057 w2060]
                tunnel: w1964 -> [_ w2059]
                tunnel: [w2057 w2058] -> w1963
                frame False {
                }
                frame True {
                  n742 = flat-sequence {
                    tunnel: [w2070] -> w2065
                    tunnel: [w2069] -> w2064
                    tunnel: w2060 -> [w2068]
                    tunnel: w2059 -> [w2066]
                    tunnel: w2065 -> [w2073]
                    tunnel: w2064 -> [w2072]
                    tunnel: [w2073] -> w2063
                    tunnel: [w2072] -> w2062
                    tunnel: w2063 -> [w2080]
                    tunnel: w2062 -> [w2079]
                    tunnel: [w2077] -> _
                    tunnel: [w2074] -> w2061
                    tunnel: [w2076] -> w2058
                    frame #0 {
                      n743 = VISA Write(VISA resource name=w2068, write buffer="00ms\n" ("string"), error in (no error)=w2066) -> (VISA resource name out=w2070:refnum<visa-resource-name>, error out=w2069:errorcluster)  [unwired: 1 out]
                    }
                    frame #1 {
                      n744 = Wait (ms)(milliseconds to wait=u32 500 ("wait")) -> ()  [unwired: 1 out]
                    }
                    frame #2 {
                      n745 = property class="Instr"(reference=w2080, error in=w2079) -> (reference out=w2081:refnum<visa-resource-name>, error out=w2078:errorcluster, "Bytes at Port"=w2082:u32)
                      n746 = VISA Read(VISA resource name=w2081, byte count=w2082, error in (no error)=w2078) -> (VISA resource name out=w2076:refnum<visa-resource-name>, read buffer=w2075:string, error out=w2077:errorcluster)  [unwired: 1 out]
                      n747 = Fract/Exp String To Number(string=w2075) -> (number=w2074:dbl)  [unwired: 3 in, 1 out]
                      "Pyro Temp" <- w2074
                    }
                  }
                }
              }
              n748 = Subtract(x=w1987, y=w1992) -> (x-y=w1991:u32)
              n749 = Divide(x=w1991, y=u32 1000) -> (x/y=w1989:dbl)
              n750 = node-c288(w2018) -> ()  [unwired: 1 out]
              n751 = node-c288(w2022) -> ()  [unwired: 1 out]
              n752 = node-c288(w2007) -> ()  [unwired: 1 out]
              n753 = node-c288(w1967) -> (w1974:T4)  [unwired: 2 in]
              n754 = To Double Precision Float(number=w1989) -> (double precision float=w1993:dbl)
              "Current Time (s)" <- w1993
              n755 = property on="MM2" class="XYGraph (strict)"("YScale.NameLbl.Text"=w1948) -> ()  [unwired: 2 in, 2 out]
              n756 = property on="MM2" class="DigNum (strict)"("UnitLabel.Text"=w1948) -> ()  [unwired: 2 in, 2 out]
              n757 = property on="MM1" class="XYGraph (strict)"("YScale.NameLbl.Text"=w1949) -> ()  [unwired: 2 in, 2 out]
              n758 = property on="MM1" class="DigNum (strict)"("UnitLabel.Text"=w1949) -> ()  [unwired: 2 in, 2 out]
              n759 = timed-sequence {
                timing: w1974 -> [_]
                timing-out: [_] -> w1973
                tunnel: w1972 -> [w2086]
                tunnel: [w2085] -> w1969
                tunnel: [w2084] -> w1968
                tunnel: [w2083] -> w1971
                n760 = timed-flat-sequence {
                  tunnel: w2086 -> [w2091]
                  tunnel: [w2090] -> w2085
                  tunnel: [w2089] -> w2084
                  tunnel: [w2088] -> w2083
                  n761 = node-c288() -> ()  [unwired: 1 in, 1 out]
                  n762 = case shown="False" "ON 2" {
                    tunnel: w2091 -> [w2094 w2098]
                    tunnel: [w2093 w2097] -> w2090
                    tunnel: [w2092 w2096] -> w2089
                    tunnel: [_ w2095] -> w2088
                    frame False {
                      (unwired) FALSE
                      n763 = Unbundle(w2094) -> ("VISA resource name out"=w2093:refnum<visa-resource-name>, "error out"=w2092:errorcluster)  [unwired: 2 out]
                    }
                    frame True {
                      n764 = stacked-sequence {
                        tunnel: w2098 -> [_ w2102]
                        tunnel: [_ w2101] -> w2097
                        tunnel: [_ w2100] -> w2096
                        tunnel: [_ w2099] -> w2095
                        frame #0 {
                          (unwired) TRUE
                        }
                        frame #1 {
                          n765 = Unbundle(w2102) -> ("VISA resource name out"=w2106:refnum<visa-resource-name>, "error out"=w2104:errorcluster, "Delay (ms) 2"=w2105:u32, "Write/\nRead \n\n2"=w2103:bool)
                          n766 = call "I3252_Comm_Interface.vi"("VISA resource name in"=w2106, "error in"=w2104, "Delay (ms)"=w2105, "Write"=w2103, "String to Write"="*V01", "Read"=w2103) -> ("VISA resource name out"=w2101:refnum<visa-resource-name>, "error out"=w2100:errorcluster, "Read String"=w2099:string)  [unwired: 2 in]
                        }
                      }
                    }
                  }
                  n767 = node-c288() -> ()  [unwired: 1 in, 1 out]
                }
              }
              n768 = node-c288(w2009) -> ()  [unwired: 1 out]
              n769 = Unbundle(w1953) -> ("Pressure Gauge#1"=w1951:dbl, "Pressure Gauge#2"=w1950:dbl)
              "LoadLock" <- w1951
              "VVP2 2" <- w1950
              n770 = Unbundle(w1978) -> ("Pressure Gauge#1"=w1977:dbl, "Pressure Gauge#2"=w1975:dbl)
              "Manipulator" <- w1975
              "Baratron" <- w1977
              n771 = Unbundle(w1979) -> ("Pressure Gauge#1"=w1947:dbl, "Pressure Gauge#2"=w1983:dbl)
              "Main Chamber" <- w1947
              "VVP1" <- w1983
              n772 = node-c288(w1973) -> ()  [unwired: 1 out]
            }
            frame #4 {
              n773 = flat-sequence {
                tunnel: w2360 -> [w2412]
                tunnel: [w2411] -> w2359
                frame #0 {
                  n774 = call <vilib>:"Space Constant.vi"() -> ("String"=w2416:string)
                  n775 = Search/Split String(string=w2412, search string/char (-)=w2416) -> (match + rest of string=w2417:string)  [unwired: 1 in, 2 out]
                  n776 = Fract/Exp String To Number(use system decimal point (T)=FALSE, string=w2417) -> (number=w2414:dbl)  [unwired: 2 in, 1 out]
                  n777 = Equal To 0?(x=w2414) -> (x = 0?=w2415:bool)
                  n778 = feedback #1() -> (w2413:dbl)  [unwired: 1 in]
                  n779 = Select(t=w2413, s=w2415, f=w2414) -> (s? t:f=w2411:dbl)
                  n780 = feedback-in #1(w2411) -> ()
                }
              }
              n781 = Unbundle(w2352) -> (w2351:dbl[], w2350:dbl[], w2349:dbl[], w2348:dbl[], w2346:dbl[], w2345:dbl[])
              n782 = flat-sequence {
                tunnel: w2361 -> [w2404]
                tunnel: [w2403] -> w2358
                frame #0 {
                  n783 = call <vilib>:"Space Constant.vi"() -> ("String"=w2408:string)
                  n784 = Search/Split String(string=w2404, search string/char (-)=w2408) -> (match + rest of string=w2409:string)  [unwired: 1 in, 2 out]
                  n785 = Fract/Exp String To Number(use system decimal point (T)=FALSE, string=w2409) -> (number=w2406:dbl)  [unwired: 2 in, 1 out]
                  n786 = Equal To 0?(x=w2406) -> (x = 0?=w2407:bool)
                  n787 = feedback #2() -> (w2405:dbl)  [unwired: 1 in]
                  n788 = Select(t=w2405, s=w2407, f=w2406) -> (s? t:f=w2403:dbl)
                  n789 = feedback-in #2(w2403) -> ()
                }
              }
              n790 = Greater?(x=w2338, y="Pressure Limit (mbar)") -> (0:w2393:bool)
              n791 = Build Array(w2337, w2336, w2335, w2334, w2333, w2332) -> (w2331:dbl[])
              n792 = case shown="False" w2393 {
                frame False {
                  w2419 = T8."Enabled" ("Disabled")
                  n793 = property on="Standby" class="Bool (strict)"("DisabledEnum"=w2419) -> ()  [unwired: 2 in, 2 out]
                  n794 = property on="Standby\n2" class="Bool (strict)"("DisabledEnum"=w2419) -> ()  [unwired: 2 in, 2 out]
                }
                frame True {
                  w2421 = T8."Disabled" ("Disabled")
                  w2420 = TRUE ("Standby")
                  n795 = property on="Standby" class="Bool (strict)"("Val(Sgnl)"=w2420, "DisabledEnum"=w2421) -> ()  [unwired: 2 in, 2 out]
                  n796 = property on="Standby\n2" class="Bool (strict)"("Val(Sgnl)"=w2420, "DisabledEnum"=w2421) -> ()  [unwired: 2 in, 2 out]
                }
              }
              n797 = call "Resistivity_Calculation.vi"("Reading 1 (V)"=w2386, "Constant"="4PP constant", "Thickness (nm)"="Thickness (nm)", "Reading 2 (A)"=w2392) -> ("Resivtivity (Ohm*cm)"=w2380:dbl, "Current"=w2328:dbl, "Voltage"=w2329:dbl)
              "Resistivity\n (Ohm*cm)" <- w2380
              "MM1" <- w2329
              "MM2" <- w2328
              n798 = Build Array (concatenate)(w2351, w2337) -> (w2357:dbl[])
              n799 = Build Array (concatenate)(w2350, w2336) -> (w2356:dbl[])
              n800 = Build Array (concatenate)(w2349, w2335) -> (w2355:dbl[])
              n801 = Build Array (concatenate)(w2348, w2334) -> (w2354:dbl[])
              n802 = Build Array (concatenate)(w2346, w2333) -> (w2344:dbl[])
              n803 = Build Array (concatenate)(w2345, w2332) -> (w2343:dbl[])
              n804 = Unbundle(w2368) -> (w2369:dbl[])  [unwired: 3 out]
              n805 = Unbundle(w2368) -> (w2364:dbl[])  [unwired: 3 out]
              n806 = Unbundle(w2368) -> (w2362:dbl[])  [unwired: 3 out]
              n807 = Unbundle(w2368) -> (w2363:dbl[])  [unwired: 3 out]
              n808 = Build Array (concatenate)(w2369, w2330) -> (w2370:dbl[])
              n809 = Build Array (concatenate)(w2364, w2342) -> (w2367:dbl[])
              n810 = Build Array (concatenate)(w2362, w2340) -> (w2365:dbl[])
              n811 = Build Array (concatenate)(w2363, w2341) -> (w2366:dbl[])
              n812 = Build Array (concatenate)(w2387, w2329) -> (w2385:dbl[])
              n813 = Build Array (concatenate)(w2384, w2328) -> (w2382:dbl[])
              n814 = Build Array (concatenate)(w2383, w2380) -> (w2381:dbl[])
              n815 = Bundle(w2357, w2356, w2355, w2354, w2344, w2343) -> (w2353:T3)  [unwired: 1 in]
              n816 = Build Array (concatenate)(w2389, w2359) -> (w2379:dbl[])
              n817 = Build Array(w2329, w2328) -> (w2327:dbl[])
              n818 = Build Array (concatenate)(w2390, w2391) -> (w2388:dbl[])
              n819 = Build Array (concatenate)(w2374, w2358) -> (w2375:dbl[])
              n820 = Build Array(w2342, w2341, w2340) -> (w2339:dbl[])
              "(°C)" <- w2359
              "(°C) \n\n2" <- w2358
            }
            frame #5 {
              # "MainChamber\nLoadlock\nVVP1\nVVP2\nManipulator"
              n821 = Bundle(w2470, w2494) -> (w2461:cluster{dbl[], dbl[]})  [unwired: 1 in]
              n822 = Bundle(w2470, w2493) -> (w2457:cluster{dbl[], dbl[]})  [unwired: 1 in]
              n823 = Bundle(w2470, w2492) -> (w2462:cluster{dbl[], dbl[]})  [unwired: 1 in]
              n824 = Bundle(w2470, w2491) -> (w2453:cluster{dbl[], dbl[]})  [unwired: 1 in]
              n825 = Bundle(w2470, w2472) -> (w2459:cluster{dbl[], dbl[]})  [unwired: 1 in]
              n826 = Bundle(w2470, w2471) -> (w2455:cluster{dbl[], dbl[]})  [unwired: 1 in]
              n827 = Bundle(w2470, w2478) -> (w2451:cluster{dbl[], dbl[]})  [unwired: 1 in]
              n828 = Bundle(w2470, w2474) -> (w2427:cluster{dbl[], dbl[]})  [unwired: 1 in]
              n829 = Bundle(w2470, w2496) -> (w2439:cluster{dbl[], dbl[]})  [unwired: 1 in]
              n830 = Bundle(w2470, w2497) -> (w2437:cluster{dbl[], dbl[]})  [unwired: 1 in]
              n831 = Bundle(w2470, w2498) -> (w2433:cluster{dbl[], dbl[]})  [unwired: 1 in]
              n832 = property on="Pyrometer" class="Bool (strict)"() -> ("Value"=w2449:bool)  [unwired: 2 in, 2 out]
              n833 = Bundle(w2470, w2487) -> (w2425:cluster{dbl[], dbl[]})  [unwired: 1 in]
              n834 = case shown="False" w2449 {
                tunnel: w2451 -> [_ w2521]
                tunnel: [cluster{dbl[], dbl[]} {[], []} w2521] -> w2450
                frame False {
                }
                frame True {
                }
              }
              "Pyrometer Temperature °C" <- w2450
              n835 = property on="ON" class="Bool (strict)"() -> ("Value"=w2435:bool)  [unwired: 2 in, 2 out]
              n836 = property on="ON" class="Bool (strict)"() -> ("Value"=w2434:bool)  [unwired: 2 in, 2 out]
              n837 = case shown="False" "Temprature1" {
                tunnel: w2427 -> [_ w2509]
                tunnel: [cluster{dbl[], dbl[]} {[], []} w2509] -> w2426
                frame False {
                }
                frame True {
                }
              }
              n838 = case shown="False" "Temperature2" {
                tunnel: w2425 -> [_ w2507]
                tunnel: [cluster{dbl[], dbl[]} {[], []} w2507] -> w2424
                frame False {
                }
                frame True {
                }
              }
              n839 = Bundle(w2470, w2477) -> (w2445:cluster{dbl[], dbl[]})  [unwired: 1 in]
              n840 = Bundle(w2474, w2475) -> (w2442:cluster{dbl[], dbl[]})  [unwired: 1 in]
              n841 = Bundle(w2470, w2476) -> (w2444:cluster{dbl[], dbl[]})  [unwired: 1 in]
              n842 = Bundle(w2470, w2475) -> (w2443:cluster{dbl[], dbl[]})  [unwired: 1 in]
              n843 = property on="OUTPUT" class="Bool (strict)"() -> ("Value"=w2441:bool)  [unwired: 2 in, 2 out]
              n844 = case shown="False" w2434 {
                tunnel: w2437 -> [_ w2512]
                tunnel: [w2510 w2512] -> w2436
                tunnel: w2433 -> [_ w2511]
                tunnel: [w2510 w2511] -> w2432
                frame False {
                  w2510 = cluster{dbl[], dbl[]} {[], []}
                }
                frame True {
                }
              }
              "Resistivity" <- w2432
              "MM2" <- w2436
              n845 = case shown="False" w2435 {
                tunnel: w2439 -> [_ w2514]
                tunnel: [cluster{dbl[], dbl[]} {[], []} w2514] -> w2438
                frame False {
                }
                frame True {
                }
              }
              "MM1" <- w2438
              n846 = Build Array (concatenate)(w2482, w2481, w2480, w2431, w2430, w2429, w2428) -> (w2505:dbl[])
              "appended array" <- w2505
              n847 = property on="Transf" class="Bool (strict)"() -> ("Value"=w2468:bool)  [unwired: 2 in, 2 out]
              n848 = property on="Main" class="Bool (strict)"() -> ("Value"=w2469:bool)  [unwired: 2 in, 2 out]
              n849 = property on="VVP2" class="Bool (strict)"() -> ("Value"=w2465:bool)  [unwired: 2 in, 2 out]
              n850 = property on="Manip" class="Bool (strict)"() -> ("Value"=w2466:bool)  [unwired: 2 in, 2 out]
              n851 = property on="VVP1" class="Bool (strict)"() -> ("Value"=w2467:bool)  [unwired: 2 in, 2 out]
              n852 = case shown="False" w2441 {
                tunnel: [w2515 w2519] -> w2440
                tunnel: [w2515 w2518] -> w2448
                tunnel: [w2515 w2517] -> w2447
                tunnel: [w2515 w2516] -> w2446
                tunnel: w2445 -> [_ w2519]
                tunnel: w2444 -> [_ w2518]
                tunnel: w2443 -> [_ w2517]
                tunnel: w2442 -> [_ w2516]
                frame False {
                  w2515 = cluster{dbl[], dbl[]} {[], []}
                }
                frame True {
                }
              }
              "Voltage Graph" <- w2440
              "Current Graph" <- w2448
              "Resistivity Graph (Ohm Cm)" <- w2447
              "Resistivity/ Temp Dependency" <- w2446
              n853 = property on="Baratron" class="Bool (strict)"() -> ("Value"=w2464:bool)  [unwired: 2 in, 2 out]
              n854 = Build Array(w2426, w2424) -> (→"TEMPERATURE":cluster{dbl[], dbl[]}[])
              n855 = case shown="False" w2469 {
                tunnel: w2461 -> [_ w2523]
                tunnel: [cluster{dbl[], dbl[]} {[], []} w2523] -> w2460
                frame False {
                }
                frame True {
                }
              }
              n856 = case shown="False" w2468 {
                tunnel: w2459 -> [_ w2525]
                tunnel: [cluster{dbl[], dbl[]} {[], []} w2525] -> w2458
                frame False {
                }
                frame True {
                }
              }
              n857 = case shown="False" w2467 {
                tunnel: w2457 -> [_ w2527]
                tunnel: [cluster{dbl[], dbl[]} {[], []} w2527] -> w2456
                frame False {
                }
                frame True {
                }
              }
              n858 = case shown="False" w2465 {
                tunnel: w2455 -> [_ w2529]
                tunnel: [cluster{dbl[], dbl[]} {[], []} w2529] -> w2454
                frame False {
                }
                frame True {
                }
              }
              n859 = case shown="False" w2466 {
                tunnel: w2453 -> [_ w2533]
                tunnel: [cluster{dbl[], dbl[]} {[], []} w2533] -> w2452
                frame False {
                }
                frame True {
                }
              }
              n860 = case shown="False" w2464 {
                tunnel: w2462 -> [_ w2531]
                tunnel: [cluster{dbl[], dbl[]} {[], []} w2531] -> w2463
                frame False {
                }
                frame True {
                }
              }
              "CMR275 Baratron" <- w2463
              n861 = Build Array(w2460, w2458, w2456, w2454, w2452) -> (→"Pirani (VVP1 Scroll)":cluster{dbl[], dbl[]}[])
            }
            frame #6 {
              n862 = Unbundle(w2554) -> ("COM out"=w2553:refnum<visa-resource-name>, "Cluster (Ausgang)"=w2552:errorcluster)
              n863 = Unbundle(w2535) -> ("Cluster (Ausgang)"=w2534:errorcluster)  [unwired: 1 out]
              n864 = Unbundle(w2551) -> ("COM out"=w2550:refnum<visa-resource-name>, "Cluster (Ausgang)"=w2549:errorcluster)
              n865 = Bundle(w2539, w2538, w2537, w2536) -> (w2540:cluster{dbl[], dbl[], dbl[], dbl[]})  [unwired: 1 in]
              n866 = call "Elapsed Time"("Time Target (s)"="Intervall (s)") -> ("Time has Elapsed"=w2543:bool)  [unwired: 11 in, 7 out]
              n867 = And(x="Write to File", y=w2543) -> (x .and. y?=w2542:bool)
              n868 = case shown="True" w2542 {
                tunnel: [w2573 w2579] -> w2565
                tunnel: "File Path" -> [w2573 w2577]
                tunnel: w2558 -> [_ w2575]
                frame False {
                  n869 = property on="Write to File" class="Bool (strict)"("Blinking"=FALSE) -> ()  [unwired: 2 in, 2 out]
                }
                frame True {
                  n870 = flat-sequence {
                    tunnel: [w2581] -> w2578
                    tunnel: w2577 -> [w2581]
                    tunnel: [w2580] -> w2576
                    tunnel: w2575 -> [w2580]
                    tunnel: [w2586] -> w2579
                    tunnel: w2578 -> [w2585]
                    tunnel: w2576 -> [w2584]
                    frame #0 {
                      n871 = property on="Write to File" class="Bool (strict)"("Blinking"=TRUE) -> ()  [unwired: 2 in, 2 out]
                    }
                    frame #1 {
                      n872 = call-poly <vilib>:"Write To Spreadsheet File.vi"("format (%.3f)"="%g", "append to file? (new file:F)"=TRUE ("transpose? (no:F)"), "1D data"=w2584, "file path (dialog if empty)"=w2585) -> ("new file path (Not A Path if cancelled)"=w2586:path)  [unwired: 4 in]
                    }
                  }
                }
              }
              n873 = Merge Errors(w2569, w2568, w2566, w2552, w2549, w2534) -> (w2567:errorcluster)
              n874 = call <vilib>:"Simple Error Handler.vi"("error in (no error)"=w2567) -> ("error?"=w2555:bool)  [unwired: 4 in, 4 out]
              n875 = local write "File Path"(w2565) -> ()
            }
            frame #7 {
              w2604 = u32 1000 ("y")
              n876 = Tick Count (ms)() -> (millisecond timer value=w2606:u32)
              n877 = Subtract(x=w2606, y=w2605) -> (x-y=w2607:u32)
              n878 = VISA Flush I/O Buffer(VISA resource name=w2601, error in (no error)=w2600) -> (VISA resource name out=w2598:refnum<visa-resource-name>, error out=w2599:errorcluster)  [unwired: 1 in]
              n879 = VISA Flush I/O Buffer(VISA resource name=w2594, error in (no error)=w2593) -> (VISA resource name out=w2597:refnum<visa-resource-name>, error out=w2596:errorcluster)  [unwired: 1 in]
              n880 = Divide(x=w2607, y=w2604) -> (x/y=→"Loop Time (s)":dbl)
              n881 = Bundle("COM out"=w2598, "error out"=w2599, "COM out"=w2597, "error out"=w2596) -> (w2595:T16)  [unwired: 1 in]
            }
            frame #8 {
              n882 = Tick Count (ms)() -> (millisecond timer value=w2629:u32)
              n883 = Subtract(x=w2629, y=w2627) -> (x-y=w2628:u32)
              n884 = Divide(x=w2628, y=w2626) -> (x/y=→"Log Intervall (s)":dbl)
            }
          }
          n885 = Exclusive Or(1:w359, 2:w467) -> (0:w468:bool)
        }
      }
      frame #5 {
        n886 = call "VC840_Close.vi"("error in (no error)"=w2652, "VISA resource name"=w2653) -> ("error out"=w2661:errorcluster)  [unwired: 9 in]
        n887 = call "VC840_Close.vi"("error in (no error)"=w2654, "VISA resource name"=w2655) -> ("error out"=w2659:errorcluster)  [unwired: 9 in]
        n888 = VISA Close(VISA resource name=w2657, error in (no error)=w2656) -> (error out=w2658:errorcluster)
        n889 = VISA Close(VISA resource name=w2645, error in (no error)=w2644) -> (error out=w2643:errorcluster)
        n890 = Unbundle(w2650) -> ("COM out"=w2649:refnum<visa-resource-name>, "error out"=w2648:errorcluster, "COM out"=w2646:refnum<visa-resource-name>, "error out"=w2647:errorcluster)
        n891 = VISA Close(VISA resource name=w2642) -> ()  [unwired: 1 in, 1 out]
        n892 = VISA Close(VISA resource name=w2649, error in (no error)=w2648) -> ()  [unwired: 1 out]
        n893 = VISA Close(VISA resource name=w2646, error in (no error)=w2647) -> ()  [unwired: 1 out]
        n894 = Merge Errors(w2658, w2659, w2661, w2643) -> (w2660:errorcluster)
        n895 = call <vilib>:"Simple Error Handler.vi"("error in (no error)"=w2660) -> ("error?"=w2651:bool)  [unwired: 1 in, 7 out]
        n896 = Stop(stop? (T)=w2651) -> ()
      }
    }
  }
